vi "VIP_Phase_2.vi"() -> ()   [LabVIEW 2024]
uses:
  <vilib>/DAQmx/read.llb/DAQmx Read (Digital 1D Bool 1Chan 1Samp).vi
  <vilib>/Utility/file.llb/Write To Spreadsheet File (DBL).vi
  <vilib>/DAQmx/create/channels.llb/DAQmx Create Channel (DI-Digital Input).vi
  <vilib>/DAQmx/miscellaneous.llb/DAQmx Fill In Error Info.vi
  <vilib>/ptbypt/NI_PtbyPt.lvlib
panel:
  out "4.2":bool
  out "mouse 4.2":cluster{"Y":dbl[], "Y":dbl[]}[](graph)
  out "mouse 4.1":cluster{"Y":dbl[], "Y":dbl[]}[](graph)
  in  "fake 4.2":bool
  in  "fake 4.1":bool
  out "ratio 4.2R":cluster{"Y":dbl[], "Y":dbl[]}[](graph)=[{"Y"=[2.5380001068115234, 12.063000202178955, 24.592000007629395, 36.145999908447266, 48.69600009918213, 58.23899984359741, 67.79099988937378, 81.40899991989136, 91.96199989318848, 99.9980001449585], "Y"=[0.0, 0.0, 0.0, 0.0, 0.0, 0.0, 0.0, 0.0, 0.0, 0.0]}]
  out "ratio 4.1L":cluster{"Y":dbl[], "Y":dbl[]}[](graph)=[{"Y"=[2.5380001068115234, 12.063000202178955, 24.592000007629395, 36.145999908447266, 48.69600009918213, 58.23899984359741, 67.79099988937378, 81.40899991989136, 91.96199989318848, 99.9980001449585], "Y"=[0.0, 0.0, 0.0, 0.0, 0.0, 0.0, 0.0, 0.0, 0.0, 0.0]}]
  out "ratio 4.2R":dbl
  out "ratio 4.1L":dbl
  in  "water dur (ms) 4.2":dbl=11.5
  in  "water port 4.2":tag="Dev1/port2/line0"
  out "Mouse path 4":path=path "C:/Users/Administrator/Documents/LabVIEW Data/a-lick-20140707-145848"
  out "Mouse file 4":string="a-lick-20140707-145848"
  in  "Mouse ID 4":string
  in  "water dur (ms) 4.1":dbl=9.0
  in  "water port 4.1":tag="Dev1/port1/line7"
  in  "free water 4.2":bool
  in  "free water 4.1":bool
  out "4.1":bool
  out "state 4.2":enum16{"waiting", "sound", "ITI"}(ring)=enum."ITI"
  out "state 4.1":enum16{"waiting", "sound", "ITI"}(ring)=enum."ITI"
  out "water # 4.1L":dbl
  out "water # 4.2R":dbl
  out "lick # 4.2R":dbl
  out "lick # 4.1L":dbl
  out "last water 4.2R":dbl
  out "last water 4.1L":dbl
  out "mistake # 4.2R":dbl
  out "mistake # 4.1L":dbl
  out "ratio 3.2R":cluster{"Y":dbl[], "Y":dbl[]}[](graph)=[{"Y"=[2.5380001068115234, 12.063000202178955, 24.592000007629395, 36.145999908447266, 48.69600009918213, 58.23899984359741, 67.79099988937378, 81.40899991989136, 91.96199989318848, 99.9980001449585], "Y"=[0.0, 0.0, 0.0, 0.0, 0.0, 0.0, 0.0, 0.0, 0.0, 0.0]}]
  out "ratio 3.1L":cluster{"Y":dbl[], "Y":dbl[]}[](graph)=[{"Y"=[2.5380001068115234, 12.063000202178955, 24.592000007629395, 36.145999908447266, 48.69600009918213, 58.23899984359741, 67.79099988937378, 81.40899991989136, 91.96199989318848, 99.9980001449585], "Y"=[0.0, 0.0, 0.0, 0.0, 0.0, 0.0, 0.0, 0.0, 0.0, 0.0]}]
  in  "free water 3.2":bool
  in  "free water 3.1":bool
  in  "water dur (ms) 3. 2":dbl=26.0
  in  "water dur (ms) 3.1":dbl=26.0
  out "mouse 3.2":cluster{"Y":dbl[], "Y":dbl[]}[](graph)
  out "mouse 3.1":cluster{"Y":dbl[], "Y":dbl[]}[](graph)
  in  "fake 3.2":bool
  in  "fake 3.1":bool
  out "last water 3.2R":dbl
  out "last water 3.1L":dbl
  out "mistake # 3.2R":dbl
  out "mistake # 3.1L":dbl
  out "water # 3.2R":dbl
  out "water # 3.1L":dbl
  out "lick # 3.2R":dbl
  out "lick # 3.1L":dbl
  out "ratio 3.2R":dbl
  out "ratio 3.1L":dbl
  in  "water port 3.2":tag="Dev1/port1/line6"
  out "3.2":bool
  out "state 3.2":enum16{"waiting", "sound", "ITI"}(ring)=enum."ITI"
  out "state 3.1":enum16{"waiting", "sound", "ITI"}(ring)=enum."ITI"
  out "3.1":bool
  out "Mouse path 3":path=path "C:/Users/Administrator/Documents/LabVIEW Data/a-lick-20140707-145848"
  out "Mouse file 3":string="a-lick-20140707-145848"
  in  "water port 3.1":tag="Dev1/port1/line5"
  in  "Mouse ID 3":string="test_3"
  out "ratio 2.2R":cluster{"Y":dbl[], "Y":dbl[]}[](graph)=[{"Y"=[2.5380001068115234, 12.063000202178955, 24.592000007629395, 36.145999908447266, 48.69600009918213, 58.23899984359741, 67.79099988937378, 81.40899991989136, 91.96199989318848, 99.9980001449585], "Y"=[0.0, 0.0, 0.0, 0.0, 0.0, 0.0, 0.0, 0.0, 0.0, 0.0]}]
  out "ratio 2.1L":cluster{"Y":dbl[], "Y":dbl[]}[](graph)=[{"Y"=[2.5380001068115234, 12.063000202178955, 24.592000007629395, 36.145999908447266, 48.69600009918213, 58.23899984359741, 67.79099988937378, 81.40899991989136, 91.96199989318848, 99.9980001449585], "Y"=[0.0, 0.0, 0.0, 0.0, 0.0, 0.0, 0.0, 0.0, 0.0, 0.0]}]
  out "ratio 1.2R":cluster{"Y":dbl[], "Y":dbl[]}[](graph)=[{"Y"=[2.5380001068115234, 12.063000202178955, 24.592000007629395, 36.145999908447266, 48.69600009918213, 58.23899984359741, 67.79099988937378, 81.40899991989136, 91.96199989318848, 99.9980001449585], "Y"=[0.0, 0.0, 0.0, 0.0, 0.0, 0.0, 0.0, 0.0, 0.0, 0.0]}]
  out "mouse 2.2":cluster{"Y":dbl[], "Y":dbl[]}[](graph)
  out "mouse 2.1":cluster{"Y":dbl[], "Y":dbl[]}[](graph)
  in  "free water 2.2":bool
  in  "free water 2.1":bool
  out "last water 2.2R":dbl
  out "last water 2.1L":dbl
  out "mistake # 2.2R":dbl
  out "mistake # 2.1L":dbl
  out "water # 2.2R":dbl
  out "water # 2.1L":dbl
  out "lick  #  2.2R":dbl
  out "lick  #  2.1L":dbl
  out "2.1":bool
  out "ratio 2.2R":dbl
  out "ratio 2.1L":dbl
  out "2.2":bool
  in  "fake 2.2":bool
  in  "fake 2.1":bool
  out "Mouse path 2":path=path "C:/Users/Administrator/Documents/LabVIEW Data/a-lick-20140707-145848"
  out "Mouse file 2":string="a-lick-20140707-145848"
  in  "Mouse ID 2":string="test_2"
  in  "water dur (ms) 2.2":dbl=26.5
  in  "water dur (ms) 2.1":dbl=35.5
  in  "water port 2.2":tag="Dev1/port1/line4"
  in  "water port 2.1":tag="Dev1/port1/line3"
  out "state 2.2":enum16{"waiting", "sound", "ITI"}(ring)=enum."ITI"
  out "state 2.1":enum16{"waiting", "sound", "ITI"}(ring)=enum."ITI"
  in  "sound port 2":tag="Dev1/ao1"
  out "time (s)":dbl=103.38100004196167
  out "mistake # 1.2R":dbl
  out "mistake # 1.1L":dbl
  in  "water dur (ms) 1.1":dbl=33.0
  in  "water port 1.1":tag="Dev1/port1/line1"
  in  "water dur (ms) 1.2":dbl=25.0
  in  "water port 1.2":tag="Dev1/port1/line2"
  out "1.1":bool
  out "1.2":bool
  out "state 1.2":enum16{"waiting", "sound", "ITI"}(ring)=enum."ITI"
  out "lick # 1.2R":dbl
  out "water # 1.2R":dbl
  in  "fake 1.2":bool
  in  "free water 1.2":bool
  out "mouse 1.2":cluster{"Y":dbl[], "Y":dbl[]}[](graph)
  out "ratio 1.2R":dbl
  out "last water 1.2R":dbl
  out "ratio 1.1L":dbl
  out "ratio 1.1L":cluster{"Y":dbl[], "Y":dbl[]}[](graph)=[{"Y"=[2.5380001068115234, 12.063000202178955, 24.592000007629395, 36.145999908447266, 48.69600009918213, 58.23899984359741, 67.79099988937378, 81.40899991989136, 91.96199989318848, 99.9980001449585], "Y"=[0.0, 0.0, 0.0, 0.0, 0.0, 0.0, 0.0, 0.0, 0.0, 0.0]}]
  in  "free water 1.1":bool
  out "Right Speaker":dbl=5.0
  out "Left Speaker":dbl=5.0
  in  "sound file 2":path=path "C:/Users/cvm-gritton-lab/Documents/Lab View Programs/Lab View Programs/LabVIEW VIs/Tones/New_Phase_2_Sounds/200k_target2.wav"
  in  "ITI max (ms)":dbl=7000.0
  in  "ITI min (ms)":dbl=5000.0
  in  "reaction dur (ms)":dbl=1750.0
  in  "sound dur (ms)":dbl=3000.0
  in  "sound file 1":path=path "C:/Users/cvm-gritton-lab/Documents/Lab View Programs/Lab View Programs/LabVIEW VIs/Tones/New_Phase_2_Sounds/200k_target1.wav"
  in  "sound port 1":tag="Dev1/ao0"
  out "trial state":T1(ring)=enum."ITI"
  out "trial #":dbl=10.0
  out "current sound":dbl=1.0
  out "next sound":dbl[](array[numeric])
  out "Mouse path 1":path=path "C:/Users/Administrator/Documents/LabVIEW Data/a-lick-20140707-145848"
  in  "fake 1.1":bool
  out "mouse 1.1":cluster{"Y":dbl[], "Y":dbl[]}[](graph)
  out "ITI (s)":dbl=6.5
  out "last water 1.1L":dbl
  out "state 1.1":enum16{"waiting", "sound", "ITI"}(ring)=enum."ITI"
  out "water # 1.1L":dbl
  out "lick # 1.1L":dbl
  out "Mouse file 1":string="a-lick-20140707-145848"
  out "data folder":path=path "C:/LabVIEW VIs/LabVIEW data"
  in  "Mouse ID 1":string
  in  "lick port":tag="Dev1/port0/line0:7"
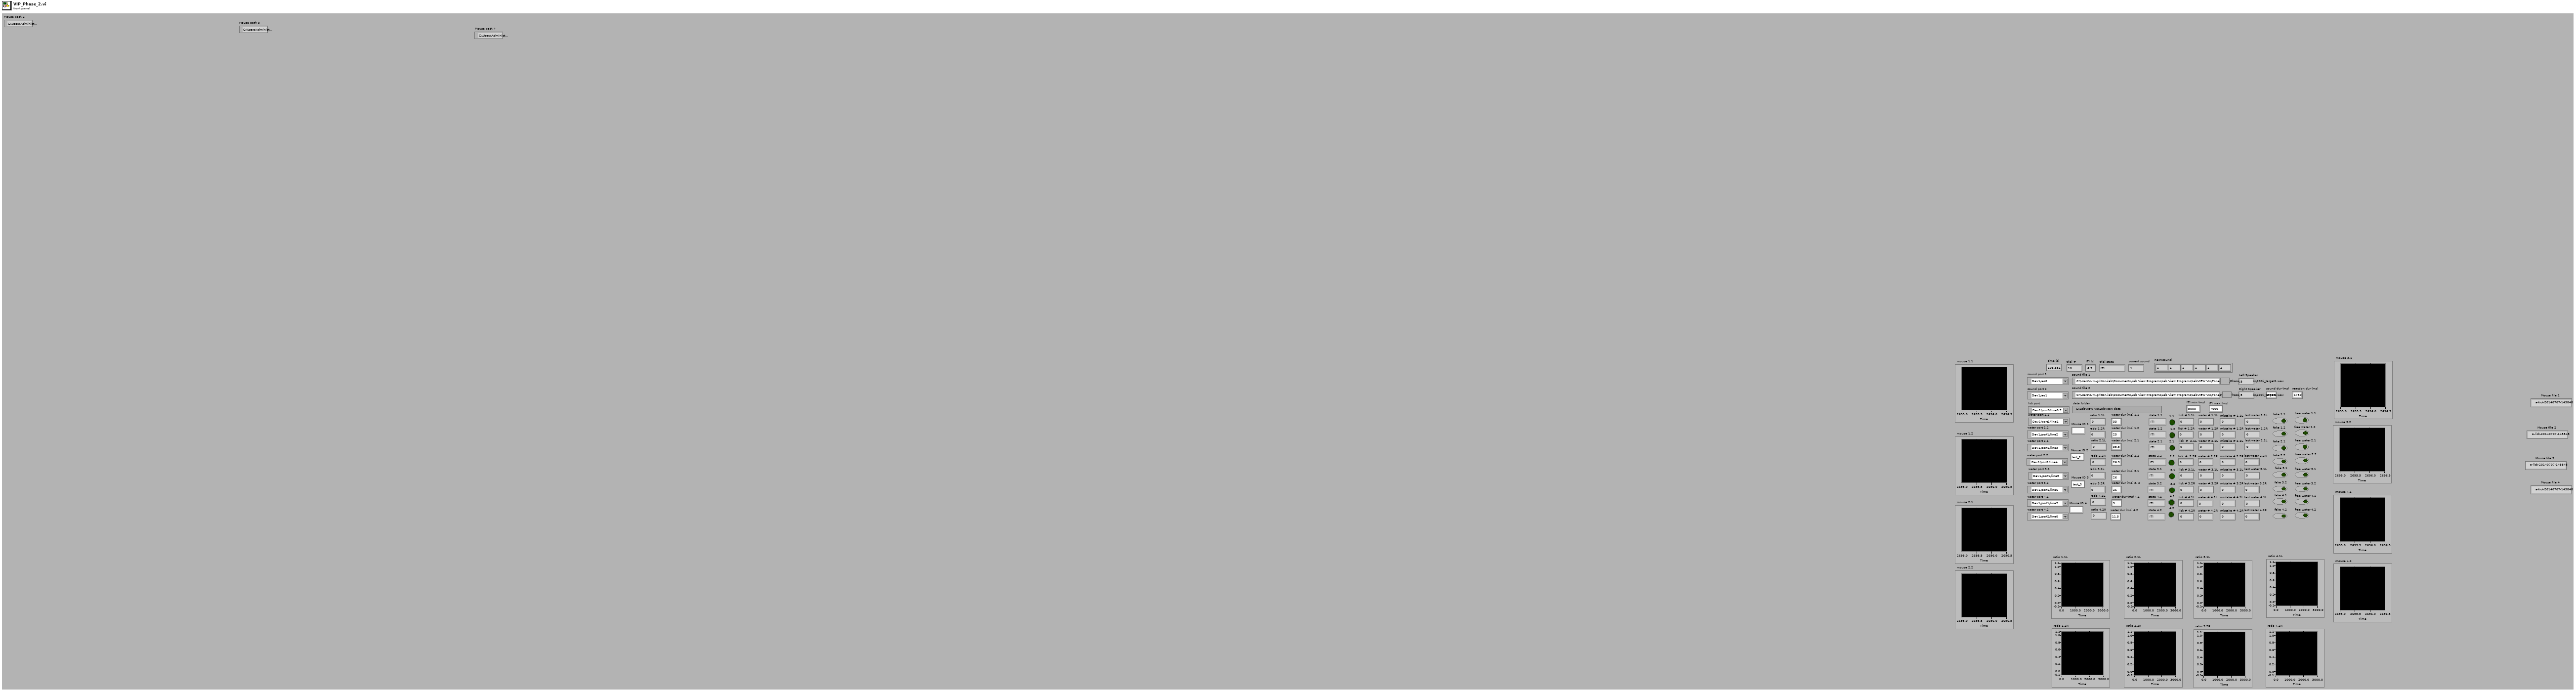
[diagram p1: front panel]
types:
  T1 = enum16{"prepare", "sound", "reaction window", "ITI", "free water", "graph", "data collection"}
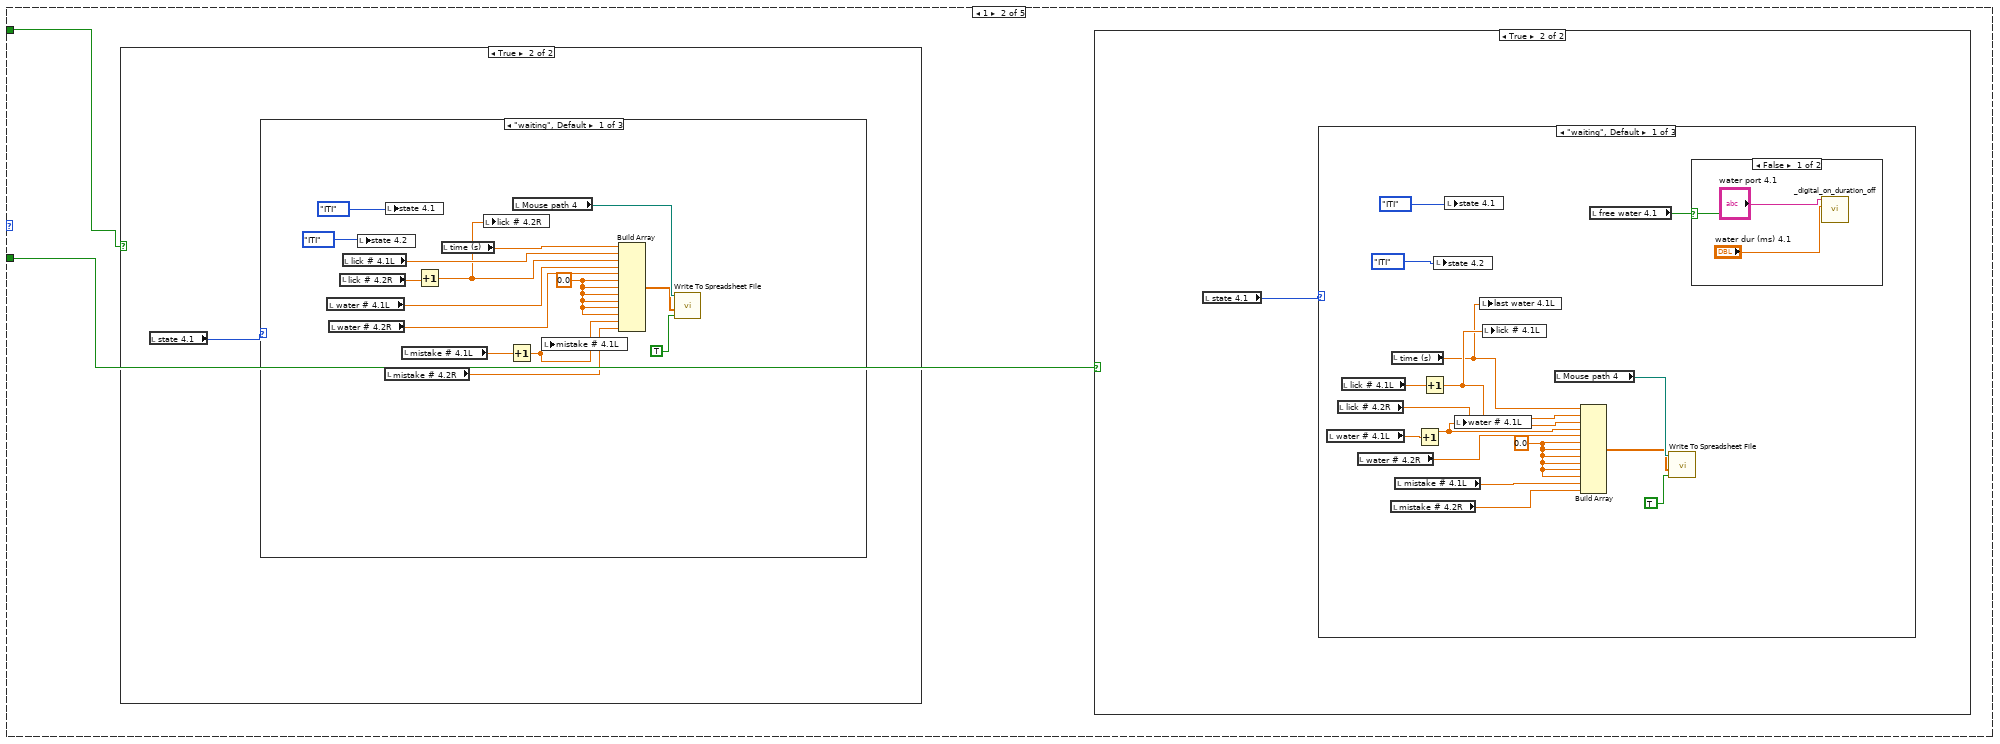
[diagram p3: hidden frame]
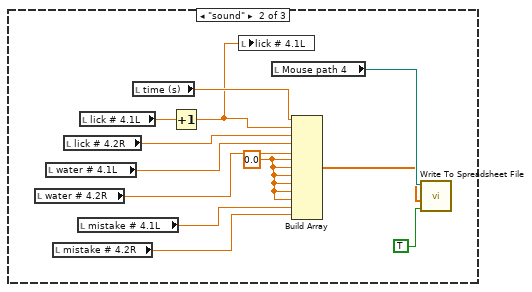
[diagram p6: hidden frame]
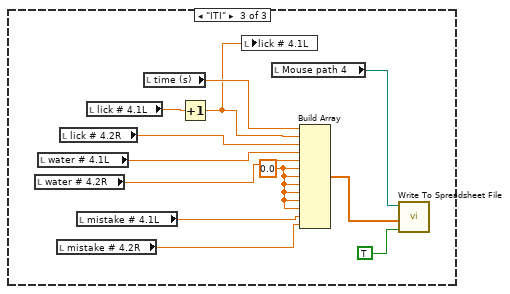
[diagram p7: hidden frame]
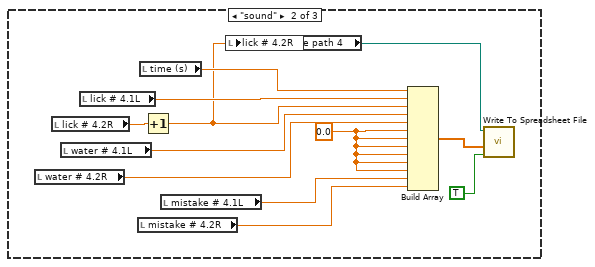
[diagram p9: hidden frame]
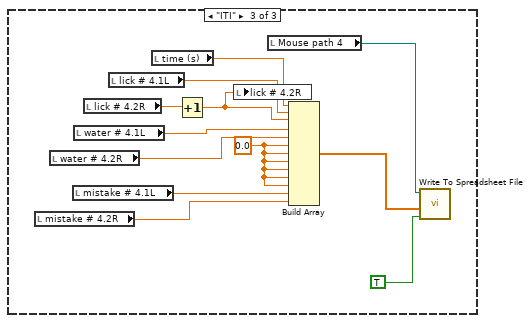
[diagram p10: hidden frame]
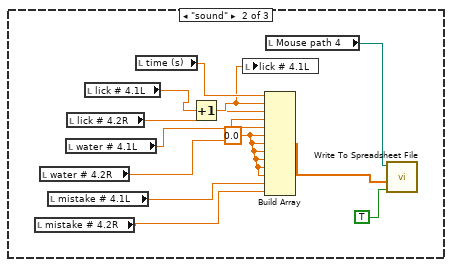
[diagram p12: hidden frame]
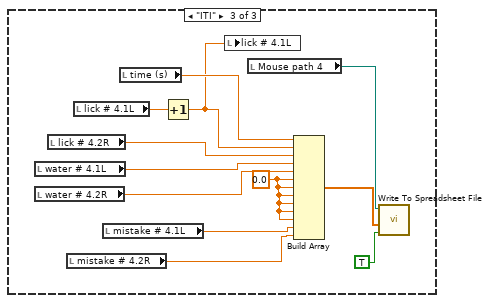
[diagram p13: hidden frame]
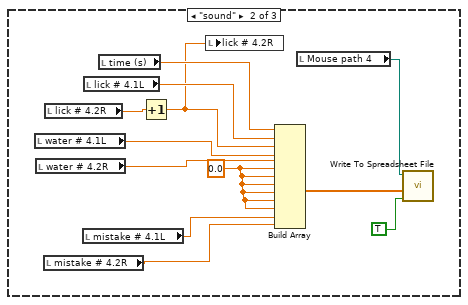
[diagram p16: hidden frame]
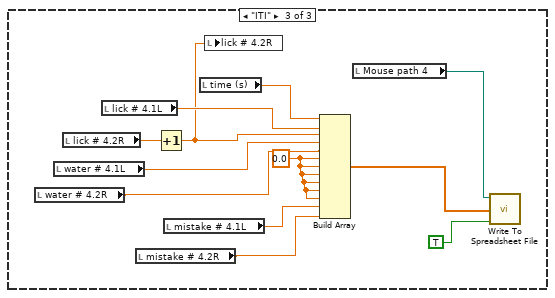
[diagram p17: hidden frame]
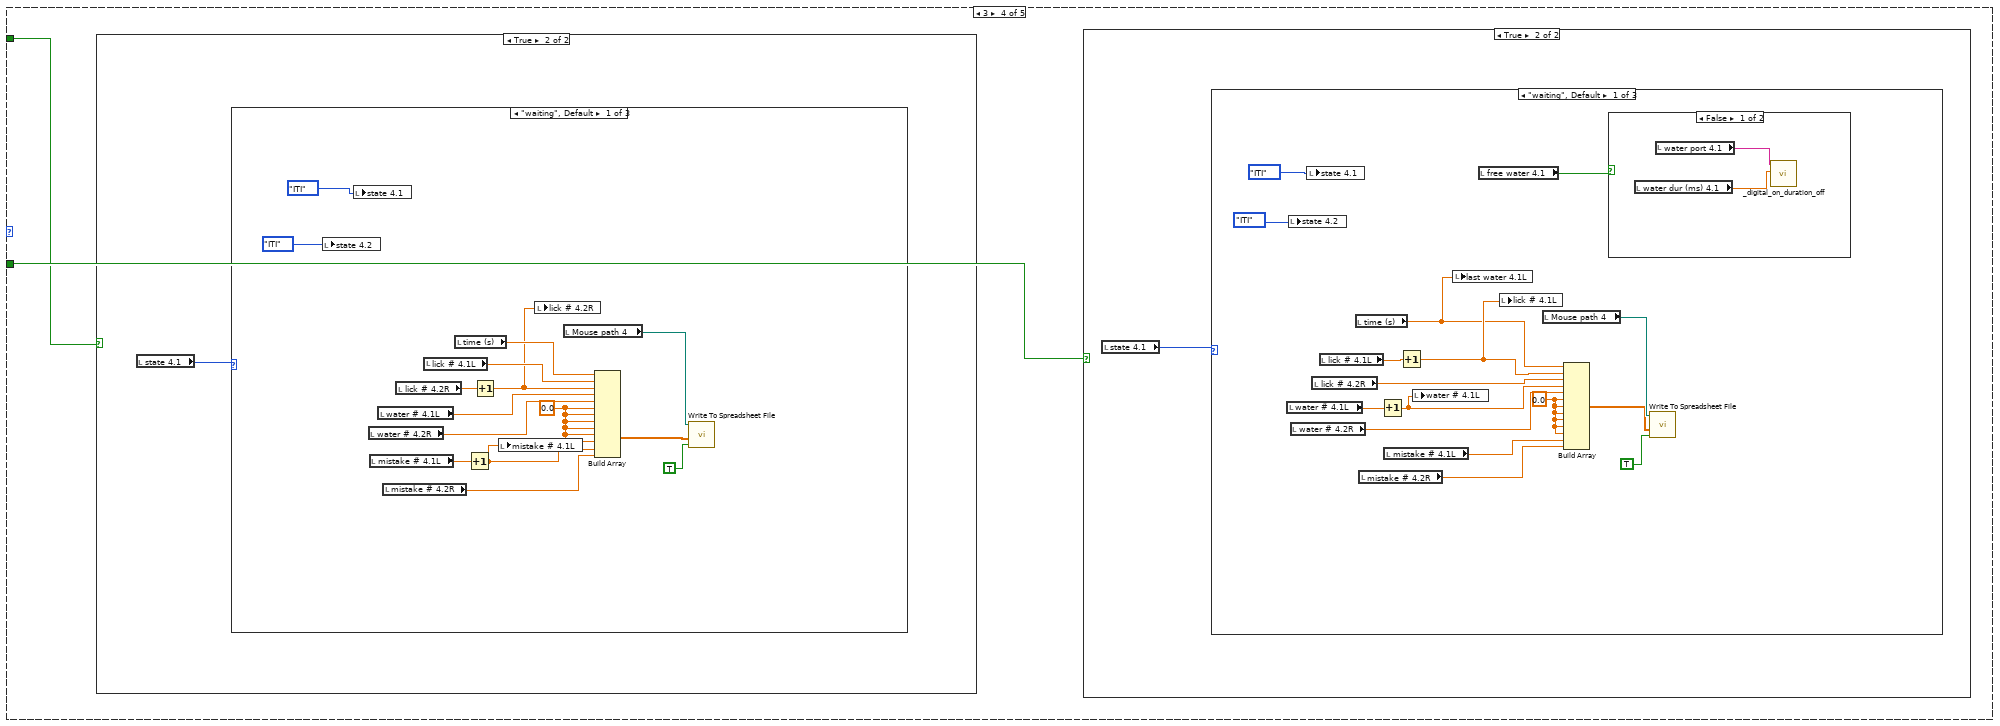
[diagram p18: hidden frame]
diagram:
  n1 = flat-sequence {
    frame #0 {
      w10 = 0.0 ("mistake # 1.1L")
      w2 = 0
      w20 = 0
      w9 = 0
      w1 = 0
      w8 = enum16{"waiting", "sound", "ITI"}."sound"
      n2 = Get Date/Time In Seconds() -> (seconds since 1Jan1904=w22:timestamp)
      n3 = call <vilib>:"Dflt Data Dir.vi"() -> ("App:Default Data Directory"=w4:path)
      "data folder" <- w4
      n4 = Format Date/Time String(time format string (%c)="%m%d%Y-%H%M%S-", seconds (now)=w22) -> (date/time string=w7:string)  [unwired: 1 in]
      n5 = Concatenate Strings(w7, "Mouse ID 1") -> (w25:string)
      "Mouse file 1" <- w25
      n6 = Concatenate Strings(w7, "Mouse ID 4") -> (w5:string)
      "Mouse file 4" <- w5
      n7 = Concatenate Strings(w7, "Mouse ID 2") -> (w15:string)
      "Mouse file 2" <- w15
      n8 = Concatenate Strings(w7, "Mouse ID 3") -> (w12:string)
      "Mouse file 3" <- w12
      n9 = Build Path(base path=w4, name or relative path=w25) -> (appended path=→"Mouse path 1":path)
      n10 = Build Path(base path=w4, name or relative path=w15) -> (appended path=→"Mouse path 2":path)
      n11 = Build Path(base path=w4, name or relative path=w12) -> (appended path=→"Mouse path 3":path)
      n12 = Build Path(base path=w4, name or relative path=w5) -> (appended path=→"Mouse path 4":path)
      n13 = call "_array_shuffle.vi"("total number"=40, "input array"=i32[] [1, 2, 3, 4, 1, 2, 3, 4]) -> ("output array"=→"next sound":dbl[])  [unwired: 9 in]
      n14 = local write "time (s)"(w20) -> ()
      "water # 1.1L" <- w1
      "lick # 1.1L" <- w1
      "state 1.1" <- w8
      "last water 1.1L" <- w9
      "current sound" <- w20
      "trial #" <- w20
      "ITI (s)" <- w20
      "Left Speaker" <- w20
      "Right Speaker" <- w20
      "ratio 1.1L" <- w2
      "last water 1.2R" <- w9
      "ratio 1.2R" <- w2
      "water # 1.2R" <- w1
      "lick # 1.2R" <- w1
      "state 1.2" <- w8
      "mistake # 1.1L" <- w10
      "mistake # 1.2R" <- w10
      "state 2.1" <- w8
      "state 2.2" <- w8
      "ratio 2.1L" <- w2
      "ratio 2.2R" <- w2
      "lick  #  2.1L" <- w1
      "lick  #  2.2R" <- w1
      "water # 2.1L" <- w1
      "water # 2.2R" <- w1
      "mistake # 2.1L" <- w10
      "mistake # 2.2R" <- w10
      "last water 2.1L" <- w9
      "last water 2.2R" <- w9
      "state 3.1" <- w8
      "state 3.2" <- w8
      "ratio 3.1L" <- w2
      "ratio 3.2R" <- w2
      "lick # 3.1L" <- w1
      "lick # 3.2R" <- w1
      "water # 3.1L" <- w1
      "water # 3.2R" <- w1
      "mistake # 3.1L" <- w10
      "mistake # 3.2R" <- w10
      "last water 3.1L" <- w9
      "last water 3.2R" <- w9
      "mistake # 4.1L" <- w10
      "mistake # 4.2R" <- w10
      "last water 4.1L" <- w9
      "last water 4.2R" <- w9
      "lick # 4.1L" <- w1
      "lick # 4.2R" <- w1
      "water # 4.2R" <- w1
      "water # 4.1L" <- w1
      "state 4.1" <- w8
      "state 4.2" <- w8
      "ratio 4.1L" <- w2
      "ratio 4.2R" <- w2
    }
    frame #1 {
      # "file format:\n1. time stamp\n2. lick #\n3. water #\n4. water triggered by lick?\n5. trial start?\n6. trial #\n7. trial sound\n8. trial ITI\n9. free water?"
      n15 = call-poly <vilib>:"DAQmx Create Virtual Channel.vi"("lines"="lick port") -> ("task out"=w27:refnum<k21>)  [unwired: 13 in, 1 out]
      n16 = call <vilib>:"DAQmx Start Task.vi"("task/channels in"=w27) -> ("task out"=w28:refnum<k21>)  [unwired: 13 in, 1 out]
      n17 = while {
        tunnel: w28 -> [w87]
        tunnel: [w86] -> w29
        shift-right: [w77] -> _
        shift-left: _ -> [w85]
        shift-right: [w82] -> _
        shift-left: _ -> [w83]
        stop <- FALSE stop-if-true
        n18 = call-poly <vilib>:"DAQmx Read.vi"("task/channels in"=w87) -> ("task out"=w86:refnum<k21>, "data"=w78:bool[])  [unwired: 12 in, 1 out]
        n19 = Build Array("fake 1.1", "fake 1.2", "fake 2.1", "fake 2.2", "fake 3.1", "fake 3.2", "fake 4.1", "fake 4.2") -> (w74:bool[])
        n20 = Or(x=w78, y=w74) -> (x .or. y?=w77:bool[])
        n21 = Index Array(array=w77) -> (element #1=w80:bool, element #2=w66:bool, element #3=w57:bool, element #4=w54:bool, element #5=w46:bool, element #6=w43:bool, element #7=w38:bool, element #8=w34:bool)  [unwired: 8 in]
        n22 = call "Collector1."("Signals"=w57) -> ("Collected Signals"=w58:dynamicdata)  [unwired: 9 in, 1 out]
        n23 = call "Collector1.2"("Signals"=w66) -> ("Collected Signals"=w65:dynamicdata)  [unwired: 9 in, 1 out]
        n24 = call "Collector1.7"("Signals"=w34) -> ("Collected Signals"=w36:dynamicdata)  [unwired: 9 in, 1 out]
        n25 = call "Collector1.3"("Signals"=w54) -> ("Collected Signals"=w55:dynamicdata)  [unwired: 9 in, 1 out]
        n26 = call "Collector1.6"("Signals"=w38) -> ("Collected Signals"=w39:dynamicdata)  [unwired: 9 in, 1 out]
        n27 = call "Collector1.1"("Signals"=w80) -> ("Collected Signals"=w67:dynamicdata)  [unwired: 9 in, 1 out]
        n28 = call "Collector1.5"("Signals"=w43) -> ("Collected Signals"=w44:dynamicdata)  [unwired: 9 in, 1 out]
        n29 = call "Collector1.4"("Signals"=w46) -> ("Collected Signals"=w47:dynamicdata)  [unwired: 9 in, 1 out]
        n30 = local read "time (s)"() -> (w81:dbl)
        n31 = call "Collector"("Signals"=w81) -> ("Collected Signals"=w33:dynamicdata)  [unwired: 9 in, 1 out]
        n32 = call "Build XY Graph1.1"("Y Input"=w67, "X Input"=w33) -> ("XY Graph"=→"mouse 1.1":cluster{"Y":dbl[], "Y":dbl[]}[])  [unwired: 3 in, 6 out]
        n33 = call "Build XY Graph1."("Y Input"=w58, "X Input"=w33) -> ("XY Graph"=→"mouse 2.1":cluster{"Y":dbl[], "Y":dbl[]}[])  [unwired: 3 in, 6 out]
        n34 = call "Build XY Graph1.2"("Y Input"=w65, "X Input"=w33) -> ("XY Graph"=→"mouse 1.2":cluster{"Y":dbl[], "Y":dbl[]}[])  [unwired: 3 in, 6 out]
        n35 = call "Build XY Graph1.7"("Y Input"=w36, "X Input"=w33) -> ("XY Graph"=→"mouse 4.2":cluster{"Y":dbl[], "Y":dbl[]}[])  [unwired: 3 in, 6 out]
        n36 = call "Build XY Graph1.3"("Y Input"=w55, "X Input"=w33) -> ("XY Graph"=→"mouse 2.2":cluster{"Y":dbl[], "Y":dbl[]}[])  [unwired: 3 in, 6 out]
        n37 = call "Build XY Graph1.6"("Y Input"=w39, "X Input"=w33) -> ("XY Graph"=→"mouse 4.1":cluster{"Y":dbl[], "Y":dbl[]}[])  [unwired: 3 in, 6 out]
        n38 = call "Build XY Graph1.5"("Y Input"=w44, "X Input"=w33) -> ("XY Graph"=→"mouse 3.2":cluster{"Y":dbl[], "Y":dbl[]}[])  [unwired: 3 in, 6 out]
        n39 = call "Build XY Graph1.4"("Y Input"=w47, "X Input"=w33) -> ("XY Graph"=→"mouse 3.1":cluster{"Y":dbl[], "Y":dbl[]}[])  [unwired: 3 in, 6 out]
        n40 = Greater?(x=w77, y=w85) -> (0:w84:bool[])
        n41 = Index Array(array=w84) -> (element #1=w72:bool, element #2=w71:bool, element #3=w60:bool, element #4=w61:bool, element #5=w52:bool, element #6=w51:bool, element #7=w31:bool, element #8=w32:bool)  [unwired: 8 in]
        "1.2" <- w71
        "1.1" <- w72
        "2.2" <- w61
        "2.1" <- w60
        "3.1" <- w52
        "3.2" <- w51
        "4.1" <- w31
        "4.2" <- w32
        n42 = local read "current sound"() -> (w70:dbl)
        n43 = local read "current sound"() -> (w64:dbl)
        n44 = local read "current sound"() -> (w42:dbl)
        n45 = local read "current sound"() -> (w53:dbl)
        n46 = case shown="1" w53 {
          tunnel: w52 -> [_ w429 w514 w599 w684]
          tunnel: w51 -> [_ w428 w513 w598 w683]
          frame 0, Default {
          }
          frame 1 {
            n47 = case shown="True" w429 {
              frame False {
              }
              frame True {
                n48 = local read "state 3.1"() -> (w470:enum16{"waiting", "sound", "ITI"})
                n49 = case shown="\"waiting\", Default" w470 {
                  frame "waiting", Default {
                    w475 = 0.0 ("element")
                    n50 = local write "state 3.2"(enum16{"waiting", "sound", "ITI"}."ITI") -> ()
                    n51 = local read "free water 3.1"() -> (w486:bool)
                    n52 = local write "state 3.1"(enum16{"waiting", "sound", "ITI"}."ITI") -> ()
                    n53 = local read "water # 3.1L"() -> (w478:dbl)
                    n54 = local read "lick # 3.2R"() -> (w479:dbl)
                    n55 = local read "lick # 3.1L"() -> (w481:dbl)
                    n56 = local read "water # 3.2R"() -> (w476:dbl)
                    n57 = case shown="False" w486 {
                      frame False {
                        n58 = call "_digital_on_duration_off.vi"("duration (ms)"="water dur (ms) 3.1", "digital port"="water port 3.1") -> ()  [unwired: 10 in]
                      }
                      frame True {
                      }
                    }
                    n59 = local read "mistake # 3.2R"() -> (w473:dbl)
                    n60 = local read "mistake # 3.1L"() -> (w474:dbl)
                    n61 = Increment(x=w478) -> (x+1=w477:dbl)
                    n62 = Increment(x=w481) -> (x+1=w480:dbl)
                    n63 = local read "time (s)"() -> (w482:dbl)
                    n64 = local write "water # 3.1L"(w477) -> ()
                    n65 = local write "lick # 3.1L"(w480) -> ()
                    n66 = local write "last water 3.1L"(w482) -> ()
                    n67 = local read "Mouse path 3"() -> (w485:path)
                    n68 = Build Array(w482, w480, w479, w477, w476, w475, w475, w475, w475, w475, w475, w474, w473) -> (w483:dbl[])
                    n69 = call-poly <vilib>:"Write To Spreadsheet File.vi"("append to file? (new file:F)"=TRUE, "1D data"=w483, "file path (dialog if empty)"=w485) -> ()  [unwired: 5 in, 1 out]
                  }
                  frame "sound" {
                    w491 = 0.0 ("element")
                    n70 = local read "water # 3.2R"() -> (w492:dbl)
                    n71 = local read "water # 3.1L"() -> (w493:dbl)
                    n72 = local read "lick # 3.2R"() -> (w494:dbl)
                    n73 = local read "mistake # 3.2R"() -> (w489:dbl)
                    n74 = local read "lick # 3.1L"() -> (w496:dbl)
                    n75 = local read "mistake # 3.1L"() -> (w490:dbl)
                    n76 = local read "time (s)"() -> (w497:dbl)
                    n77 = Increment(x=w496) -> (x+1=w495:dbl)
                    n78 = local write "lick # 3.1L"(w495) -> ()
                    n79 = local read "Mouse path 3"() -> (w500:path)
                    n80 = Build Array(w497, w495, w494, w493, w492, w491, w491, w491, w491, w491, w491, w490, w489) -> (w498:dbl[])
                    n81 = call-poly <vilib>:"Write To Spreadsheet File.vi"("append to file? (new file:F)"=TRUE, "1D data"=w498, "file path (dialog if empty)"=w500) -> ()  [unwired: 5 in, 1 out]
                  }
                  frame "ITI" {
                    w503 = 0.0 ("element")
                    n82 = local read "water # 3.2R"() -> (w504:dbl)
                    n83 = local read "lick # 3.2R"() -> (w506:dbl)
                    n84 = local read "lick # 3.1L"() -> (w508:dbl)
                    n85 = local read "water # 3.1L"() -> (w505:dbl)
                    n86 = local read "time (s)"() -> (w509:dbl)
                    n87 = Increment(x=w508) -> (x+1=w507:dbl)
                    n88 = local read "mistake # 3.1L"() -> (w502:dbl)
                    n89 = local read "mistake # 3.2R"() -> (w501:dbl)
                    n90 = local write "lick # 3.1L"(w507) -> ()
                    n91 = local read "Mouse path 3"() -> (w512:path)
                    n92 = Build Array(w509, w507, w506, w505, w504, w503, w503, w503, w503, w503, w503, w502, w501) -> (w510:dbl[])
                    n93 = call-poly <vilib>:"Write To Spreadsheet File.vi"("append to file? (new file:F)"=TRUE, "1D data"=w510, "file path (dialog if empty)"=w512) -> ()  [unwired: 5 in, 1 out]
                  }
                }
              }
            }
            n94 = case shown="True" w428 {
              frame False {
              }
              frame True {
                n95 = local read "state 3.1"() -> (w430:enum16{"waiting", "sound", "ITI"})
                n96 = case shown="\"waiting\", Default" w430 {
                  frame "waiting", Default {
                    w434 = 0.0 ("element")
                    n97 = local write "state 3.2"(enum16{"waiting", "sound", "ITI"}."ITI") -> ()
                    n98 = local write "state 3.1"(enum16{"waiting", "sound", "ITI"}."ITI") -> ()
                    n99 = local read "water # 3.2R"() -> (w435:dbl)
                    n100 = local read "water # 3.1L"() -> (w436:dbl)
                    n101 = local read "lick # 3.2R"() -> (w438:dbl)
                    n102 = local read "mistake # 3.1L"() -> (w433:dbl)
                    n103 = local read "lick # 3.1L"() -> (w439:dbl)
                    n104 = local read "mistake # 3.2R"() -> (w431:dbl)
                    n105 = local read "time (s)"() -> (w440:dbl)
                    n106 = Increment(x=w438) -> (x+1=w437:dbl)
                    n107 = local write "lick # 3.2R"(w437) -> ()
                    n108 = Increment(x=w433) -> (x+1=w432:dbl)
                    n109 = local write "mistake # 3.1L"(w432) -> ()
                    n110 = Build Array(w440, w439, w437, w436, w435, w434, w434, w434, w434, w434, w434, w432, w431) -> (w441:dbl[])
                    n111 = local read "Mouse path 3"() -> (w443:path)
                    n112 = call-poly <vilib>:"Write To Spreadsheet File.vi"("append to file? (new file:F)"=TRUE, "1D data"=w441, "file path (dialog if empty)"=w443) -> ()  [unwired: 5 in, 1 out]
                  }
                  frame "sound" {
                    w448 = 0.0 ("element")
                    n113 = local read "water # 3.1L"() -> (w450:dbl)
                    n114 = local read "lick # 3.2R"() -> (w452:dbl)
                    n115 = local read "water # 3.2R"() -> (w449:dbl)
                    n116 = local read "lick # 3.1L"() -> (w453:dbl)
                    n117 = local read "time (s)"() -> (w454:dbl)
                    n118 = Increment(x=w452) -> (x+1=w451:dbl)
                    n119 = local read "mistake # 3.2R"() -> (w446:dbl)
                    n120 = local read "mistake # 3.1L"() -> (w447:dbl)
                    n121 = local write "lick # 3.2R"(w451) -> ()
                    n122 = local read "Mouse path 3"() -> (w456:path)
                    n123 = Build Array(w454, w453, w451, w450, w449, w448, w448, w448, w448, w448, w448, w447, w446) -> (w455:dbl[])
                    n124 = call-poly <vilib>:"Write To Spreadsheet File.vi"("append to file? (new file:F)"=TRUE, "1D data"=w455, "file path (dialog if empty)"=w456) -> ()  [unwired: 5 in, 1 out]
                  }
                  frame "ITI" {
                    w460 = 0.0 ("element")
                    n125 = local read "water # 3.2R"() -> (w461:dbl)
                    n126 = local read "water # 3.1L"() -> (w462:dbl)
                    n127 = local read "lick # 3.2R"() -> (w464:dbl)
                    n128 = local read "lick # 3.1L"() -> (w465:dbl)
                    n129 = Increment(x=w464) -> (x+1=w463:dbl)
                    n130 = local read "time (s)"() -> (w466:dbl)
                    n131 = local read "mistake # 3.2R"() -> (w458:dbl)
                    n132 = local read "mistake # 3.1L"() -> (w459:dbl)
                    n133 = local write "lick # 3.2R"(w463) -> ()
                    n134 = local read "Mouse path 3"() -> (w468:path)
                    n135 = Build Array(w466, w465, w463, w462, w461, w460, w460, w460, w460, w460, w460, w459, w458) -> (w467:dbl[])
                    n136 = call-poly <vilib>:"Write To Spreadsheet File.vi"("append to file? (new file:F)"=TRUE, "1D data"=w467, "file path (dialog if empty)"=w468) -> ()  [unwired: 5 in, 1 out]
                  }
                }
              }
            }
          }
          frame 2 {
            n137 = case shown="True" w514 {
              frame False {
              }
              frame True {
                n138 = local read "state 3.2"() -> (w558:enum16{"waiting", "sound", "ITI"})
                n139 = case shown="\"waiting\", Default" w558 {
                  frame "waiting", Default {
                    w562 = 0.0 ("element")
                    n140 = local read "water # 3.2R"() -> (w563:dbl)
                    n141 = local read "water # 3.1L"() -> (w564:dbl)
                    n142 = local read "lick # 3.2R"() -> (w565:dbl)
                    n143 = local read "lick # 3.1L"() -> (w567:dbl)
                    n144 = local write "state 3.2"(enum16{"waiting", "sound", "ITI"}."ITI") -> ()
                    n145 = local read "time (s)"() -> (w568:dbl)
                    n146 = local write "state 3.1"(enum16{"waiting", "sound", "ITI"}."ITI") -> ()
                    n147 = local read "mistake # 3.1L"() -> (w561:dbl)
                    n148 = local read "mistake # 3.2R"() -> (w560:dbl)
                    n149 = Increment(x=w567) -> (x+1=w566:dbl)
                    n150 = local write "lick # 3.1L"(w566) -> ()
                    n151 = local read "Mouse path 3"() -> (w570:path)
                    n152 = Increment(x=w560) -> (x+1=w559:dbl)
                    n153 = local write "mistake # 3.2R"(w559) -> ()
                    n154 = Build Array(w568, w566, w565, w564, w563, w562, w562, w562, w562, w562, w562, w561, w559) -> (w569:dbl[])
                    n155 = call-poly <vilib>:"Write To Spreadsheet File.vi"("append to file? (new file:F)"=TRUE, "1D data"=w569, "file path (dialog if empty)"=w570) -> ()  [unwired: 5 in, 1 out]
                  }
                  frame "sound" {
                    w576 = 0.0 ("element")
                    n156 = local read "water # 3.2R"() -> (w577:dbl)
                    n157 = local read "water # 3.1L"() -> (w578:dbl)
                    n158 = local read "lick # 3.2R"() -> (w579:dbl)
                    n159 = local read "lick # 3.1L"() -> (w581:dbl)
                    n160 = local read "mistake # 3.2R"() -> (w574:dbl)
                    n161 = local read "mistake # 3.1L"() -> (w575:dbl)
                    n162 = local read "time (s)"() -> (w582:dbl)
                    n163 = Increment(x=w581) -> (x+1=w580:dbl)
                    n164 = local write "lick # 3.1L"(w580) -> ()
                    n165 = local read "Mouse path 3"() -> (w584:path)
                    n166 = Build Array(w582, w580, w579, w578, w577, w576, w576, w576, w576, w576, w576, w575, w574) -> (w583:dbl[])
                    n167 = call-poly <vilib>:"Write To Spreadsheet File.vi"("append to file? (new file:F)"=TRUE, "1D data"=w583, "file path (dialog if empty)"=w584) -> ()  [unwired: 5 in, 1 out]
                  }
                  frame "ITI" {
                    w588 = 0.0 ("element")
                    n168 = local read "mistake # 3.2R"() -> (w586:dbl)
                    n169 = local read "mistake # 3.1L"() -> (w587:dbl)
                    n170 = local read "water # 3.2R"() -> (w589:dbl)
                    n171 = local read "water # 3.1L"() -> (w590:dbl)
                    n172 = local read "lick # 3.2R"() -> (w591:dbl)
                    n173 = local read "lick # 3.1L"() -> (w593:dbl)
                    n174 = local read "time (s)"() -> (w594:dbl)
                    n175 = Increment(x=w593) -> (x+1=w592:dbl)
                    n176 = local write "lick # 3.1L"(w592) -> ()
                    n177 = local read "Mouse path 3"() -> (w596:path)
                    n178 = Build Array(w594, w592, w591, w590, w589, w588, w588, w588, w588, w588, w588, w587, w586) -> (w595:dbl[])
                    n179 = call-poly <vilib>:"Write To Spreadsheet File.vi"("append to file? (new file:F)"=TRUE, "1D data"=w595, "file path (dialog if empty)"=w596) -> ()  [unwired: 5 in, 1 out]
                  }
                }
              }
            }
            n180 = case shown="True" w513 {
              frame False {
              }
              frame True {
                n181 = local read "state 3.2"() -> (w515:enum16{"waiting", "sound", "ITI"})
                n182 = case shown="\"waiting\", Default" w515 {
                  frame "waiting", Default {
                    w519 = 0.0 ("element")
                    n183 = local read "water # 3.2R"() -> (w521:dbl)
                    n184 = local read "mistake # 3.2R"() -> (w517:dbl)
                    n185 = local read "lick # 3.2R"() -> (w524:dbl)
                    n186 = local read "water # 3.1L"() -> (w522:dbl)
                    n187 = local read "mistake # 3.1L"() -> (w518:dbl)
                    n188 = local write "state 3.1"(enum16{"waiting", "sound", "ITI"}."ITI") -> ()
                    n189 = local write "state 3.2"(enum16{"waiting", "sound", "ITI"}."ITI") -> ()
                    n190 = local read "lick # 3.1L"() -> (w525:dbl)
                    n191 = local read "time (s)"() -> (w516:dbl)
                    n192 = Increment(x=w521) -> (x+1=w520:dbl)
                    n193 = Increment(x=w524) -> (x+1=w523:dbl)
                    n194 = local read "free water 3.2"() -> (w531:bool)
                    n195 = local write "water # 3.2R"(w520) -> ()
                    n196 = local write "last water 3.2R"(w516) -> ()
                    n197 = local write "lick # 3.2R"(w523) -> ()
                    n198 = local read "Mouse path 3"() -> (w527:path)
                    n199 = Build Array(w516, w525, w523, w522, w520, w519, w519, w519, w519, w519, w519, w518, w517) -> (w526:dbl[])
                    n200 = case shown="False" w531 {
                      frame False {
                        n201 = call "_digital_on_duration_off.vi"("duration (ms)"="water dur (ms) 3. 2", "digital port"="water port 3.2") -> ()  [unwired: 10 in]
                      }
                      frame True {
                      }
                    }
                    n202 = call-poly <vilib>:"Write To Spreadsheet File.vi"("append to file? (new file:F)"=TRUE, "1D data"=w526, "file path (dialog if empty)"=w527) -> ()  [unwired: 5 in, 1 out]
                  }
                  frame "sound" {
                    w536 = 0.0 ("element")
                    n203 = local read "lick # 3.2R"() -> (w540:dbl)
                    n204 = local read "water # 3.1L"() -> (w538:dbl)
                    n205 = local read "water # 3.2R"() -> (w537:dbl)
                    n206 = local read "lick # 3.1L"() -> (w541:dbl)
                    n207 = local read "mistake # 3.2R"() -> (w534:dbl)
                    n208 = local read "mistake # 3.1L"() -> (w535:dbl)
                    n209 = Increment(x=w540) -> (x+1=w539:dbl)
                    n210 = local read "time (s)"() -> (w542:dbl)
                    n211 = local write "lick # 3.2R"(w539) -> ()
                    n212 = local read "Mouse path 3"() -> (w545:path)
                    n213 = Build Array(w542, w541, w539, w538, w537, w536, w536, w536, w536, w536, w536, w535, w534) -> (w543:dbl[])
                    n214 = call-poly <vilib>:"Write To Spreadsheet File.vi"("append to file? (new file:F)"=TRUE, "1D data"=w543, "file path (dialog if empty)"=w545) -> ()  [unwired: 5 in, 1 out]
                  }
                  frame "ITI" {
                    w548 = 0.0 ("element")
                    n215 = local read "water # 3.2R"() -> (w549:dbl)
                    n216 = local read "lick # 3.2R"() -> (w552:dbl)
                    n217 = local read "water # 3.1L"() -> (w550:dbl)
                    n218 = local read "lick # 3.1L"() -> (w553:dbl)
                    n219 = local read "mistake # 3.2R"() -> (w546:dbl)
                    n220 = local read "mistake # 3.1L"() -> (w547:dbl)
                    n221 = local read "time (s)"() -> (w554:dbl)
                    n222 = Increment(x=w552) -> (x+1=w551:dbl)
                    n223 = local write "lick # 3.2R"(w551) -> ()
                    n224 = local read "Mouse path 3"() -> (w556:path)
                    n225 = Build Array(w554, w553, w551, w550, w549, w548, w548, w548, w548, w548, w548, w547, w546) -> (w555:dbl[])
                    n226 = call-poly <vilib>:"Write To Spreadsheet File.vi"("append to file? (new file:F)"=TRUE, "1D data"=w555, "file path (dialog if empty)"=w556) -> ()  [unwired: 5 in, 1 out]
                  }
                }
              }
            }
          }
          frame 3 {
            n227 = case shown="True" w599 {
              frame False {
              }
              frame True {
                n228 = local read "state 3.1"() -> (w640:enum16{"waiting", "sound", "ITI"})
                n229 = case shown="\"waiting\", Default" w640 {
                  frame "waiting", Default {
                    w643 = 0.0 ("element")
                    n230 = local read "water # 3.2R"() -> (w645:dbl)
                    n231 = local read "water # 3.1L"() -> (w647:dbl)
                    n232 = local read "lick # 3.1L"() -> (w650:dbl)
                    n233 = local write "state 3.2"(enum16{"waiting", "sound", "ITI"}."ITI") -> ()
                    n234 = local read "lick # 3.2R"() -> (w648:dbl)
                    n235 = local write "state 3.1"(enum16{"waiting", "sound", "ITI"}."ITI") -> ()
                    n236 = local read "time (s)"() -> (w644:dbl)
                    n237 = Increment(x=w650) -> (x+1=w649:dbl)
                    n238 = Increment(x=w647) -> (x+1=w646:dbl)
                    n239 = local read "mistake # 3.2R"() -> (w641:dbl)
                    n240 = local read "mistake # 3.1L"() -> (w642:dbl)
                    n241 = local read "free water 3.1"() -> (w654:bool)
                    n242 = local write "water # 3.1L"(w646) -> ()
                    n243 = local write "lick # 3.1L"(w649) -> ()
                    n244 = local write "last water 3.1L"(w644) -> ()
                    n245 = local read "Mouse path 3"() -> (w653:path)
                    n246 = case shown="False" w654 {
                      frame False {
                        n247 = local read "water dur (ms) 3.1"() -> (w657:dbl)
                        n248 = local read "water port 3.1"() -> (w658:tag)
                        n249 = call "_digital_on_duration_off.vi"("duration (ms)"=w657, "digital port"=w658) -> ()  [unwired: 10 in]
                      }
                      frame True {
                      }
                    }
                    n250 = Build Array(w644, w649, w648, w646, w645, w643, w643, w643, w643, w643, w643, w642, w641) -> (w651:dbl[])
                    n251 = call-poly <vilib>:"Write To Spreadsheet File.vi"("append to file? (new file:F)"=TRUE, "1D data"=w651, "file path (dialog if empty)"=w653) -> ()  [unwired: 5 in, 1 out]
                  }
                  frame "sound" {
                    w661 = 0.0 ("element")
                    n252 = local read "lick # 3.2R"() -> (w664:dbl)
                    n253 = local read "water # 3.2R"() -> (w662:dbl)
                    n254 = local read "water # 3.1L"() -> (w663:dbl)
                    n255 = local read "lick # 3.1L"() -> (w666:dbl)
                    n256 = local read "mistake # 3.2R"() -> (w659:dbl)
                    n257 = local read "mistake # 3.1L"() -> (w660:dbl)
                    n258 = Increment(x=w666) -> (x+1=w665:dbl)
                    n259 = local read "time (s)"() -> (w667:dbl)
                    n260 = local write "lick # 3.1L"(w665) -> ()
                    n261 = local read "Mouse path 3"() -> (w669:path)
                    n262 = Build Array(w667, w665, w664, w663, w662, w661, w661, w661, w661, w661, w661, w660, w659) -> (w668:dbl[])
                    n263 = call-poly <vilib>:"Write To Spreadsheet File.vi"("append to file? (new file:F)"=TRUE, "1D data"=w668, "file path (dialog if empty)"=w669) -> ()  [unwired: 5 in, 1 out]
                  }
                  frame "ITI" {
                    w673 = 0.0 ("element")
                    n264 = local read "water # 3.2R"() -> (w674:dbl)
                    n265 = local read "water # 3.1L"() -> (w675:dbl)
                    n266 = local read "lick # 3.2R"() -> (w676:dbl)
                    n267 = local read "lick # 3.1L"() -> (w678:dbl)
                    n268 = local read "mistake # 3.2R"() -> (w671:dbl)
                    n269 = local read "mistake # 3.1L"() -> (w672:dbl)
                    n270 = local read "time (s)"() -> (w679:dbl)
                    n271 = Increment(x=w678) -> (x+1=w677:dbl)
                    n272 = local write "lick # 3.1L"(w677) -> ()
                    n273 = local read "Mouse path 3"() -> (w681:path)
                    n274 = Build Array(w679, w677, w676, w675, w674, w673, w673, w673, w673, w673, w673, w672, w671) -> (w680:dbl[])
                    n275 = call-poly <vilib>:"Write To Spreadsheet File.vi"("append to file? (new file:F)"=TRUE, "1D data"=w680, "file path (dialog if empty)"=w681) -> ()  [unwired: 5 in, 1 out]
                  }
                }
              }
            }
            n276 = case shown="True" w598 {
              frame False {
              }
              frame True {
                n277 = local read "state 3.1"() -> (w600:enum16{"waiting", "sound", "ITI"})
                n278 = case shown="\"ITI\"" w600 {
                  frame "waiting", Default {
                    w604 = 0.0 ("element")
                    n279 = local write "state 3.2"(enum16{"waiting", "sound", "ITI"}."ITI") -> ()
                    n280 = local write "state 3.1"(enum16{"waiting", "sound", "ITI"}."ITI") -> ()
                    n281 = local read "lick # 3.2R"() -> (w608:dbl)
                    n282 = local read "water # 3.2R"() -> (w605:dbl)
                    n283 = local read "water # 3.1L"() -> (w606:dbl)
                    n284 = local read "lick # 3.1L"() -> (w609:dbl)
                    n285 = local read "mistake # 3.1L"() -> (w603:dbl)
                    n286 = local read "mistake # 3.2R"() -> (w601:dbl)
                    n287 = local read "time (s)"() -> (w610:dbl)
                    n288 = Increment(x=w608) -> (x+1=w607:dbl)
                    n289 = local write "lick # 3.2R"(w607) -> ()
                    n290 = Increment(x=w603) -> (x+1=w602:dbl)
                    n291 = local write "mistake # 3.1L"(w602) -> ()
                    n292 = local read "Mouse path 3"() -> (w611:path)
                    n293 = Build Array(w610, w609, w607, w606, w605, w604, w604, w604, w604, w604, w604, w602, w601) -> (w612:dbl[])
                    n294 = call-poly <vilib>:"Write To Spreadsheet File.vi"("append to file? (new file:F)"=TRUE, "1D data"=w612, "file path (dialog if empty)"=w611) -> ()  [unwired: 5 in, 1 out]
                  }
                  frame "sound" {
                    w618 = 0.0 ("element")
                    n295 = local read "water # 3.2R"() -> (w619:dbl)
                    n296 = local read "water # 3.1L"() -> (w620:dbl)
                    n297 = local read "mistake # 3.2R"() -> (w616:dbl)
                    n298 = local read "lick # 3.2R"() -> (w622:dbl)
                    n299 = local read "mistake # 3.1L"() -> (w617:dbl)
                    n300 = local read "lick # 3.1L"() -> (w623:dbl)
                    n301 = local read "time (s)"() -> (w624:dbl)
                    n302 = Increment(x=w622) -> (x+1=w621:dbl)
                    n303 = local read "Mouse path 3"() -> (w626:path)
                    n304 = local write "lick # 3.2R"(w621) -> ()
                    n305 = Build Array(w624, w623, w621, w620, w619, w618, w618, w618, w618, w618, w618, w617, w616) -> (w625:dbl[])
                    n306 = call-poly <vilib>:"Write To Spreadsheet File.vi"("append to file? (new file:F)"=TRUE, "1D data"=w625, "file path (dialog if empty)"=w626) -> ()  [unwired: 5 in, 1 out]
                  }
                  frame "ITI" {
                    w630 = 0.0 ("element")
                    n307 = local read "lick # 3.2R"() -> (w634:dbl)
                    n308 = local read "water # 3.2R"() -> (w631:dbl)
                    n309 = local read "water # 3.1L"() -> (w632:dbl)
                    n310 = local read "lick # 3.1L"() -> (w635:dbl)
                    n311 = local read "mistake # 3.1L"() -> (w629:dbl)
                    n312 = local read "mistake # 3.2R"() -> (w628:dbl)
                    n313 = Increment(x=w634) -> (x+1=w633:dbl)
                    n314 = local read "time (s)"() -> (w636:dbl)
                    n315 = local write "lick # 3.2R"(w633) -> ()
                    n316 = local read "Mouse path 3"() -> (w638:path)
                    n317 = Build Array(w636, w635, w633, w632, w631, w630, w630, w630, w630, w630, w630, w629, w628) -> (w637:dbl[])
                    n318 = call-poly <vilib>:"Write To Spreadsheet File.vi"("append to file? (new file:F)"=TRUE, "1D data"=w637, "file path (dialog if empty)"=w638) -> ()  [unwired: 5 in, 1 out]
                  }
                }
              }
            }
          }
          frame 4 {
            n319 = case shown="True" w684 {
              frame False {
              }
              frame True {
                n320 = local read "state 3.2"() -> (w728:enum16{"waiting", "sound", "ITI"})
                n321 = case shown="\"waiting\", Default" w728 {
                  frame "waiting", Default {
                    w732 = 0.0 ("element")
                    n322 = local read "mistake # 3.2R"() -> (w730:dbl)
                    n323 = local read "mistake # 3.1L"() -> (w731:dbl)
                    n324 = local read "water # 3.2R"() -> (w733:dbl)
                    n325 = local read "water # 3.1L"() -> (w734:dbl)
                    n326 = local read "lick # 3.2R"() -> (w735:dbl)
                    n327 = local read "lick # 3.1L"() -> (w737:dbl)
                    n328 = local write "state 3.2"(enum16{"waiting", "sound", "ITI"}."ITI") -> ()
                    n329 = local write "state 3.1"(enum16{"waiting", "sound", "ITI"}."ITI") -> ()
                    n330 = local read "time (s)"() -> (w738:dbl)
                    n331 = Increment(x=w730) -> (x+1=w729:dbl)
                    n332 = Increment(x=w737) -> (x+1=w736:dbl)
                    n333 = local write "mistake # 3.2R"(w729) -> ()
                    n334 = local write "lick # 3.1L"(w736) -> ()
                    n335 = local read "Mouse path 3"() -> (w740:path)
                    n336 = Build Array(w738, w736, w735, w734, w733, w732, w732, w732, w732, w732, w732, w731, w729) -> (w739:dbl[])
                    n337 = call-poly <vilib>:"Write To Spreadsheet File.vi"("append to file? (new file:F)"=TRUE, "1D data"=w739, "file path (dialog if empty)"=w740) -> ()  [unwired: 5 in, 1 out]
                  }
                  frame "sound" {
                    w746 = 0.0 ("element")
                    n338 = local read "mistake # 3.2R"() -> (w744:dbl)
                    n339 = local read "water # 3.2R"() -> (w747:dbl)
                    n340 = local read "mistake # 3.1L"() -> (w745:dbl)
                    n341 = local read "water # 3.1L"() -> (w748:dbl)
                    n342 = local read "lick # 3.2R"() -> (w749:dbl)
                    n343 = local read "lick # 3.1L"() -> (w751:dbl)
                    n344 = local read "time (s)"() -> (w752:dbl)
                    n345 = Increment(x=w751) -> (x+1=w750:dbl)
                    n346 = local read "Mouse path 3"() -> (w754:path)
                    n347 = local write "lick # 3.1L"(w750) -> ()
                    n348 = Build Array(w752, w750, w749, w748, w747, w746, w746, w746, w746, w746, w746, w745, w744) -> (w753:dbl[])
                    n349 = call-poly <vilib>:"Write To Spreadsheet File.vi"("append to file? (new file:F)"=TRUE, "1D data"=w753, "file path (dialog if empty)"=w754) -> ()  [unwired: 5 in, 1 out]
                  }
                  frame "ITI" {
                    w758 = 0.0 ("element")
                    n350 = local read "water # 3.1L"() -> (w760:dbl)
                    n351 = local read "water # 3.2R"() -> (w759:dbl)
                    n352 = local read "lick # 3.2R"() -> (w761:dbl)
                    n353 = local read "lick # 3.1L"() -> (w763:dbl)
                    n354 = local read "mistake # 3.1L"() -> (w757:dbl)
                    n355 = local read "mistake # 3.2R"() -> (w756:dbl)
                    n356 = local read "time (s)"() -> (w764:dbl)
                    n357 = Increment(x=w763) -> (x+1=w762:dbl)
                    n358 = local write "lick # 3.1L"(w762) -> ()
                    n359 = Build Array(w764, w762, w761, w760, w759, w758, w758, w758, w758, w758, w758, w757, w756) -> (w765:dbl[])
                    n360 = local read "Mouse path 3"() -> (w766:path)
                    n361 = call-poly <vilib>:"Write To Spreadsheet File.vi"("append to file? (new file:F)"=TRUE, "1D data"=w765, "file path (dialog if empty)"=w766) -> ()  [unwired: 5 in, 1 out]
                  }
                }
              }
            }
            n362 = case shown="True" w683 {
              frame False {
              }
              frame True {
                n363 = local read "state 3.2"() -> (w685:enum16{"waiting", "sound", "ITI"})
                n364 = case shown="\"waiting\", Default" w685 {
                  frame "waiting", Default {
                    w690 = 0.0 ("element")
                    n365 = local read "lick # 3.2R"() -> (w695:dbl)
                    n366 = local read "water # 3.2R"() -> (w692:dbl)
                    n367 = local read "water # 3.1L"() -> (w693:dbl)
                    n368 = local read "lick # 3.1L"() -> (w696:dbl)
                    n369 = local read "mistake # 3.1L"() -> (w689:dbl)
                    n370 = local read "mistake # 3.2R"() -> (w688:dbl)
                    n371 = local read "time (s)"() -> (w686:dbl)
                    n372 = Increment(x=w695) -> (x+1=w694:dbl)
                    n373 = Increment(x=w692) -> (x+1=w691:dbl)
                    n374 = local write "water # 3.2R"(w691) -> ()
                    n375 = local write "state 3.2"(enum16{"waiting", "sound", "ITI"}."ITI") -> ()
                    n376 = local write "state 3.1"(enum16{"waiting", "sound", "ITI"}."ITI") -> ()
                    n377 = local write "last water 3.2R"(w686) -> ()
                    n378 = local write "lick # 3.2R"(w694) -> ()
                    n379 = local read "Mouse path 3"() -> (w698:path)
                    n380 = local read "free water 3.2"() -> (w687:bool)
                    n381 = Build Array(w686, w696, w694, w693, w691, w690, w690, w690, w690, w690, w690, w689, w688) -> (w697:dbl[])
                    n382 = call-poly <vilib>:"Write To Spreadsheet File.vi"("append to file? (new file:F)"=TRUE, "1D data"=w697, "file path (dialog if empty)"=w698) -> ()  [unwired: 5 in, 1 out]
                    n383 = case shown="False" w687 {
                      frame False {
                        n384 = local read "water dur (ms) 3. 2"() -> (w703:dbl)
                        n385 = local read "water port 3.2"() -> (w702:tag)
                        n386 = call "_digital_on_duration_off.vi"("duration (ms)"=w703, "digital port"=w702) -> ()  [unwired: 10 in]
                      }
                      frame True {
                      }
                    }
                  }
                  frame "sound" {
                    w706 = 0.0 ("element")
                    n387 = local read "water # 3.2R"() -> (w707:dbl)
                    n388 = local read "water # 3.1L"() -> (w708:dbl)
                    n389 = local read "lick # 3.2R"() -> (w710:dbl)
                    n390 = local read "mistake # 3.2R"() -> (w704:dbl)
                    n391 = local read "lick # 3.1L"() -> (w711:dbl)
                    n392 = local read "mistake # 3.1L"() -> (w705:dbl)
                    n393 = local read "time (s)"() -> (w712:dbl)
                    n394 = Increment(x=w710) -> (x+1=w709:dbl)
                    n395 = local write "lick # 3.2R"(w709) -> ()
                    n396 = local read "Mouse path 3"() -> (w714:path)
                    n397 = Build Array(w712, w711, w709, w708, w707, w706, w706, w706, w706, w706, w706, w705, w704) -> (w713:dbl[])
                    n398 = call-poly <vilib>:"Write To Spreadsheet File.vi"("append to file? (new file:F)"=TRUE, "1D data"=w713, "file path (dialog if empty)"=w714) -> ()  [unwired: 5 in, 1 out]
                  }
                  frame "ITI" {
                    w718 = 0.0 ("element")
                    n399 = local read "water # 3.2R"() -> (w719:dbl)
                    n400 = local read "lick # 3.2R"() -> (w722:dbl)
                    n401 = local read "water # 3.1L"() -> (w720:dbl)
                    n402 = local read "mistake # 3.2R"() -> (w716:dbl)
                    n403 = local read "lick # 3.1L"() -> (w723:dbl)
                    n404 = local read "mistake # 3.1L"() -> (w717:dbl)
                    n405 = local read "time (s)"() -> (w724:dbl)
                    n406 = Increment(x=w722) -> (x+1=w721:dbl)
                    n407 = local write "lick # 3.2R"(w721) -> ()
                    n408 = local read "Mouse path 3"() -> (w726:path)
                    n409 = Build Array(w724, w723, w721, w720, w719, w718, w718, w718, w718, w718, w718, w717, w716) -> (w725:dbl[])
                    n410 = call-poly <vilib>:"Write To Spreadsheet File.vi"("append to file? (new file:F)"=TRUE, "1D data"=w725, "file path (dialog if empty)"=w726) -> ()  [unwired: 5 in, 1 out]
                  }
                }
              }
            }
          }
        }
        n411 = case shown="2" w64 {
          tunnel: w60 -> [_ w769 w854 w939 w1024]
          tunnel: w61 -> [_ w768 w853 w938 w1023]
          frame 0, Default {
          }
          frame 1 {
            n412 = case shown="True" w769 {
              frame False {
              }
              frame True {
                n413 = local read "state 2.1"() -> (w810:enum16{"waiting", "sound", "ITI"})
                n414 = case shown="\"waiting\", Default" w810 {
                  frame "waiting", Default {
                    w815 = 0.0 ("element")
                    n415 = local read "free water 2.1"() -> (w811:bool)
                    n416 = case shown="False" w811 {
                      frame False {
                        n417 = call "_digital_on_duration_off.vi"("duration (ms)"="water dur (ms) 2.1", "digital port"="water port 2.1") -> ()  [unwired: 10 in]
                      }
                      frame True {
                      }
                    }
                    n418 = local write "state 2.2"(enum16{"waiting", "sound", "ITI"}."ITI") -> ()
                    n419 = local write "state 2.1"(enum16{"waiting", "sound", "ITI"}."ITI") -> ()
                    n420 = local read "lick  #  2.1L"() -> (w821:dbl)
                    n421 = local read "water # 2.2R"() -> (w816:dbl)
                    n422 = local read "water # 2.1L"() -> (w818:dbl)
                    n423 = local read "lick  #  2.2R"() -> (w819:dbl)
                    n424 = Increment(x=w821) -> (x+1=w820:dbl)
                    n425 = local read "mistake # 2.2R"() -> (w813:dbl)
                    n426 = local read "mistake # 2.1L"() -> (w814:dbl)
                    n427 = Increment(x=w818) -> (x+1=w817:dbl)
                    n428 = local read "time (s)"() -> (w812:dbl)
                    n429 = local write "lick  #  2.1L"(w820) -> ()
                    n430 = local write "water # 2.1L"(w817) -> ()
                    n431 = local write "last water 2.1L"(w812) -> ()
                    n432 = local read "Mouse path 2"() -> (w824:path)
                    n433 = Build Array(w812, w820, w819, w817, w816, w815, w815, w815, w815, w815, w815, w814, w813) -> (w822:dbl[])
                    n434 = call-poly <vilib>:"Write To Spreadsheet File.vi"("append to file? (new file:F)"=TRUE, "1D data"=w822, "file path (dialog if empty)"=w824) -> ()  [unwired: 5 in, 1 out]
                  }
                  frame "sound" {
                    w831 = 0.0 ("element")
                    n435 = local read "water # 2.2R"() -> (w832:dbl)
                    n436 = local read "water # 2.1L"() -> (w833:dbl)
                    n437 = local read "lick  #  2.2R"() -> (w834:dbl)
                    n438 = local read "lick  #  2.1L"() -> (w836:dbl)
                    n439 = local read "mistake # 2.2R"() -> (w829:dbl)
                    n440 = local read "mistake # 2.1L"() -> (w830:dbl)
                    n441 = local read "time (s)"() -> (w837:dbl)
                    n442 = Increment(x=w836) -> (x+1=w835:dbl)
                    n443 = local write "lick  #  2.1L"(w835) -> ()
                    n444 = local read "Mouse path 2"() -> (w840:path)
                    n445 = Build Array(w837, w835, w834, w833, w832, w831, w831, w831, w831, w831, w831, w830, w829) -> (w838:dbl[])
                    n446 = call-poly <vilib>:"Write To Spreadsheet File.vi"("append to file? (new file:F)"=TRUE, "1D data"=w838, "file path (dialog if empty)"=w840) -> ()  [unwired: 5 in, 1 out]
                  }
                  frame "ITI" {
                    w843 = 0.0 ("element")
                    n447 = local read "water # 2.2R"() -> (w844:dbl)
                    n448 = local read "water # 2.1L"() -> (w845:dbl)
                    n449 = local read "lick  #  2.2R"() -> (w846:dbl)
                    n450 = local read "lick  #  2.1L"() -> (w848:dbl)
                    n451 = local read "time (s)"() -> (w849:dbl)
                    n452 = local read "mistake # 2.2R"() -> (w841:dbl)
                    n453 = local read "mistake # 2.1L"() -> (w842:dbl)
                    n454 = Increment(x=w848) -> (x+1=w847:dbl)
                    n455 = local write "lick  #  2.1L"(w847) -> ()
                    n456 = local read "Mouse path 2"() -> (w851:path)
                    n457 = Build Array(w849, w847, w846, w845, w844, w843, w843, w843, w843, w843, w843, w842, w841) -> (w850:dbl[])
                    n458 = call-poly <vilib>:"Write To Spreadsheet File.vi"("append to file? (new file:F)"=TRUE, "1D data"=w850, "file path (dialog if empty)"=w851) -> ()  [unwired: 5 in, 1 out]
                  }
                }
              }
            }
            n459 = case shown="True" w768 {
              frame False {
              }
              frame True {
                n460 = local read "state 2.1"() -> (w770:enum16{"waiting", "sound", "ITI"})
                n461 = case shown="\"waiting\", Default" w770 {
                  frame "waiting", Default {
                    w774 = 0.0 ("element")
                    n462 = local read "mistake # 2.1L"() -> (w773:dbl)
                    n463 = local read "mistake # 2.2R"() -> (w771:dbl)
                    n464 = local read "water # 2.2R"() -> (w775:dbl)
                    n465 = local read "lick  #  2.2R"() -> (w779:dbl)
                    n466 = local read "water # 2.1L"() -> (w776:dbl)
                    n467 = local read "lick  #  2.1L"() -> (w778:dbl)
                    n468 = local write "state 2.2"(enum16{"waiting", "sound", "ITI"}."ITI") -> ()
                    n469 = local read "time (s)"() -> (w780:dbl)
                    n470 = Increment(x=w779) -> (x+1=w777:dbl)
                    n471 = Increment(x=w773) -> (x+1=w772:dbl)
                    n472 = local write "state 2.1"(enum16{"waiting", "sound", "ITI"}."ITI") -> ()
                    n473 = local write "mistake # 2.1L"(w772) -> ()
                    n474 = local write "lick  #  2.2R"(w777) -> ()
                    n475 = local read "Mouse path 2"() -> (w783:path)
                    n476 = Build Array(w780, w778, w777, w776, w775, w774, w774, w774, w774, w774, w774, w772, w771) -> (w782:dbl[])
                    n477 = call-poly <vilib>:"Write To Spreadsheet File.vi"("append to file? (new file:F)"=TRUE, "1D data"=w782, "file path (dialog if empty)"=w783) -> ()  [unwired: 5 in, 1 out]
                  }
                  frame "ITI" {
                    w788 = 0.0 ("element")
                    n478 = local read "water # 2.2R"() -> (w789:dbl)
                    n479 = local read "lick  #  2.2R"() -> (w792:dbl)
                    n480 = local read "water # 2.1L"() -> (w790:dbl)
                    n481 = local read "lick  #  2.1L"() -> (w793:dbl)
                    n482 = local read "mistake # 2.2R"() -> (w786:dbl)
                    n483 = Increment(x=w792) -> (x+1=w791:dbl)
                    n484 = local read "time (s)"() -> (w794:dbl)
                    n485 = local read "mistake # 2.1L"() -> (w787:dbl)
                    n486 = local write "lick  #  2.2R"(w791) -> ()
                    n487 = local read "Mouse path 2"() -> (w796:path)
                    n488 = Build Array(w794, w793, w791, w790, w789, w788, w788, w788, w788, w788, w788, w787, w786) -> (w795:dbl[])
                    n489 = call-poly <vilib>:"Write To Spreadsheet File.vi"("append to file? (new file:F)"=TRUE, "1D data"=w795, "file path (dialog if empty)"=w796) -> ()  [unwired: 5 in, 1 out]
                  }
                  frame "sound" {
                    w800 = 0.0 ("element")
                    n490 = local read "water # 2.2R"() -> (w801:dbl)
                    n491 = local read "water # 2.1L"() -> (w802:dbl)
                    n492 = local read "lick  #  2.2R"() -> (w804:dbl)
                    n493 = local read "lick  #  2.1L"() -> (w805:dbl)
                    n494 = local read "mistake # 2.2R"() -> (w798:dbl)
                    n495 = local read "mistake # 2.1L"() -> (w799:dbl)
                    n496 = Increment(x=w804) -> (x+1=w803:dbl)
                    n497 = local read "time (s)"() -> (w806:dbl)
                    n498 = local write "lick  #  2.2R"(w803) -> ()
                    n499 = local read "Mouse path 2"() -> (w808:path)
                    n500 = Build Array(w806, w805, w803, w802, w801, w800, w800, w800, w800, w800, w800, w799, w798) -> (w807:dbl[])
                    n501 = call-poly <vilib>:"Write To Spreadsheet File.vi"("append to file? (new file:F)"=TRUE, "1D data"=w807, "file path (dialog if empty)"=w808) -> ()  [unwired: 5 in, 1 out]
                  }
                }
              }
            }
          }
          frame 2 {
            n502 = case shown="True" w854 {
              frame False {
              }
              frame True {
                n503 = local read "state 2.2"() -> (w898:enum16{"waiting", "sound", "ITI"})
                n504 = case shown="\"waiting\", Default" w898 {
                  frame "waiting", Default {
                    w902 = 0.0 ("element")
                    n505 = local write "state 2.2"(enum16{"waiting", "sound", "ITI"}."ITI") -> ()
                    n506 = local write "state 2.1"(enum16{"waiting", "sound", "ITI"}."ITI") -> ()
                    n507 = local read "mistake # 2.2R"() -> (w900:dbl)
                    n508 = local read "water # 2.2R"() -> (w903:dbl)
                    n509 = local read "water # 2.1L"() -> (w904:dbl)
                    n510 = local read "lick  #  2.2R"() -> (w905:dbl)
                    n511 = local read "mistake # 2.1L"() -> (w901:dbl)
                    n512 = local read "lick  #  2.1L"() -> (w907:dbl)
                    n513 = Increment(x=w900) -> (x+1=w899:dbl)
                    n514 = local read "time (s)"() -> (w908:dbl)
                    n515 = Increment(x=w907) -> (x+1=w906:dbl)
                    n516 = local write "mistake # 2.2R"(w899) -> ()
                    n517 = local write "lick  #  2.1L"(w906) -> ()
                    n518 = local read "Mouse path 2"() -> (w910:path)
                    n519 = Build Array(w908, w906, w905, w904, w903, w902, w902, w902, w902, w902, w902, w901, w899) -> (w909:dbl[])
                    n520 = call-poly <vilib>:"Write To Spreadsheet File.vi"("append to file? (new file:F)"=TRUE, "1D data"=w909, "file path (dialog if empty)"=w910) -> ()  [unwired: 5 in, 1 out]
                  }
                  frame "sound" {
                    w916 = 0.0 ("element")
                    n521 = local read "water # 2.2R"() -> (w917:dbl)
                    n522 = local read "water # 2.1L"() -> (w918:dbl)
                    n523 = local read "lick  #  2.2R"() -> (w919:dbl)
                    n524 = local read "mistake # 2.2R"() -> (w914:dbl)
                    n525 = local read "mistake # 2.1L"() -> (w915:dbl)
                    n526 = local read "lick  #  2.1L"() -> (w921:dbl)
                    n527 = Increment(x=w921) -> (x+1=w920:dbl)
                    n528 = local read "time (s)"() -> (w922:dbl)
                    n529 = local write "lick  #  2.1L"(w920) -> ()
                    n530 = local read "Mouse path 2"() -> (w924:path)
                    n531 = Build Array(w922, w920, w919, w918, w917, w916, w916, w916, w916, w916, w916, w915, w914) -> (w923:dbl[])
                    n532 = call-poly <vilib>:"Write To Spreadsheet File.vi"("append to file? (new file:F)"=TRUE, "1D data"=w923, "file path (dialog if empty)"=w924) -> ()  [unwired: 5 in, 1 out]
                  }
                  frame "ITI" {
                    w928 = 0.0 ("element")
                    n533 = local read "water # 2.2R"() -> (w929:dbl)
                    n534 = local read "water # 2.1L"() -> (w930:dbl)
                    n535 = local read "lick  #  2.1L"() -> (w933:dbl)
                    n536 = local read "lick  #  2.2R"() -> (w931:dbl)
                    n537 = local read "time (s)"() -> (w934:dbl)
                    n538 = Increment(x=w933) -> (x+1=w932:dbl)
                    n539 = local write "lick  #  2.1L"(w932) -> ()
                    n540 = local read "Mouse path 2"() -> (w936:path)
                    n541 = local read "mistake # 2.2R"() -> (w926:dbl)
                    n542 = local read "mistake # 2.1L"() -> (w927:dbl)
                    n543 = Build Array(w934, w932, w931, w930, w929, w928, w928, w928, w928, w928, w928, w927, w926) -> (w935:dbl[])
                    n544 = call-poly <vilib>:"Write To Spreadsheet File.vi"("append to file? (new file:F)"=TRUE, "1D data"=w935, "file path (dialog if empty)"=w936) -> ()  [unwired: 5 in, 1 out]
                  }
                }
              }
            }
            n545 = case shown="True" w853 {
              frame False {
              }
              frame True {
                n546 = local read "state 2.2"() -> (w855:enum16{"waiting", "sound", "ITI"})
                n547 = case shown="\"waiting\", Default" w855 {
                  frame "waiting", Default {
                    w862 = 0.0 ("element")
                    n548 = local read "water # 2.2R"() -> (w857:dbl)
                    n549 = local read "water # 2.1L"() -> (w863:dbl)
                    n550 = local read "lick  #  2.2R"() -> (w865:dbl)
                    n551 = local read "mistake # 2.2R"() -> (w860:dbl)
                    n552 = local read "mistake # 2.1L"() -> (w861:dbl)
                    n553 = local read "lick  #  2.1L"() -> (w866:dbl)
                    n554 = local read "time (s)"() -> (w859:dbl)
                    n555 = Increment(x=w857) -> (x+1=w856:dbl)
                    n556 = Increment(x=w865) -> (x+1=w864:dbl)
                    n557 = local write "water # 2.2R"(w856) -> ()
                    n558 = local read "free water 2.2"() -> (w858:bool)
                    n559 = local write "lick  #  2.2R"(w864) -> ()
                    n560 = local write "last water 2.2R"(w859) -> ()
                    n561 = local read "Mouse path 2"() -> (w868:path)
                    n562 = Build Array(w859, w866, w864, w863, w856, w862, w862, w862, w862, w862, w862, w861, w860) -> (w867:dbl[])
                    n563 = case shown="False" w858 {
                      frame False {
                        n564 = call "_digital_on_duration_off.vi"("duration (ms)"="water dur (ms) 2.2", "digital port"="water port 2.2") -> ()  [unwired: 10 in]
                      }
                      frame True {
                      }
                    }
                    n565 = local write "state 2.2"(enum16{"waiting", "sound", "ITI"}."ITI") -> ()
                    n566 = call-poly <vilib>:"Write To Spreadsheet File.vi"("append to file? (new file:F)"=TRUE, "1D data"=w867, "file path (dialog if empty)"=w868) -> ()  [unwired: 5 in, 1 out]
                    n567 = local write "state 2.1"(enum16{"waiting", "sound", "ITI"}."ITI") -> ()
                  }
                  frame "ITI" {
                    w876 = 0.0 ("element")
                    n568 = local read "water # 2.2R"() -> (w877:dbl)
                    n569 = local read "water # 2.1L"() -> (w878:dbl)
                    n570 = local read "lick  #  2.2R"() -> (w880:dbl)
                    n571 = local read "mistake # 2.2R"() -> (w874:dbl)
                    n572 = local read "mistake # 2.1L"() -> (w875:dbl)
                    n573 = local read "lick  #  2.1L"() -> (w881:dbl)
                    n574 = local read "time (s)"() -> (w882:dbl)
                    n575 = Increment(x=w880) -> (x+1=w879:dbl)
                    n576 = local write "lick  #  2.2R"(w879) -> ()
                    n577 = local read "Mouse path 2"() -> (w885:path)
                    n578 = Build Array(w882, w881, w879, w878, w877, w876, w876, w876, w876, w876, w876, w875, w874) -> (w883:dbl[])
                    n579 = call-poly <vilib>:"Write To Spreadsheet File.vi"("append to file? (new file:F)"=TRUE, "1D data"=w883, "file path (dialog if empty)"=w885) -> ()  [unwired: 5 in, 1 out]
                  }
                  frame "sound" {
                    w888 = 0.0 ("element")
                    n580 = local read "lick  #  2.2R"() -> (w892:dbl)
                    n581 = local read "water # 2.2R"() -> (w889:dbl)
                    n582 = local read "water # 2.1L"() -> (w890:dbl)
                    n583 = local read "lick  #  2.1L"() -> (w893:dbl)
                    n584 = local read "mistake # 2.2R"() -> (w886:dbl)
                    n585 = local read "time (s)"() -> (w894:dbl)
                    n586 = Increment(x=w892) -> (x+1=w891:dbl)
                    n587 = local read "mistake # 2.1L"() -> (w887:dbl)
                    n588 = local write "lick  #  2.2R"(w891) -> ()
                    n589 = local read "Mouse path 2"() -> (w897:path)
                    n590 = Build Array(w894, w893, w891, w890, w889, w888, w888, w888, w888, w888, w888, w887, w886) -> (w895:dbl[])
                    n591 = call-poly <vilib>:"Write To Spreadsheet File.vi"("append to file? (new file:F)"=TRUE, "1D data"=w895, "file path (dialog if empty)"=w897) -> ()  [unwired: 5 in, 1 out]
                  }
                }
              }
            }
          }
          frame 3 {
            n592 = case shown="True" w939 {
              frame False {
              }
              frame True {
                n593 = local read "state 2.1"() -> (w980:enum16{"waiting", "sound", "ITI"})
                n594 = case shown="\"waiting\", Default" w980 {
                  frame "waiting", Default {
                    w985 = 0.0 ("element")
                    n595 = local read "water # 2.1L"() -> (w988:dbl)
                    n596 = local read "lick  #  2.2R"() -> (w989:dbl)
                    n597 = local read "lick  #  2.1L"() -> (w991:dbl)
                    n598 = local read "water # 2.2R"() -> (w986:dbl)
                    n599 = local write "state 2.2"(enum16{"waiting", "sound", "ITI"}."ITI") -> ()
                    n600 = local write "state 2.1"(enum16{"waiting", "sound", "ITI"}."ITI") -> ()
                    n601 = local read "mistake # 2.2R"() -> (w983:dbl)
                    n602 = Increment(x=w988) -> (x+1=w987:dbl)
                    n603 = local read "mistake # 2.1L"() -> (w984:dbl)
                    n604 = Increment(x=w991) -> (x+1=w990:dbl)
                    n605 = local read "time (s)"() -> (w982:dbl)
                    n606 = local read "free water 2.1"() -> (w981:bool)
                    n607 = local write "water # 2.1L"(w987) -> ()
                    n608 = local write "lick  #  2.1L"(w990) -> ()
                    n609 = local write "last water 2.1L"(w982) -> ()
                    n610 = case shown="False" w981 {
                      frame False {
                        n611 = local read "water dur (ms) 2.1"() -> (w998:dbl)
                        n612 = local read "water port 2.1"() -> (w997:tag)
                        n613 = call "_digital_on_duration_off.vi"("duration (ms)"=w998, "digital port"=w997) -> ()  [unwired: 10 in]
                      }
                      frame True {
                      }
                    }
                    n614 = Build Array(w982, w990, w989, w987, w986, w985, w985, w985, w985, w985, w985, w984, w983) -> (w992:dbl[])
                    n615 = local read "Mouse path 2"() -> (w993:path)
                    n616 = call-poly <vilib>:"Write To Spreadsheet File.vi"("append to file? (new file:F)"=TRUE, "1D data"=w992, "file path (dialog if empty)"=w993) -> ()  [unwired: 5 in, 1 out]
                  }
                  frame "ITI" {
                    w1001 = 0.0 ("element")
                    n617 = local read "lick  #  2.2R"() -> (w1004:dbl)
                    n618 = local read "water # 2.2R"() -> (w1002:dbl)
                    n619 = local read "water # 2.1L"() -> (w1003:dbl)
                    n620 = local read "lick  #  2.1L"() -> (w1006:dbl)
                    n621 = local read "mistake # 2.2R"() -> (w999:dbl)
                    n622 = local read "mistake # 2.1L"() -> (w1000:dbl)
                    n623 = local read "time (s)"() -> (w1007:dbl)
                    n624 = Increment(x=w1006) -> (x+1=w1005:dbl)
                    n625 = local write "lick  #  2.1L"(w1005) -> ()
                    n626 = local read "Mouse path 2"() -> (w1009:path)
                    n627 = Build Array(w1007, w1005, w1004, w1003, w1002, w1001, w1001, w1001, w1001, w1001, w1001, w1000, w999) -> (w1008:dbl[])
                    n628 = call-poly <vilib>:"Write To Spreadsheet File.vi"("append to file? (new file:F)"=TRUE, "1D data"=w1008, "file path (dialog if empty)"=w1009) -> ()  [unwired: 5 in, 1 out]
                  }
                  frame "sound" {
                    w1013 = 0.0 ("element")
                    n629 = local read "water # 2.2R"() -> (w1014:dbl)
                    n630 = local read "water # 2.1L"() -> (w1015:dbl)
                    n631 = local read "mistake # 2.2R"() -> (w1011:dbl)
                    n632 = local read "lick  #  2.1L"() -> (w1018:dbl)
                    n633 = local read "mistake # 2.1L"() -> (w1012:dbl)
                    n634 = local read "lick  #  2.2R"() -> (w1016:dbl)
                    n635 = local read "time (s)"() -> (w1019:dbl)
                    n636 = Increment(x=w1018) -> (x+1=w1017:dbl)
                    n637 = local read "Mouse path 2"() -> (w1021:path)
                    n638 = local write "lick  #  2.1L"(w1017) -> ()
                    n639 = Build Array(w1019, w1017, w1016, w1015, w1014, w1013, w1013, w1013, w1013, w1013, w1013, w1012, w1011) -> (w1020:dbl[])
                    n640 = call-poly <vilib>:"Write To Spreadsheet File.vi"("append to file? (new file:F)"=TRUE, "1D data"=w1020, "file path (dialog if empty)"=w1021) -> ()  [unwired: 5 in, 1 out]
                  }
                }
              }
            }
            n641 = case shown="True" w938 {
              frame False {
              }
              frame True {
                n642 = local read "state 2.1"() -> (w940:enum16{"waiting", "sound", "ITI"})
                n643 = case shown="\"waiting\", Default" w940 {
                  frame "waiting", Default {
                    w944 = 0.0 ("element")
                    n644 = local write "state 2.2"(enum16{"waiting", "sound", "ITI"}."ITI") -> ()
                    n645 = local write "state 2.1"(enum16{"waiting", "sound", "ITI"}."ITI") -> ()
                    n646 = local read "water # 2.2R"() -> (w945:dbl)
                    n647 = local read "mistake # 2.2R"() -> (w941:dbl)
                    n648 = local read "water # 2.1L"() -> (w946:dbl)
                    n649 = local read "lick  #  2.2R"() -> (w948:dbl)
                    n650 = local read "mistake # 2.1L"() -> (w943:dbl)
                    n651 = local read "lick  #  2.1L"() -> (w949:dbl)
                    n652 = local read "time (s)"() -> (w950:dbl)
                    n653 = Increment(x=w948) -> (x+1=w947:dbl)
                    n654 = Increment(x=w943) -> (x+1=w942:dbl)
                    n655 = local write "mistake # 2.1L"(w942) -> ()
                    n656 = local write "lick  #  2.2R"(w947) -> ()
                    n657 = local read "Mouse path 2"() -> (w953:path)
                    n658 = Build Array(w950, w949, w947, w946, w945, w944, w944, w944, w944, w944, w944, w942, w941) -> (w951:dbl[])
                    n659 = call-poly <vilib>:"Write To Spreadsheet File.vi"("append to file? (new file:F)"=TRUE, "1D data"=w951, "file path (dialog if empty)"=w953) -> ()  [unwired: 5 in, 1 out]
                  }
                  frame "ITI" {
                    w958 = 0.0 ("element")
                    n660 = local read "water # 2.2R"() -> (w959:dbl)
                    n661 = local read "water # 2.1L"() -> (w960:dbl)
                    n662 = local read "lick  #  2.2R"() -> (w962:dbl)
                    n663 = local read "lick  #  2.1L"() -> (w963:dbl)
                    n664 = local read "mistake # 2.2R"() -> (w956:dbl)
                    n665 = local read "mistake # 2.1L"() -> (w957:dbl)
                    n666 = local read "time (s)"() -> (w964:dbl)
                    n667 = Increment(x=w962) -> (x+1=w961:dbl)
                    n668 = local write "lick  #  2.2R"(w961) -> ()
                    n669 = local read "Mouse path 2"() -> (w966:path)
                    n670 = Build Array(w964, w963, w961, w960, w959, w958, w958, w958, w958, w958, w958, w957, w956) -> (w965:dbl[])
                    n671 = call-poly <vilib>:"Write To Spreadsheet File.vi"("append to file? (new file:F)"=TRUE, "1D data"=w965, "file path (dialog if empty)"=w966) -> ()  [unwired: 5 in, 1 out]
                  }
                  frame "sound" {
                    w970 = 0.0 ("element")
                    n672 = local read "water # 2.2R"() -> (w971:dbl)
                    n673 = local read "water # 2.1L"() -> (w972:dbl)
                    n674 = local read "lick  #  2.2R"() -> (w974:dbl)
                    n675 = local read "mistake # 2.2R"() -> (w968:dbl)
                    n676 = local read "mistake # 2.1L"() -> (w969:dbl)
                    n677 = local read "lick  #  2.1L"() -> (w975:dbl)
                    n678 = Increment(x=w974) -> (x+1=w973:dbl)
                    n679 = local read "time (s)"() -> (w976:dbl)
                    n680 = local write "lick  #  2.2R"(w973) -> ()
                    n681 = local read "Mouse path 2"() -> (w978:path)
                    n682 = Build Array(w976, w975, w973, w972, w971, w970, w970, w970, w970, w970, w970, w969, w968) -> (w977:dbl[])
                    n683 = call-poly <vilib>:"Write To Spreadsheet File.vi"("append to file? (new file:F)"=TRUE, "1D data"=w977, "file path (dialog if empty)"=w978) -> ()  [unwired: 5 in, 1 out]
                  }
                }
              }
            }
          }
          frame 4 {
            n684 = case shown="True" w1024 {
              frame False {
              }
              frame True {
                n685 = local read "state 2.2"() -> (w1068:enum16{"waiting", "sound", "ITI"})
                n686 = case shown="\"waiting\", Default" w1068 {
                  frame "waiting", Default {
                    w1072 = 0.0 ("element")
                    n687 = local read "lick  #  2.2R"() -> (w1075:dbl)
                    n688 = local read "lick  #  2.1L"() -> (w1077:dbl)
                    n689 = local read "water # 2.2R"() -> (w1073:dbl)
                    n690 = local read "water # 2.1L"() -> (w1074:dbl)
                    n691 = local read "mistake # 2.2R"() -> (w1070:dbl)
                    n692 = local read "mistake # 2.1L"() -> (w1071:dbl)
                    n693 = local read "time (s)"() -> (w1078:dbl)
                    n694 = Increment(x=w1077) -> (x+1=w1076:dbl)
                    n695 = local write "lick  #  2.1L"(w1076) -> ()
                    n696 = local read "Mouse path 2"() -> (w1080:path)
                    n697 = Increment(x=w1070) -> (x+1=w1069:dbl)
                    n698 = local write "mistake # 2.2R"(w1069) -> ()
                    n699 = Build Array(w1078, w1076, w1075, w1074, w1073, w1072, w1072, w1072, w1072, w1072, w1072, w1071, w1069) -> (w1079:dbl[])
                    n700 = call-poly <vilib>:"Write To Spreadsheet File.vi"("append to file? (new file:F)"=TRUE, "1D data"=w1079, "file path (dialog if empty)"=w1080) -> ()  [unwired: 5 in, 1 out]
                    n701 = local write "state 2.2"(enum16{"waiting", "sound", "ITI"}."ITI") -> ()
                    n702 = local write "state 2.1"(enum16{"waiting", "sound", "ITI"}."ITI") -> ()
                  }
                  frame "sound" {
                    w1086 = 0.0 ("element")
                    n703 = local read "lick  #  2.2R"() -> (w1089:dbl)
                    n704 = local read "lick  #  2.1L"() -> (w1091:dbl)
                    n705 = local read "water # 2.2R"() -> (w1087:dbl)
                    n706 = local read "water # 2.1L"() -> (w1088:dbl)
                    n707 = local read "mistake # 2.2R"() -> (w1084:dbl)
                    n708 = local read "mistake # 2.1L"() -> (w1085:dbl)
                    n709 = local read "time (s)"() -> (w1092:dbl)
                    n710 = Increment(x=w1091) -> (x+1=w1090:dbl)
                    n711 = local write "lick  #  2.1L"(w1090) -> ()
                    n712 = local read "Mouse path 2"() -> (w1094:path)
                    n713 = Build Array(w1092, w1090, w1089, w1088, w1087, w1086, w1086, w1086, w1086, w1086, w1086, w1085, w1084) -> (w1093:dbl[])
                    n714 = call-poly <vilib>:"Write To Spreadsheet File.vi"("append to file? (new file:F)"=TRUE, "1D data"=w1093, "file path (dialog if empty)"=w1094) -> ()  [unwired: 5 in, 1 out]
                  }
                  frame "ITI" {
                    w1098 = 0.0 ("element")
                    n715 = local read "water # 2.1L"() -> (w1100:dbl)
                    n716 = local read "water # 2.2R"() -> (w1099:dbl)
                    n717 = local read "lick  #  2.2R"() -> (w1101:dbl)
                    n718 = local read "lick  #  2.1L"() -> (w1103:dbl)
                    n719 = local read "mistake # 2.2R"() -> (w1096:dbl)
                    n720 = local read "mistake # 2.1L"() -> (w1097:dbl)
                    n721 = local read "time (s)"() -> (w1104:dbl)
                    n722 = Increment(x=w1103) -> (x+1=w1102:dbl)
                    n723 = local write "lick  #  2.1L"(w1102) -> ()
                    n724 = local read "Mouse path 2"() -> (w1106:path)
                    n725 = Build Array(w1104, w1102, w1101, w1100, w1099, w1098, w1098, w1098, w1098, w1098, w1098, w1097, w1096) -> (w1105:dbl[])
                    n726 = call-poly <vilib>:"Write To Spreadsheet File.vi"("append to file? (new file:F)"=TRUE, "1D data"=w1105, "file path (dialog if empty)"=w1106) -> ()  [unwired: 5 in, 1 out]
                  }
                }
              }
            }
            n727 = case shown="True" w1023 {
              frame False {
              }
              frame True {
                n728 = local read "state 2.2"() -> (w1025:enum16{"waiting", "sound", "ITI"})
                n729 = case shown="\"waiting\", Default" w1025 {
                  frame "waiting", Default {
                    w1029 = 0.0 ("element")
                    n730 = local read "water # 2.2R"() -> (w1031:dbl)
                    n731 = local read "lick  #  2.2R"() -> (w1034:dbl)
                    n732 = local read "water # 2.1L"() -> (w1032:dbl)
                    n733 = local read "lick  #  2.1L"() -> (w1035:dbl)
                    n734 = local read "mistake # 2.2R"() -> (w1027:dbl)
                    n735 = local read "time (s)"() -> (w1036:dbl)
                    n736 = local read "mistake # 2.1L"() -> (w1028:dbl)
                    n737 = Increment(x=w1034) -> (x+1=w1033:dbl)
                    n738 = Increment(x=w1031) -> (x+1=w1030:dbl)
                    n739 = local write "state 2.1"(enum16{"waiting", "sound", "ITI"}."ITI") -> ()
                    n740 = local write "state 2.2"(enum16{"waiting", "sound", "ITI"}."ITI") -> ()
                    n741 = local write "water # 2.2R"(w1030) -> ()
                    n742 = local write "lick  #  2.2R"(w1033) -> ()
                    n743 = local read "Mouse path 2"() -> (w1038:path)
                    n744 = Build Array(w1036, w1035, w1033, w1032, w1030, w1029, w1029, w1029, w1029, w1029, w1029, w1028, w1027) -> (w1037:dbl[])
                    n745 = call-poly <vilib>:"Write To Spreadsheet File.vi"("append to file? (new file:F)"=TRUE, "1D data"=w1037, "file path (dialog if empty)"=w1038) -> ()  [unwired: 5 in, 1 out]
                    n746 = local read "free water 2.2"() -> (w1026:bool)
                    n747 = case shown="False" w1026 {
                      frame False {
                        n748 = local read "water dur (ms) 2.2"() -> (w1043:dbl)
                        n749 = local read "water port 2.2"() -> (w1042:tag)
                        n750 = call "_digital_on_duration_off.vi"("duration (ms)"=w1043, "digital port"=w1042) -> ()  [unwired: 10 in]
                      }
                      frame True {
                      }
                    }
                  }
                  frame "sound" {
                    w1046 = 0.0 ("element")
                    n751 = local read "water # 2.1L"() -> (w1048:dbl)
                    n752 = local read "water # 2.2R"() -> (w1047:dbl)
                    n753 = local read "lick  #  2.2R"() -> (w1050:dbl)
                    n754 = local read "lick  #  2.1L"() -> (w1051:dbl)
                    n755 = local read "mistake # 2.2R"() -> (w1044:dbl)
                    n756 = local read "mistake # 2.1L"() -> (w1045:dbl)
                    n757 = local read "time (s)"() -> (w1052:dbl)
                    n758 = Increment(x=w1050) -> (x+1=w1049:dbl)
                    n759 = local write "lick  #  2.2R"(w1049) -> ()
                    n760 = local read "Mouse path 2"() -> (w1055:path)
                    n761 = Build Array(w1052, w1051, w1049, w1048, w1047, w1046, w1046, w1046, w1046, w1046, w1046, w1045, w1044) -> (w1053:dbl[])
                    n762 = call-poly <vilib>:"Write To Spreadsheet File.vi"("append to file? (new file:F)"=TRUE, "1D data"=w1053, "file path (dialog if empty)"=w1055) -> ()  [unwired: 5 in, 1 out]
                  }
                  frame "ITI" {
                    w1058 = 0.0 ("element")
                    n763 = local read "water # 2.2R"() -> (w1059:dbl)
                    n764 = local read "water # 2.1L"() -> (w1060:dbl)
                    n765 = local read "lick  #  2.2R"() -> (w1062:dbl)
                    n766 = local read "lick  #  2.1L"() -> (w1063:dbl)
                    n767 = local read "time (s)"() -> (w1064:dbl)
                    n768 = Increment(x=w1062) -> (x+1=w1061:dbl)
                    n769 = local read "mistake # 2.2R"() -> (w1056:dbl)
                    n770 = local read "mistake # 2.1L"() -> (w1057:dbl)
                    n771 = local write "lick  #  2.2R"(w1061) -> ()
                    n772 = local read "Mouse path 2"() -> (w1065:path)
                    n773 = Build Array(w1064, w1063, w1061, w1060, w1059, w1058, w1058, w1058, w1058, w1058, w1058, w1057, w1056) -> (w1066:dbl[])
                    n774 = call-poly <vilib>:"Write To Spreadsheet File.vi"("append to file? (new file:F)"=TRUE, "1D data"=w1066, "file path (dialog if empty)"=w1065) -> ()  [unwired: 5 in, 1 out]
                  }
                }
              }
            }
          }
        }
        n775 = case shown="2" w42 {
          tunnel: w31 -> [_ w88 w174 w259 w344]
          tunnel: w32 -> [_ w89 w173 w258 w343]
          frame 0, Default {
          }
          frame 1 {
            n776 = case shown="True" w89 {
              frame False {
              }
              frame True {
                n777 = local read "state 4.1"() -> (w133:enum16{"waiting", "sound", "ITI"})
                n778 = case shown="\"waiting\", Default" w133 {
                  frame "waiting", Default {
                    w137 = 0.0 ("element")
                    n779 = local read "water # 4.1L"() -> (w139:dbl)
                    n780 = local read "water # 4.2R"() -> (w138:dbl)
                    n781 = local read "lick # 4.2R"() -> (w141:dbl)
                    n782 = local read "lick # 4.1L"() -> (w142:dbl)
                    n783 = local write "state 4.2"(enum16{"waiting", "sound", "ITI"}."ITI") -> ()
                    n784 = local read "mistake # 4.2R"() -> (w134:dbl)
                    n785 = local write "state 4.1"(enum16{"waiting", "sound", "ITI"}."ITI") -> ()
                    n786 = local read "mistake # 4.1L"() -> (w136:dbl)
                    n787 = Increment(x=w141) -> (x+1=w140:dbl)
                    n788 = local read "time (s)"() -> (w143:dbl)
                    n789 = local write "lick # 4.2R"(w140) -> ()
                    n790 = Increment(x=w136) -> (x+1=w135:dbl)
                    n791 = local read "Mouse path 4"() -> (w145:path)
                    n792 = local write "mistake # 4.1L"(w135) -> ()
                    n793 = Build Array(w143, w142, w140, w139, w138, w137, w137, w137, w137, w137, w137, w135, w134) -> (w144:dbl[])
                    n794 = call-poly <vilib>:"Write To Spreadsheet File.vi"("append to file? (new file:F)"=TRUE, "1D data"=w144, "file path (dialog if empty)"=w145) -> ()  [unwired: 5 in, 1 out]
                  }
                  frame "sound" {
                    w151 = 0.0 ("element")
                    n795 = local read "water # 4.2R"() -> (w152:dbl)
                    n796 = local read "lick # 4.2R"() -> (w155:dbl)
                    n797 = local read "water # 4.1L"() -> (w153:dbl)
                    n798 = local read "lick # 4.1L"() -> (w156:dbl)
                    n799 = local read "mistake # 4.2R"() -> (w149:dbl)
                    n800 = local read "time (s)"() -> (w157:dbl)
                    n801 = Increment(x=w155) -> (x+1=w154:dbl)
                    n802 = local read "mistake # 4.1L"() -> (w150:dbl)
                    n803 = local write "lick # 4.2R"(w154) -> ()
                    n804 = local read "Mouse path 4"() -> (w159:path)
                    n805 = Build Array(w157, w156, w154, w153, w152, w151, w151, w151, w151, w151, w151, w150, w149) -> (w158:dbl[])
                    n806 = call-poly <vilib>:"Write To Spreadsheet File.vi"("append to file? (new file:F)"=TRUE, "1D data"=w158, "file path (dialog if empty)"=w159) -> ()  [unwired: 5 in, 1 out]
                  }
                  frame "ITI" {
                    w163 = 0.0 ("element")
                    n807 = local read "mistake # 4.2R"() -> (w161:dbl)
                    n808 = local read "water # 4.2R"() -> (w164:dbl)
                    n809 = local read "mistake # 4.1L"() -> (w162:dbl)
                    n810 = local read "water # 4.1L"() -> (w165:dbl)
                    n811 = local read "lick # 4.2R"() -> (w167:dbl)
                    n812 = local read "lick # 4.1L"() -> (w168:dbl)
                    n813 = local read "time (s)"() -> (w169:dbl)
                    n814 = Increment(x=w167) -> (x+1=w166:dbl)
                    n815 = local write "lick # 4.2R"(w166) -> ()
                    n816 = local read "Mouse path 4"() -> (w171:path)
                    n817 = Build Array(w169, w168, w166, w165, w164, w163, w163, w163, w163, w163, w163, w162, w161) -> (w170:dbl[])
                    n818 = call-poly <vilib>:"Write To Spreadsheet File.vi"("append to file? (new file:F)"=TRUE, "1D data"=w170, "file path (dialog if empty)"=w171) -> ()  [unwired: 5 in, 1 out]
                  }
                }
              }
            }
            n819 = case shown="True" w88 {
              frame False {
              }
              frame True {
                n820 = local read "state 4.1"() -> (w90:enum16{"waiting", "sound", "ITI"})
                n821 = case shown="\"waiting\", Default" w90 {
                  frame "waiting", Default {
                    w94 = 0.0 ("element")
                    n822 = local read "water # 4.1L"() -> (w97:dbl)
                    n823 = local read "lick # 4.2R"() -> (w98:dbl)
                    n824 = local read "lick # 4.1L"() -> (w100:dbl)
                    n825 = local read "water # 4.2R"() -> (w95:dbl)
                    n826 = local read "mistake # 4.2R"() -> (w92:dbl)
                    n827 = local read "time (s)"() -> (w91:dbl)
                    n828 = local read "mistake # 4.1L"() -> (w93:dbl)
                    n829 = Increment(x=w97) -> (x+1=w96:dbl)
                    n830 = Increment(x=w100) -> (x+1=w99:dbl)
                    n831 = local write "state 4.2"(enum16{"waiting", "sound", "ITI"}."ITI") -> ()
                    n832 = local write "state 4.1"(enum16{"waiting", "sound", "ITI"}."ITI") -> ()
                    n833 = local write "water # 4.1L"(w96) -> ()
                    n834 = local write "last water 4.1L"(w91) -> ()
                    n835 = local write "lick # 4.1L"(w99) -> ()
                    n836 = local read "Mouse path 4"() -> (w102:path)
                    n837 = Build Array(w91, w99, w98, w96, w95, w94, w94, w94, w94, w94, w94, w93, w92) -> (w101:dbl[])
                    n838 = local read "free water 4.1"() -> (w104:bool)
                    n839 = call-poly <vilib>:"Write To Spreadsheet File.vi"("append to file? (new file:F)"=TRUE, "1D data"=w101, "file path (dialog if empty)"=w102) -> ()  [unwired: 5 in, 1 out]
                    n840 = case shown="False" w104 {
                      frame False {
                        n841 = call "_digital_on_duration_off.vi"("duration (ms)"="water dur (ms) 4.1", "digital port"="water port 4.1") -> ()  [unwired: 10 in]
                      }
                      frame True {
                      }
                    }
                  }
                  frame "sound" {
                    w111 = 0.0 ("element")
                    n842 = local read "water # 4.2R"() -> (w112:dbl)
                    n843 = local read "water # 4.1L"() -> (w113:dbl)
                    n844 = local read "mistake # 4.2R"() -> (w109:dbl)
                    n845 = local read "lick # 4.2R"() -> (w114:dbl)
                    n846 = local read "mistake # 4.1L"() -> (w110:dbl)
                    n847 = local read "lick # 4.1L"() -> (w116:dbl)
                    n848 = local read "time (s)"() -> (w117:dbl)
                    n849 = Increment(x=w116) -> (x+1=w115:dbl)
                    n850 = local write "lick # 4.1L"(w115) -> ()
                    n851 = local read "Mouse path 4"() -> (w119:path)
                    n852 = Build Array(w117, w115, w114, w113, w112, w111, w111, w111, w111, w111, w111, w110, w109) -> (w118:dbl[])
                    n853 = call-poly <vilib>:"Write To Spreadsheet File.vi"("append to file? (new file:F)"=TRUE, "1D data"=w118, "file path (dialog if empty)"=w119) -> ()  [unwired: 5 in, 1 out]
                  }
                  frame "ITI" {
                    w123 = 0.0 ("element")
                    n854 = local read "water # 4.2R"() -> (w124:dbl)
                    n855 = local read "water # 4.1L"() -> (w125:dbl)
                    n856 = local read "mistake # 4.2R"() -> (w121:dbl)
                    n857 = local read "lick # 4.2R"() -> (w126:dbl)
                    n858 = local read "mistake # 4.1L"() -> (w122:dbl)
                    n859 = local read "lick # 4.1L"() -> (w128:dbl)
                    n860 = local read "time (s)"() -> (w129:dbl)
                    n861 = Increment(x=w128) -> (x+1=w127:dbl)
                    n862 = local write "lick # 4.1L"(w127) -> ()
                    n863 = local read "Mouse path 4"() -> (w131:path)
                    n864 = Build Array(w129, w127, w126, w125, w124, w123, w123, w123, w123, w123, w123, w122, w121) -> (w130:dbl[])
                    n865 = call-poly <vilib>:"Write To Spreadsheet File.vi"("append to file? (new file:F)"=TRUE, "1D data"=w130, "file path (dialog if empty)"=w131) -> ()  [unwired: 5 in, 1 out]
                  }
                }
              }
            }
          }
          frame 2 {
            n866 = case shown="True" w173 {
              frame False {
              }
              frame True {
                n867 = local read "state 4.2"() -> (w215:enum16{"waiting", "sound", "ITI"})
                n868 = case shown="\"waiting\", Default" w215 {
                  frame "waiting", Default {
                    w219 = 0.0 ("element")
                    n869 = local read "water # 4.2R"() -> (w221:dbl)
                    n870 = local read "mistake # 4.2R"() -> (w217:dbl)
                    n871 = local read "mistake # 4.1L"() -> (w218:dbl)
                    n872 = local read "water # 4.1L"() -> (w222:dbl)
                    n873 = local read "lick # 4.2R"() -> (w224:dbl)
                    n874 = local write "state 4.2"(enum16{"waiting", "sound", "ITI"}."ITI") -> ()
                    n875 = local write "state 4.1"(enum16{"waiting", "sound", "ITI"}."ITI") -> ()
                    n876 = local read "lick # 4.1L"() -> (w225:dbl)
                    n877 = Increment(x=w221) -> (x+1=w220:dbl)
                    n878 = local read "time (s)"() -> (w216:dbl)
                    n879 = local write "water # 4.2R"(w220) -> ()
                    n880 = Increment(x=w224) -> (x+1=w223:dbl)
                    n881 = local write "last water 4.2R"(w216) -> ()
                    n882 = local read "free water 4.2"() -> (w229:bool)
                    n883 = local write "lick # 4.2R"(w223) -> ()
                    n884 = Build Array(w216, w225, w223, w222, w220, w219, w219, w219, w219, w219, w219, w218, w217) -> (w226:dbl[])
                    n885 = local read "Mouse path 4"() -> (w227:path)
                    n886 = case shown="False" w229 {
                      frame False {
                        n887 = call "_digital_on_duration_off.vi"("duration (ms)"="water dur (ms) 4.2", "digital port"="water port 4.2") -> ()  [unwired: 10 in]
                      }
                      frame True {
                      }
                    }
                    n888 = call-poly <vilib>:"Write To Spreadsheet File.vi"("append to file? (new file:F)"=TRUE, "1D data"=w226, "file path (dialog if empty)"=w227) -> ()  [unwired: 5 in, 1 out]
                  }
                  frame "sound" {
                    w236 = 0.0 ("element")
                    n889 = local read "water # 4.1L"() -> (w238:dbl)
                    n890 = local read "water # 4.2R"() -> (w237:dbl)
                    n891 = local read "mistake # 4.2R"() -> (w234:dbl)
                    n892 = local read "lick # 4.2R"() -> (w240:dbl)
                    n893 = local read "mistake # 4.1L"() -> (w235:dbl)
                    n894 = local read "lick # 4.1L"() -> (w241:dbl)
                    n895 = local read "time (s)"() -> (w242:dbl)
                    n896 = Increment(x=w240) -> (x+1=w239:dbl)
                    n897 = local write "lick # 4.2R"(w239) -> ()
                    n898 = Build Array(w242, w241, w239, w238, w237, w236, w236, w236, w236, w236, w236, w235, w234) -> (w243:dbl[])
                    n899 = local read "Mouse path 4"() -> (w244:path)
                    n900 = call-poly <vilib>:"Write To Spreadsheet File.vi"("append to file? (new file:F)"=TRUE, "1D data"=w243, "file path (dialog if empty)"=w244) -> ()  [unwired: 5 in, 1 out]
                  }
                  frame "ITI" {
                    w248 = 0.0 ("element")
                    n901 = local read "water # 4.2R"() -> (w249:dbl)
                    n902 = local read "water # 4.1L"() -> (w250:dbl)
                    n903 = local read "lick # 4.2R"() -> (w252:dbl)
                    n904 = local read "lick # 4.1L"() -> (w253:dbl)
                    n905 = local read "mistake # 4.2R"() -> (w246:dbl)
                    n906 = Increment(x=w252) -> (x+1=w251:dbl)
                    n907 = local read "mistake # 4.1L"() -> (w247:dbl)
                    n908 = local read "time (s)"() -> (w254:dbl)
                    n909 = local write "lick # 4.2R"(w251) -> ()
                    n910 = Build Array(w254, w253, w251, w250, w249, w248, w248, w248, w248, w248, w248, w247, w246) -> (w255:dbl[])
                    n911 = local read "Mouse path 4"() -> (w256:path)
                    n912 = call-poly <vilib>:"Write To Spreadsheet File.vi"("append to file? (new file:F)"=TRUE, "1D data"=w255, "file path (dialog if empty)"=w256) -> ()  [unwired: 5 in, 1 out]
                  }
                }
              }
            }
            n913 = case shown="True" w174 {
              frame False {
              }
              frame True {
                n914 = local read "state 4.2"() -> (w175:enum16{"waiting", "sound", "ITI"})
                n915 = case shown="\"waiting\", Default" w175 {
                  frame "waiting", Default {
                    w179 = 0.0 ("element")
                    n916 = local read "lick # 4.2R"() -> (w182:dbl)
                    n917 = local read "lick # 4.1L"() -> (w184:dbl)
                    n918 = local read "mistake # 4.2R"() -> (w177:dbl)
                    n919 = local read "water # 4.1L"() -> (w181:dbl)
                    n920 = local read "water # 4.2R"() -> (w180:dbl)
                    n921 = local read "time (s)"() -> (w185:dbl)
                    n922 = local read "mistake # 4.1L"() -> (w178:dbl)
                    n923 = local write "state 4.2"(enum16{"waiting", "sound", "ITI"}."ITI") -> ()
                    n924 = local write "state 4.1"(enum16{"waiting", "sound", "ITI"}."ITI") -> ()
                    n925 = Increment(x=w184) -> (x+1=w183:dbl)
                    n926 = Increment(x=w177) -> (x+1=w176:dbl)
                    n927 = local write "mistake # 4.2R"(w176) -> ()
                    n928 = local write "lick # 4.1L"(w183) -> ()
                    n929 = Build Array(w185, w183, w182, w181, w180, w179, w179, w179, w179, w179, w179, w178, w176) -> (w186:dbl[])
                    n930 = local read "Mouse path 4"() -> (w187:path)
                    n931 = call-poly <vilib>:"Write To Spreadsheet File.vi"("append to file? (new file:F)"=TRUE, "1D data"=w186, "file path (dialog if empty)"=w187) -> ()  [unwired: 5 in, 1 out]
                  }
                  frame "sound" {
                    w193 = 0.0 ("element")
                    n932 = local read "mistake # 4.2R"() -> (w191:dbl)
                    n933 = local read "water # 4.2R"() -> (w194:dbl)
                    n934 = local read "mistake # 4.1L"() -> (w192:dbl)
                    n935 = local read "water # 4.1L"() -> (w195:dbl)
                    n936 = local read "lick # 4.2R"() -> (w196:dbl)
                    n937 = local read "lick # 4.1L"() -> (w198:dbl)
                    n938 = local read "time (s)"() -> (w199:dbl)
                    n939 = Increment(x=w198) -> (x+1=w197:dbl)
                    n940 = local write "lick # 4.1L"(w197) -> ()
                    n941 = Build Array(w199, w197, w196, w195, w194, w193, w193, w193, w193, w193, w193, w192, w191) -> (w200:dbl[])
                    n942 = local read "Mouse path 4"() -> (w201:path)
                    n943 = call-poly <vilib>:"Write To Spreadsheet File.vi"("append to file? (new file:F)"=TRUE, "1D data"=w200, "file path (dialog if empty)"=w201) -> ()  [unwired: 5 in, 1 out]
                  }
                  frame "ITI" {
                    w205 = 0.0 ("element")
                    n944 = local read "water # 4.1L"() -> (w207:dbl)
                    n945 = local read "water # 4.2R"() -> (w206:dbl)
                    n946 = local read "lick # 4.2R"() -> (w208:dbl)
                    n947 = local read "mistake # 4.2R"() -> (w203:dbl)
                    n948 = local read "lick # 4.1L"() -> (w210:dbl)
                    n949 = local read "mistake # 4.1L"() -> (w204:dbl)
                    n950 = local read "time (s)"() -> (w211:dbl)
                    n951 = Increment(x=w210) -> (x+1=w209:dbl)
                    n952 = local write "lick # 4.1L"(w209) -> ()
                    n953 = local read "Mouse path 4"() -> (w213:path)
                    n954 = Build Array(w211, w209, w208, w207, w206, w205, w205, w205, w205, w205, w205, w204, w203) -> (w212:dbl[])
                    n955 = call-poly <vilib>:"Write To Spreadsheet File.vi"("append to file? (new file:F)"=TRUE, "1D data"=w212, "file path (dialog if empty)"=w213) -> ()  [unwired: 5 in, 1 out]
                  }
                }
              }
            }
          }
          frame 3 {
            n956 = case shown="True" w258 {
              frame False {
              }
              frame True {
                n957 = local read "state 4.1"() -> (w303:enum16{"waiting", "sound", "ITI"})
                n958 = case shown="\"waiting\", Default" w303 {
                  frame "waiting", Default {
                    w307 = 0.0 ("element")
                    n959 = local write "state 4.2"(enum16{"waiting", "sound", "ITI"}."ITI") -> ()
                    n960 = local write "state 4.1"(enum16{"waiting", "sound", "ITI"}."ITI") -> ()
                    n961 = local read "water # 4.2R"() -> (w308:dbl)
                    n962 = local read "mistake # 4.1L"() -> (w306:dbl)
                    n963 = local read "water # 4.1L"() -> (w309:dbl)
                    n964 = local read "mistake # 4.2R"() -> (w304:dbl)
                    n965 = local read "lick # 4.2R"() -> (w311:dbl)
                    n966 = local read "lick # 4.1L"() -> (w312:dbl)
                    n967 = local read "time (s)"() -> (w313:dbl)
                    n968 = Increment(x=w306) -> (x+1=w305:dbl)
                    n969 = Increment(x=w311) -> (x+1=w310:dbl)
                    n970 = local write "mistake # 4.1L"(w305) -> ()
                    n971 = local write "lick # 4.2R"(w310) -> ()
                    n972 = local read "Mouse path 4"() -> (w315:path)
                    n973 = Build Array(w313, w312, w310, w309, w308, w307, w307, w307, w307, w307, w307, w305, w304) -> (w314:dbl[])
                    n974 = call-poly <vilib>:"Write To Spreadsheet File.vi"("append to file? (new file:F)"=TRUE, "1D data"=w314, "file path (dialog if empty)"=w315) -> ()  [unwired: 5 in, 1 out]
                  }
                  frame "sound" {
                    w321 = 0.0 ("element")
                    n975 = local read "lick # 4.2R"() -> (w325:dbl)
                    n976 = local read "water # 4.1L"() -> (w323:dbl)
                    n977 = local read "water # 4.2R"() -> (w322:dbl)
                    n978 = local read "mistake # 4.2R"() -> (w319:dbl)
                    n979 = local read "lick # 4.1L"() -> (w326:dbl)
                    n980 = local read "time (s)"() -> (w327:dbl)
                    n981 = local read "mistake # 4.1L"() -> (w320:dbl)
                    n982 = Increment(x=w325) -> (x+1=w324:dbl)
                    n983 = local write "lick # 4.2R"(w324) -> ()
                    n984 = Build Array(w327, w326, w324, w323, w322, w321, w321, w321, w321, w321, w321, w320, w319) -> (w328:dbl[])
                    n985 = local read "Mouse path 4"() -> (w329:path)
                    n986 = call-poly <vilib>:"Write To Spreadsheet File.vi"("append to file? (new file:F)"=TRUE, "1D data"=w328, "file path (dialog if empty)"=w329) -> ()  [unwired: 5 in, 1 out]
                  }
                  frame "ITI" {
                    w333 = 0.0 ("element")
                    n987 = local read "water # 4.2R"() -> (w334:dbl)
                    n988 = local read "water # 4.1L"() -> (w335:dbl)
                    n989 = local read "mistake # 4.1L"() -> (w332:dbl)
                    n990 = local read "mistake # 4.2R"() -> (w331:dbl)
                    n991 = local read "lick # 4.2R"() -> (w337:dbl)
                    n992 = local read "lick # 4.1L"() -> (w338:dbl)
                    n993 = local read "time (s)"() -> (w339:dbl)
                    n994 = Increment(x=w337) -> (x+1=w336:dbl)
                    n995 = local write "lick # 4.2R"(w336) -> ()
                    n996 = local read "Mouse path 4"() -> (w341:path)
                    n997 = Build Array(w339, w338, w336, w335, w334, w333, w333, w333, w333, w333, w333, w332, w331) -> (w340:dbl[])
                    n998 = call-poly <vilib>:"Write To Spreadsheet File.vi"("append to file? (new file:F)"=TRUE, "1D data"=w340, "file path (dialog if empty)"=w341) -> ()  [unwired: 5 in, 1 out]
                  }
                }
              }
            }
            n999 = case shown="True" w259 {
              frame False {
              }
              frame True {
                n1000 = local read "state 4.1"() -> (w260:enum16{"waiting", "sound", "ITI"})
                n1001 = case shown="\"waiting\", Default" w260 {
                  frame "waiting", Default {
                    w264 = 0.0 ("element")
                    n1002 = local read "water # 4.1L"() -> (w267:dbl)
                    n1003 = local write "state 4.2"(enum16{"waiting", "sound", "ITI"}."ITI") -> ()
                    n1004 = local read "water # 4.2R"() -> (w265:dbl)
                    n1005 = local write "state 4.1"(enum16{"waiting", "sound", "ITI"}."ITI") -> ()
                    n1006 = local read "lick # 4.2R"() -> (w268:dbl)
                    n1007 = local read "lick # 4.1L"() -> (w270:dbl)
                    n1008 = local read "time (s)"() -> (w261:dbl)
                    n1009 = local read "mistake # 4.2R"() -> (w262:dbl)
                    n1010 = Increment(x=w267) -> (x+1=w266:dbl)
                    n1011 = local read "mistake # 4.1L"() -> (w263:dbl)
                    n1012 = Increment(x=w270) -> (x+1=w269:dbl)
                    n1013 = local write "water # 4.1L"(w266) -> ()
                    n1014 = local write "last water 4.1L"(w261) -> ()
                    n1015 = local read "free water 4.1"() -> (w276:bool)
                    n1016 = local write "lick # 4.1L"(w269) -> ()
                    n1017 = local read "Mouse path 4"() -> (w272:path)
                    n1018 = Build Array(w261, w269, w268, w266, w265, w264, w264, w264, w264, w264, w264, w263, w262) -> (w271:dbl[])
                    n1019 = case shown="False" w276 {
                      frame False {
                        n1020 = local read "water dur (ms) 4.1"() -> (w277:dbl)
                        n1021 = local read "water port 4.1"() -> (w278:tag)
                        n1022 = call "_digital_on_duration_off.vi"("duration (ms)"=w277, "digital port"=w278) -> ()  [unwired: 10 in]
                      }
                      frame True {
                      }
                    }
                    n1023 = call-poly <vilib>:"Write To Spreadsheet File.vi"("append to file? (new file:F)"=TRUE, "1D data"=w271, "file path (dialog if empty)"=w272) -> ()  [unwired: 5 in, 1 out]
                  }
                  frame "sound" {
                    w281 = 0.0 ("element")
                    n1024 = local read "water # 4.1L"() -> (w283:dbl)
                    n1025 = local read "water # 4.2R"() -> (w282:dbl)
                    n1026 = local read "lick # 4.2R"() -> (w284:dbl)
                    n1027 = local read "lick # 4.1L"() -> (w286:dbl)
                    n1028 = local read "mistake # 4.2R"() -> (w279:dbl)
                    n1029 = local read "mistake # 4.1L"() -> (w280:dbl)
                    n1030 = Increment(x=w286) -> (x+1=w285:dbl)
                    n1031 = local read "time (s)"() -> (w287:dbl)
                    n1032 = local write "lick # 4.1L"(w285) -> ()
                    n1033 = Build Array(w287, w285, w284, w283, w282, w281, w281, w281, w281, w281, w281, w280, w279) -> (w288:dbl[])
                    n1034 = local read "Mouse path 4"() -> (w289:path)
                    n1035 = call-poly <vilib>:"Write To Spreadsheet File.vi"("append to file? (new file:F)"=TRUE, "1D data"=w288, "file path (dialog if empty)"=w289) -> ()  [unwired: 5 in, 1 out]
                  }
                  frame "ITI" {
                    w293 = 0.0 ("element")
                    n1036 = local read "water # 4.2R"() -> (w294:dbl)
                    n1037 = local read "lick # 4.2R"() -> (w296:dbl)
                    n1038 = local read "water # 4.1L"() -> (w295:dbl)
                    n1039 = local read "lick # 4.1L"() -> (w298:dbl)
                    n1040 = local read "mistake # 4.1L"() -> (w292:dbl)
                    n1041 = local read "mistake # 4.2R"() -> (w291:dbl)
                    n1042 = Increment(x=w298) -> (x+1=w297:dbl)
                    n1043 = local read "time (s)"() -> (w299:dbl)
                    n1044 = local write "lick # 4.1L"(w297) -> ()
                    n1045 = local read "Mouse path 4"() -> (w301:path)
                    n1046 = Build Array(w299, w297, w296, w295, w294, w293, w293, w293, w293, w293, w293, w292, w291) -> (w300:dbl[])
                    n1047 = call-poly <vilib>:"Write To Spreadsheet File.vi"("append to file? (new file:F)"=TRUE, "1D data"=w300, "file path (dialog if empty)"=w301) -> ()  [unwired: 5 in, 1 out]
                  }
                }
              }
            }
          }
          frame 4 {
            n1048 = case shown="True" w343 {
              frame False {
              }
              frame True {
                n1049 = local read "state 4.2"() -> (w385:enum16{"waiting", "sound", "ITI"})
                n1050 = case shown="\"waiting\", Default" w385 {
                  frame "waiting", Default {
                    w389 = 0.0 ("element")
                    n1051 = local read "water # 4.2R"() -> (w391:dbl)
                    n1052 = local read "lick # 4.2R"() -> (w394:dbl)
                    n1053 = local read "water # 4.1L"() -> (w392:dbl)
                    n1054 = local read "lick # 4.1L"() -> (w395:dbl)
                    n1055 = local read "mistake # 4.2R"() -> (w387:dbl)
                    n1056 = local read "time (s)"() -> (w386:dbl)
                    n1057 = local read "mistake # 4.1L"() -> (w388:dbl)
                    n1058 = Increment(x=w394) -> (x+1=w393:dbl)
                    n1059 = Increment(x=w391) -> (x+1=w390:dbl)
                    n1060 = local write "state 4.2"(enum16{"waiting", "sound", "ITI"}."ITI") -> ()
                    n1061 = local write "water # 4.2R"(w390) -> ()
                    n1062 = local write "lick # 4.2R"(w393) -> ()
                    n1063 = local write "last water 4.2R"(w386) -> ()
                    n1064 = local read "Mouse path 4"() -> (w397:path)
                    n1065 = local write "state 4.1"(enum16{"waiting", "sound", "ITI"}."ITI") -> ()
                    n1066 = local read "free water 4.2"() -> (w399:bool)
                    n1067 = Build Array(w386, w395, w393, w392, w390, w389, w389, w389, w389, w389, w389, w388, w387) -> (w396:dbl[])
                    n1068 = call-poly <vilib>:"Write To Spreadsheet File.vi"("append to file? (new file:F)"=TRUE, "1D data"=w396, "file path (dialog if empty)"=w397) -> ()  [unwired: 5 in, 1 out]
                    n1069 = case shown="False" w399 {
                      frame False {
                        n1070 = local read "water dur (ms) 4.2"() -> (w402:dbl)
                        n1071 = local read "water port 4.2"() -> (w403:tag)
                        n1072 = call "_digital_on_duration_off.vi"("duration (ms)"=w402, "digital port"=w403) -> ()  [unwired: 10 in]
                      }
                      frame True {
                      }
                    }
                  }
                  frame "sound" {
                    w406 = 0.0 ("element")
                    n1073 = local read "water # 4.2R"() -> (w407:dbl)
                    n1074 = local read "water # 4.1L"() -> (w408:dbl)
                    n1075 = local read "lick # 4.2R"() -> (w410:dbl)
                    n1076 = local read "lick # 4.1L"() -> (w411:dbl)
                    n1077 = local read "mistake # 4.2R"() -> (w404:dbl)
                    n1078 = local read "mistake # 4.1L"() -> (w405:dbl)
                    n1079 = Increment(x=w410) -> (x+1=w409:dbl)
                    n1080 = local write "lick # 4.2R"(w409) -> ()
                    n1081 = local read "time (s)"() -> (w412:dbl)
                    n1082 = Build Array(w412, w411, w409, w408, w407, w406, w406, w406, w406, w406, w406, w405, w404) -> (w413:dbl[])
                    n1083 = local read "Mouse path 4"() -> (w414:path)
                    n1084 = call-poly <vilib>:"Write To Spreadsheet File.vi"("append to file? (new file:F)"=TRUE, "1D data"=w413, "file path (dialog if empty)"=w414) -> ()  [unwired: 5 in, 1 out]
                  }
                  frame "ITI" {
                    w418 = 0.0 ("element")
                    n1085 = local read "water # 4.2R"() -> (w419:dbl)
                    n1086 = local read "lick # 4.2R"() -> (w422:dbl)
                    n1087 = local read "water # 4.1L"() -> (w420:dbl)
                    n1088 = local read "lick # 4.1L"() -> (w423:dbl)
                    n1089 = local read "mistake # 4.2R"() -> (w416:dbl)
                    n1090 = local read "mistake # 4.1L"() -> (w417:dbl)
                    n1091 = Increment(x=w422) -> (x+1=w421:dbl)
                    n1092 = local read "time (s)"() -> (w424:dbl)
                    n1093 = local write "lick # 4.2R"(w421) -> ()
                    n1094 = Build Array(w424, w423, w421, w420, w419, w418, w418, w418, w418, w418, w418, w417, w416) -> (w425:dbl[])
                    n1095 = local read "Mouse path 4"() -> (w426:path)
                    n1096 = call-poly <vilib>:"Write To Spreadsheet File.vi"("append to file? (new file:F)"=TRUE, "1D data"=w425, "file path (dialog if empty)"=w426) -> ()  [unwired: 5 in, 1 out]
                  }
                }
              }
            }
            n1097 = case shown="True" w344 {
              frame False {
              }
              frame True {
                n1098 = local read "state 4.2"() -> (w345:enum16{"waiting", "sound", "ITI"})
                n1099 = case shown="\"ITI\"" w345 {
                  frame "waiting", Default {
                    w349 = 0.0 ("element")
                    n1100 = local read "water # 4.2R"() -> (w350:dbl)
                    n1101 = local read "water # 4.1L"() -> (w351:dbl)
                    n1102 = local read "lick # 4.2R"() -> (w352:dbl)
                    n1103 = local read "lick # 4.1L"() -> (w354:dbl)
                    n1104 = local read "mistake # 4.2R"() -> (w347:dbl)
                    n1105 = local read "mistake # 4.1L"() -> (w348:dbl)
                    n1106 = local read "time (s)"() -> (w355:dbl)
                    n1107 = Increment(x=w354) -> (x+1=w353:dbl)
                    n1108 = Increment(x=w347) -> (x+1=w346:dbl)
                    n1109 = local write "lick # 4.1L"(w353) -> ()
                    n1110 = local write "mistake # 4.2R"(w346) -> ()
                    n1111 = local read "Mouse path 4"() -> (w357:path)
                    n1112 = Build Array(w355, w353, w352, w351, w350, w349, w349, w349, w349, w349, w348, w346) -> (w356:dbl[])
                    n1113 = local write "state 4.1"(enum16{"waiting", "sound", "ITI"}."ITI") -> ()
                    n1114 = local write "state 4.2"(enum16{"waiting", "sound", "ITI"}."ITI") -> ()
                    n1115 = call-poly <vilib>:"Write To Spreadsheet File.vi"("append to file? (new file:F)"=TRUE, "1D data"=w356, "file path (dialog if empty)"=w357) -> ()  [unwired: 5 in, 1 out]
                  }
                  frame "sound" {
                    w363 = 0.0 ("element")
                    n1116 = local read "lick # 4.2R"() -> (w366:dbl)
                    n1117 = local read "water # 4.2R"() -> (w364:dbl)
                    n1118 = local read "water # 4.1L"() -> (w365:dbl)
                    n1119 = local read "lick # 4.1L"() -> (w368:dbl)
                    n1120 = local read "mistake # 4.2R"() -> (w361:dbl)
                    n1121 = local read "mistake # 4.1L"() -> (w362:dbl)
                    n1122 = local read "time (s)"() -> (w369:dbl)
                    n1123 = Increment(x=w368) -> (x+1=w367:dbl)
                    n1124 = local write "lick # 4.1L"(w367) -> ()
                    n1125 = local read "Mouse path 4"() -> (w371:path)
                    n1126 = Build Array(w369, w367, w366, w365, w364, w363, w363, w363, w363, w363, w363, w362, w361) -> (w370:dbl[])
                    n1127 = call-poly <vilib>:"Write To Spreadsheet File.vi"("append to file? (new file:F)"=TRUE, "1D data"=w370, "file path (dialog if empty)"=w371) -> ()  [unwired: 5 in, 1 out]
                  }
                  frame "ITI" {
                    w375 = 0.0 ("element")
                    n1128 = local read "water # 4.2R"() -> (w376:dbl)
                    n1129 = local read "water # 4.1L"() -> (w377:dbl)
                    n1130 = local read "lick # 4.2R"() -> (w378:dbl)
                    n1131 = local read "lick # 4.1L"() -> (w380:dbl)
                    n1132 = local read "mistake # 4.1L"() -> (w374:dbl)
                    n1133 = local read "mistake # 4.2R"() -> (w373:dbl)
                    n1134 = local read "time (s)"() -> (w381:dbl)
                    n1135 = Increment(x=w380) -> (x+1=w379:dbl)
                    n1136 = local write "lick # 4.1L"(w379) -> ()
                    n1137 = local read "Mouse path 4"() -> (w383:path)
                    n1138 = Build Array(w381, w379, w378, w377, w376, w375, w375, w375, w375, w375, w375, w374, w373) -> (w382:dbl[])
                    n1139 = call-poly <vilib>:"Write To Spreadsheet File.vi"("append to file? (new file:F)"=TRUE, "1D data"=w382, "file path (dialog if empty)"=w383) -> ()  [unwired: 5 in, 1 out]
                  }
                }
              }
            }
          }
        }
        n1140 = case shown="1" w70 {
          tunnel: w72 -> [_ w1109 w1214 w1321 w1425]
          tunnel: w71 -> [_ w1108 w1215 w1320 w1424]
          frame 0, Default {
          }
          frame 1 {
            n1141 = case shown="True" w1108 {
              frame False {
              }
              frame True {
                n1142 = local read "state 1.1"() -> (w1110:enum16{"waiting", "sound", "ITI"})
                n1143 = case shown="\"waiting\", Default" w1110 {
                  frame "waiting", Default {
                    w1119 = 0
                    n1144 = local read "water # 1.2R"() -> (w1113:dbl)
                    n1145 = local read "lick # 1.2R"() -> (w1123:dbl)
                    n1146 = local read "lick # 1.1L"() -> (w1122:dbl)
                    n1147 = local read "water # 1.1L"() -> (w1125:dbl)
                    n1148 = local read "current sound"() -> (w1127:dbl)
                    n1149 = local read "time (s)"() -> (w1121:dbl)
                    n1150 = local read "trial #"() -> (w1126:dbl)
                    n1151 = local read "mistake # 1.1L"() -> (w1115:dbl)
                    n1152 = Increment(x=w1123) -> (x+1=w1124:dbl)
                    n1153 = local read "mistake # 1.2R"() -> (w1117:dbl)
                    n1154 = local write "lick # 1.2R"(w1124) -> ()
                    n1155 = local write "state 1.2"(enum16{"waiting", "sound", "ITI"}."ITI") -> ()
                    n1156 = local write "state 1.1"(enum16{"waiting", "sound", "ITI"}."ITI") -> ()
                    n1157 = local read "ITI (s)"() -> (w1128:dbl)
                    n1158 = Increment(x=w1115) -> (x+1=w1114:dbl)
                    n1159 = local read "Mouse path 1"() -> (w1118:path)
                    n1160 = local write "mistake # 1.1L"(w1114) -> ()
                    n1161 = Build Array(w1121, w1122, w1124, w1125, w1113, 0.0 ("element"), w1119, w1126, w1127, w1128, w1119, w1114, w1117) -> (w1129:dbl[])
                    n1162 = call-poly <vilib>:"Write To Spreadsheet File.vi"("append to file? (new file:F)"=TRUE, "1D data"=w1129, "file path (dialog if empty)"=w1118) -> ()  [unwired: 5 in, 1 out]
                  }
                  frame "ITI" {
                    w1132 = 0 ("element")
                    n1163 = local read "lick # 1.2R"() -> (w1139:dbl)
                    n1164 = local read "water # 1.1L"() -> (w1137:dbl)
                    n1165 = local read "water # 1.2R"() -> (w1136:dbl)
                    n1166 = local read "lick # 1.1L"() -> (w1140:dbl)
                    n1167 = local read "mistake # 1.2R"() -> (w1130:dbl)
                    n1168 = local read "current sound"() -> (w1134:dbl)
                    n1169 = local read "mistake # 1.1L"() -> (w1131:dbl)
                    n1170 = local read "time (s)"() -> (w1141:dbl)
                    n1171 = local read "trial #"() -> (w1135:dbl)
                    n1172 = local read "ITI (s)"() -> (w1133:dbl)
                    n1173 = Increment(x=w1139) -> (x+1=w1138:dbl)
                    n1174 = local write "lick # 1.2R"(w1138) -> ()
                    n1175 = local read "Mouse path 1"() -> (w1144:path)
                    n1176 = Build Array(w1141, w1140, w1138, w1137, w1136, w1132, w1132, w1135, w1134, w1133, w1132, w1131, w1130) -> (w1142:dbl[])
                    n1177 = call-poly <vilib>:"Write To Spreadsheet File.vi"("append to file? (new file:F)"=TRUE, "1D data"=w1142, "file path (dialog if empty)"=w1144) -> ()  [unwired: 5 in, 1 out]
                  }
                  frame "sound" {
                    w1147 = 0 ("element")
                    n1178 = local read "water # 1.2R"() -> (w1151:dbl)
                    n1179 = local read "water # 1.1L"() -> (w1152:dbl)
                    n1180 = local read "lick # 1.2R"() -> (w1154:dbl)
                    n1181 = local read "lick # 1.1L"() -> (w1155:dbl)
                    n1182 = Increment(x=w1154) -> (x+1=w1153:dbl)
                    n1183 = local read "mistake # 1.2R"() -> (w1145:dbl)
                    n1184 = local read "mistake # 1.1L"() -> (w1146:dbl)
                    n1185 = local read "current sound"() -> (w1149:dbl)
                    n1186 = local read "time (s)"() -> (w1156:dbl)
                    n1187 = local write "lick # 1.2R"(w1153) -> ()
                    n1188 = local read "ITI (s)"() -> (w1148:dbl)
                    n1189 = local read "trial #"() -> (w1150:dbl)
                    n1190 = local read "Mouse path 1"() -> (w1159:path)
                    n1191 = Build Array(w1156, w1155, w1153, w1152, w1151, w1147, w1147, w1150, w1149, w1148, w1147, w1146, w1145) -> (w1157:dbl[])
                    n1192 = call-poly <vilib>:"Write To Spreadsheet File.vi"("append to file? (new file:F)"=TRUE, "1D data"=w1157, "file path (dialog if empty)"=w1159) -> ()  [unwired: 5 in, 1 out]
                  }
                }
              }
            }
            n1193 = case shown="True" w1109 {
              frame False {
              }
              frame True {
                n1194 = local read "Mouse path 1"() -> (w1160:path)
                n1195 = local read "state 1.1"() -> (w1161:enum16{"waiting", "sound", "ITI"})
                n1196 = case shown="\"waiting\", Default" w1161 {
                  tunnel: w1160 -> [w1168 _ w1201]
                  frame "waiting", Default {
                    w1173 = 0
                    n1197 = local read "time (s)"() -> (w1180:dbl)
                    n1198 = local read "lick # 1.1L"() -> (w1179:dbl)
                    n1199 = local read "water # 1.1L"() -> (w1178:dbl)
                    n1200 = local write "state 1.2"(enum16{"waiting", "sound", "ITI"}."ITI") -> ()
                    n1201 = local write "state 1.1"(enum16{"waiting", "sound", "ITI"}."ITI") -> ()
                    n1202 = local write "last water 1.1L"(w1180) -> ()
                    n1203 = Increment(x=w1178) -> (x+1=w1176:dbl)
                    n1204 = Increment(x=w1179) -> (x+1=w1177:dbl)
                    n1205 = local write "lick # 1.1L"(w1177) -> ()
                    n1206 = local write "water # 1.1L"(w1176) -> ()
                    n1207 = local read "lick # 1.2R"() -> (w1167:dbl)
                    n1208 = local read "free water 1.1"() -> (w1164:bool)
                    n1209 = local read "current sound"() -> (w1171:dbl)
                    n1210 = local read "trial #"() -> (w1172:dbl)
                    n1211 = local read "water # 1.2R"() -> (w1175:dbl)
                    n1212 = case shown="False" w1164 {
                      frame False {
                        n1213 = call "_digital_on_duration_off.vi"("duration (ms)"="water dur (ms) 1.1", "digital port"="water port 1.1") -> ()  [unwired: 10 in]
                      }
                      frame True {
                      }
                    }
                    n1214 = local read "ITI (s)"() -> (w1170:dbl)
                    n1215 = local read "mistake # 1.1L"() -> (w1166:dbl)
                    n1216 = local read "mistake # 1.2R"() -> (w1165:dbl)
                    n1217 = Build Array(w1180, w1177, w1167, w1176, w1175, 1, w1173, w1172, w1171, w1170, w1173, w1166, w1165) -> (w1169:dbl[])
                    n1218 = call-poly <vilib>:"Write To Spreadsheet File.vi"("append to file? (new file:F)"=TRUE, "1D data"=w1169, "file path (dialog if empty)"=w1168) -> ()  [unwired: 5 in, 1 out]
                  }
                  frame "sound" {
                    w1186 = 0 ("element")
                    n1219 = local read "mistake # 1.2R"() -> (w1184:dbl)
                    n1220 = local read "water # 1.2R"() -> (w1190:dbl)
                    n1221 = local read "water # 1.1L"() -> (w1191:dbl)
                    n1222 = local read "mistake # 1.1L"() -> (w1185:dbl)
                    n1223 = local read "current sound"() -> (w1188:dbl)
                    n1224 = local read "trial #"() -> (w1189:dbl)
                    n1225 = local read "lick # 1.2R"() -> (w1192:dbl)
                    n1226 = local read "lick # 1.1L"() -> (w1194:dbl)
                    n1227 = local read "ITI (s)"() -> (w1187:dbl)
                    n1228 = Increment(x=w1194) -> (x+1=w1193:dbl)
                    n1229 = local read "time (s)"() -> (w1195:dbl)
                    n1230 = local write "lick # 1.1L"(w1193) -> ()
                    n1231 = local read "Mouse path 1"() -> (w1197:path)
                    n1232 = Build Array(w1195, w1193, w1192, w1191, w1190, w1186, w1186, w1189, w1188, w1187, w1186, w1185, w1184) -> (w1196:dbl[])
                    n1233 = call-poly <vilib>:"Write To Spreadsheet File.vi"("append to file? (new file:F)"=TRUE, "1D data"=w1196, "file path (dialog if empty)"=w1197) -> ()  [unwired: 5 in, 1 out]
                  }
                  frame "ITI" {
                    w1207 = 0
                    n1234 = local read "time (s)"() -> (w1212:dbl)
                    n1235 = local read "lick # 1.1L"() -> (w1211:dbl)
                    n1236 = local read "lick # 1.2R"() -> (w1202:dbl)
                    n1237 = Increment(x=w1211) -> (x+1=w1210:dbl)
                    n1238 = local read "water # 1.1L"() -> (w1209:dbl)
                    n1239 = local read "water # 1.2R"() -> (w1208:dbl)
                    n1240 = local write "lick # 1.1L"(w1210) -> ()
                    n1241 = local read "current sound"() -> (w1205:dbl)
                    n1242 = local read "ITI (s)"() -> (w1204:dbl)
                    n1243 = local read "trial #"() -> (w1206:dbl)
                    n1244 = local read "mistake # 1.2R"() -> (w1199:dbl)
                    n1245 = local read "mistake # 1.1L"() -> (w1200:dbl)
                    n1246 = Build Array(w1212, w1210, w1202, w1209, w1208, w1207, w1207, w1206, w1205, w1204, w1207, w1200, w1199) -> (w1203:dbl[])
                    n1247 = call-poly <vilib>:"Write To Spreadsheet File.vi"("append to file? (new file:F)"=TRUE, "1D data"=w1203, "file path (dialog if empty)"=w1201) -> ()  [unwired: 5 in, 1 out]
                  }
                }
              }
            }
          }
          frame 2 {
            n1248 = case shown="True" w1214 {
              frame False {
              }
              frame True {
                n1249 = local read "state 1.2"() -> (w1216:enum16{"waiting", "sound", "ITI"})
                n1250 = case shown="\"waiting\", Default" w1216 {
                  frame "waiting", Default {
                    w1223 = 0
                    n1251 = local read "water # 1.1L"() -> (w1217:dbl)
                    n1252 = local read "lick # 1.2R"() -> (w1229:dbl)
                    n1253 = local read "water # 1.2R"() -> (w1230:dbl)
                    n1254 = local read "time (s)"() -> (w1226:dbl)
                    n1255 = local read "current sound"() -> (w1232:dbl)
                    n1256 = local read "lick # 1.1L"() -> (w1227:dbl)
                    n1257 = local write "state 1.2"(enum16{"waiting", "sound", "ITI"}."ITI") -> ()
                    n1258 = local write "state 1.1"(enum16{"waiting", "sound", "ITI"}."ITI") -> ()
                    n1259 = local read "mistake # 1.2R"() -> (w1220:dbl)
                    n1260 = local read "ITI (s)"() -> (w1233:dbl)
                    n1261 = Increment(x=w1227) -> (x+1=w1228:dbl)
                    n1262 = local write "lick # 1.1L"(w1228) -> ()
                    n1263 = local read "mistake # 1.1L"() -> (w1222:dbl)
                    n1264 = local read "trial #"() -> (w1231:dbl)
                    n1265 = Increment(x=w1220) -> (x+1=w1219:dbl)
                    n1266 = local read "Mouse path 1"() -> (w1235:path)
                    n1267 = local write "mistake # 1.2R"(w1219) -> ()
                    n1268 = Build Array(w1226, w1228, w1229, w1217, w1230, 0.0 ("element"), w1223, w1231, w1232, w1233, w1223, w1222, w1219) -> (w1234:dbl[])
                    n1269 = call-poly <vilib>:"Write To Spreadsheet File.vi"("append to file? (new file:F)"=TRUE, "1D data"=w1234, "file path (dialog if empty)"=w1235) -> ()  [unwired: 5 in, 1 out]
                  }
                  frame "ITI" {
                    w1238 = 0 ("element")
                    n1270 = local read "lick # 1.1L"() -> (w1246:dbl)
                    n1271 = local read "water # 1.2R"() -> (w1242:dbl)
                    n1272 = local read "water # 1.1L"() -> (w1243:dbl)
                    n1273 = local read "lick # 1.2R"() -> (w1244:dbl)
                    n1274 = local read "mistake # 1.2R"() -> (w1236:dbl)
                    n1275 = local read "current sound"() -> (w1240:dbl)
                    n1276 = local read "mistake # 1.1L"() -> (w1237:dbl)
                    n1277 = local read "trial #"() -> (w1241:dbl)
                    n1278 = Increment(x=w1246) -> (x+1=w1245:dbl)
                    n1279 = local read "time (s)"() -> (w1247:dbl)
                    n1280 = local read "ITI (s)"() -> (w1239:dbl)
                    n1281 = local write "lick # 1.1L"(w1245) -> ()
                    n1282 = Build Array(w1247, w1245, w1244, w1243, w1242, w1238, w1238, w1241, w1240, w1239, w1238, w1237, w1236) -> (w1248:dbl[])
                    n1283 = local read "Mouse path 1"() -> (w1250:path)
                    n1284 = call-poly <vilib>:"Write To Spreadsheet File.vi"("append to file? (new file:F)"=TRUE, "1D data"=w1248, "file path (dialog if empty)"=w1250) -> ()  [unwired: 5 in, 1 out]
                  }
                  frame "sound" {
                    w1253 = 0 ("element")
                    n1285 = local read "water # 1.2R"() -> (w1257:dbl)
                    n1286 = local read "water # 1.1L"() -> (w1258:dbl)
                    n1287 = local read "lick # 1.2R"() -> (w1259:dbl)
                    n1288 = local read "mistake # 1.2R"() -> (w1251:dbl)
                    n1289 = local read "mistake # 1.1L"() -> (w1252:dbl)
                    n1290 = local read "current sound"() -> (w1255:dbl)
                    n1291 = local read "lick # 1.1L"() -> (w1261:dbl)
                    n1292 = local read "trial #"() -> (w1256:dbl)
                    n1293 = local read "ITI (s)"() -> (w1254:dbl)
                    n1294 = local read "time (s)"() -> (w1262:dbl)
                    n1295 = Increment(x=w1261) -> (x+1=w1260:dbl)
                    n1296 = local write "lick # 1.1L"(w1260) -> ()
                    n1297 = local read "Mouse path 1"() -> (w1265:path)
                    n1298 = Build Array(w1262, w1260, w1259, w1258, w1257, w1253, w1253, w1256, w1255, w1254, w1253, w1252, w1251) -> (w1263:dbl[])
                    n1299 = call-poly <vilib>:"Write To Spreadsheet File.vi"("append to file? (new file:F)"=TRUE, "1D data"=w1263, "file path (dialog if empty)"=w1265) -> ()  [unwired: 5 in, 1 out]
                  }
                }
              }
            }
            n1300 = case shown="True" w1215 {
              frame False {
              }
              frame True {
                n1301 = local read "Mouse path 1"() -> (w1266:path)
                n1302 = local read "state 1.2"() -> (w1267:enum16{"waiting", "sound", "ITI"})
                n1303 = case shown="\"waiting\", Default" w1267 {
                  tunnel: w1266 -> [w1275 _ w1307]
                  frame "waiting", Default {
                    w1281 = 0
                    n1304 = local read "lick # 1.1L"() -> (w1274:dbl)
                    n1305 = local read "lick # 1.2R"() -> (w1273:dbl)
                    n1306 = local read "time (s)"() -> (w1286:dbl)
                    n1307 = local read "water # 1.2R"() -> (w1284:dbl)
                    n1308 = Increment(x=w1273) -> (x+1=w1272:dbl)
                    n1309 = local write "last water 1.2R"(w1286) -> ()
                    n1310 = local write "lick # 1.2R"(w1272) -> ()
                    n1311 = Increment(x=w1284) -> (x+1=w1283:dbl)
                    n1312 = local read "free water 1.2"() -> (w1269:bool)
                    n1313 = local write "water # 1.2R"(w1283) -> ()
                    n1314 = case shown="False" w1269 {
                      frame False {
                        n1315 = call "_digital_on_duration_off.vi"("duration (ms)"="water dur (ms) 1.2", "digital port"="water port 1.2") -> ()  [unwired: 10 in]
                      }
                      frame True {
                      }
                    }
                    n1316 = local read "water # 1.1L"() -> (w1285:dbl)
                    n1317 = local read "current sound"() -> (w1279:dbl)
                    n1318 = local read "trial #"() -> (w1280:dbl)
                    n1319 = local read "mistake # 1.2R"() -> (w1270:dbl)
                    n1320 = local read "mistake # 1.1L"() -> (w1271:dbl)
                    n1321 = local read "ITI (s)"() -> (w1278:dbl)
                    n1322 = Build Array(w1286, w1274, w1272, w1285, w1283, 1, w1281, w1280, w1279, w1278, w1281, w1271, w1270) -> (w1277:dbl[])
                    n1323 = local write "state 1.1"(enum16{"waiting", "sound", "ITI"}."ITI") -> ()
                    n1324 = local write "state 1.2"(enum16{"waiting", "sound", "ITI"}."ITI") -> ()
                    n1325 = call-poly <vilib>:"Write To Spreadsheet File.vi"("append to file? (new file:F)"=TRUE, "1D data"=w1277, "file path (dialog if empty)"=w1275) -> ()  [unwired: 5 in, 1 out]
                  }
                  frame "sound" {
                    w1292 = 0 ("element")
                    n1326 = local read "water # 1.2R"() -> (w1296:dbl)
                    n1327 = local read "water # 1.1L"() -> (w1297:dbl)
                    n1328 = local read "lick # 1.1L"() -> (w1299:dbl)
                    n1329 = local read "lick # 1.2R"() -> (w1300:dbl)
                    n1330 = local read "current sound"() -> (w1294:dbl)
                    n1331 = local read "mistake # 1.1L"() -> (w1291:dbl)
                    n1332 = local read "ITI (s)"() -> (w1293:dbl)
                    n1333 = local read "mistake # 1.2R"() -> (w1290:dbl)
                    n1334 = local read "trial #"() -> (w1295:dbl)
                    n1335 = local read "time (s)"() -> (w1301:dbl)
                    n1336 = Increment(x=w1300) -> (x+1=w1298:dbl)
                    n1337 = local write "lick # 1.2R"(w1298) -> ()
                    n1338 = local read "Mouse path 1"() -> (w1304:path)
                    n1339 = Build Array(w1301, w1299, w1298, w1297, w1296, w1292, w1292, w1295, w1294, w1293, w1292, w1291, w1290) -> (w1302:dbl[])
                    n1340 = call-poly <vilib>:"Write To Spreadsheet File.vi"("append to file? (new file:F)"=TRUE, "1D data"=w1302, "file path (dialog if empty)"=w1304) -> ()  [unwired: 5 in, 1 out]
                  }
                  frame "ITI" {
                    w1313 = 0
                    n1341 = local read "lick # 1.1L"() -> (w1308:dbl)
                    n1342 = local read "lick # 1.2R"() -> (w1317:dbl)
                    n1343 = local read "time (s)"() -> (w1318:dbl)
                    n1344 = Increment(x=w1317) -> (x+1=w1316:dbl)
                    n1345 = local write "lick # 1.2R"(w1316) -> ()
                    n1346 = local read "water # 1.1L"() -> (w1315:dbl)
                    n1347 = local read "current sound"() -> (w1311:dbl)
                    n1348 = local read "water # 1.2R"() -> (w1314:dbl)
                    n1349 = local read "trial #"() -> (w1312:dbl)
                    n1350 = local read "mistake # 1.1L"() -> (w1306:dbl)
                    n1351 = local read "mistake # 1.2R"() -> (w1305:dbl)
                    n1352 = local read "ITI (s)"() -> (w1310:dbl)
                    n1353 = Build Array(w1318, w1308, w1316, w1315, w1314, w1313, w1313, w1312, w1311, w1310, w1313, w1306, w1305) -> (w1309:dbl[])
                    n1354 = call-poly <vilib>:"Write To Spreadsheet File.vi"("append to file? (new file:F)"=TRUE, "1D data"=w1309, "file path (dialog if empty)"=w1307) -> ()  [unwired: 5 in, 1 out]
                  }
                }
              }
            }
          }
          frame 3 {
            n1355 = case shown="True" w1321 {
              frame False {
              }
              frame True {
                n1356 = local read "state 1.1"() -> (w1371:enum16{"waiting", "sound", "ITI"})
                n1357 = case shown="\"waiting\", Default" w1371 {
                  frame "waiting", Default {
                    w1376 = 0 ("element")
                    n1358 = local read "water # 1.2R"() -> (w1381:dbl)
                    n1359 = local read "water # 1.1L"() -> (w1383:dbl)
                    n1360 = local read "lick # 1.2R"() -> (w1384:dbl)
                    n1361 = local read "lick # 1.1L"() -> (w1386:dbl)
                    n1362 = local read "time (s)"() -> (w1387:dbl)
                    n1363 = Increment(x=w1383) -> (x+1=w1382:dbl)
                    n1364 = Increment(x=w1386) -> (x+1=w1385:dbl)
                    n1365 = local write "state 1.1"(enum16{"waiting", "sound", "ITI"}."ITI") -> ()
                    n1366 = local write "water # 1.1L"(w1382) -> ()
                    n1367 = local read "Mouse path 1"() -> (w1389:path)
                    n1368 = local write "lick # 1.1L"(w1385) -> ()
                    n1369 = local write "last water 1.1L"(w1387) -> ()
                    n1370 = local read "current sound"() -> (w1378:dbl)
                    n1371 = local read "mistake # 1.2R"() -> (w1374:dbl)
                    n1372 = local read "mistake # 1.1L"() -> (w1375:dbl)
                    n1373 = local read "ITI (s)"() -> (w1377:dbl)
                    n1374 = local read "trial #"() -> (w1379:dbl)
                    n1375 = local read "free water 1.1"() -> (w1372:bool)
                    n1376 = local write "state 1.2"(enum16{"waiting", "sound", "ITI"}."ITI") -> ()
                    n1377 = case shown="False" w1372 {
                      frame False {
                        n1378 = local read "water port 1.1"() -> (w1392:tag)
                        n1379 = local read "water dur (ms) 1.1"() -> (w1393:dbl)
                        n1380 = call "_digital_on_duration_off.vi"("duration (ms)"=w1393, "digital port"=w1392) -> ()  [unwired: 10 in]
                      }
                      frame True {
                      }
                    }
                    n1381 = Build Array(w1387, w1385, w1384, w1382, w1381, 1 ("element"), w1376, w1379, w1378, w1377, w1376, w1375, w1374) -> (w1388:dbl[])
                    n1382 = call-poly <vilib>:"Write To Spreadsheet File.vi"("append to file? (new file:F)"=TRUE, "1D data"=w1388, "file path (dialog if empty)"=w1389) -> ()  [unwired: 5 in, 1 out]
                  }
                  frame "ITI" {
                    w1396 = 0 ("element")
                    n1383 = local read "water # 1.2R"() -> (w1400:dbl)
                    n1384 = local read "water # 1.1L"() -> (w1401:dbl)
                    n1385 = local read "lick # 1.1L"() -> (w1404:dbl)
                    n1386 = local read "lick # 1.2R"() -> (w1402:dbl)
                    n1387 = local read "current sound"() -> (w1398:dbl)
                    n1388 = local read "trial #"() -> (w1399:dbl)
                    n1389 = local read "ITI (s)"() -> (w1397:dbl)
                    n1390 = local read "time (s)"() -> (w1405:dbl)
                    n1391 = Increment(x=w1404) -> (x+1=w1403:dbl)
                    n1392 = local read "mistake # 1.1L"() -> (w1395:dbl)
                    n1393 = local read "mistake # 1.2R"() -> (w1394:dbl)
                    n1394 = local write "lick # 1.1L"(w1403) -> ()
                    n1395 = local read "Mouse path 1"() -> (w1408:path)
                    n1396 = Build Array(w1405, w1403, w1402, w1401, w1400, w1396, w1396, w1399, w1398, w1397, w1396, w1395, w1394) -> (w1406:dbl[])
                    n1397 = call-poly <vilib>:"Write To Spreadsheet File.vi"("append to file? (new file:F)"=TRUE, "1D data"=w1406, "file path (dialog if empty)"=w1408) -> ()  [unwired: 5 in, 1 out]
                  }
                  frame "sound" {
                    w1411 = 0 ("element")
                    n1398 = local read "water # 1.2R"() -> (w1415:dbl)
                    n1399 = local read "water # 1.1L"() -> (w1416:dbl)
                    n1400 = local read "lick # 1.2R"() -> (w1417:dbl)
                    n1401 = local read "lick # 1.1L"() -> (w1419:dbl)
                    n1402 = local read "current sound"() -> (w1413:dbl)
                    n1403 = local read "mistake # 1.2R"() -> (w1409:dbl)
                    n1404 = local read "ITI (s)"() -> (w1412:dbl)
                    n1405 = local read "trial #"() -> (w1414:dbl)
                    n1406 = local read "mistake # 1.1L"() -> (w1410:dbl)
                    n1407 = local read "time (s)"() -> (w1420:dbl)
                    n1408 = Increment(x=w1419) -> (x+1=w1418:dbl)
                    n1409 = local write "lick # 1.1L"(w1418) -> ()
                    n1410 = local read "Mouse path 1"() -> (w1423:path)
                    n1411 = Build Array(w1420, w1418, w1417, w1416, w1415, w1411, w1411, w1414, w1413, w1412, w1411, w1410, w1409) -> (w1421:dbl[])
                    n1412 = call-poly <vilib>:"Write To Spreadsheet File.vi"("append to file? (new file:F)"=TRUE, "1D data"=w1421, "file path (dialog if empty)"=w1423) -> ()  [unwired: 5 in, 1 out]
                  }
                }
              }
            }
            n1413 = case shown="True" w1320 {
              frame False {
              }
              frame True {
                n1414 = local read "state 1.1"() -> (w1322:enum16{"waiting", "sound", "ITI"})
                n1415 = case shown="\"waiting\", Default" w1322 {
                  frame "waiting", Default {
                    w1327 = 0 ("element")
                    n1416 = local read "water # 1.2R"() -> (w1331:dbl)
                    n1417 = local read "water # 1.1L"() -> (w1332:dbl)
                    n1418 = local read "lick # 1.2R"() -> (w1334:dbl)
                    n1419 = local read "lick # 1.1L"() -> (w1335:dbl)
                    n1420 = local read "current sound"() -> (w1329:dbl)
                    n1421 = local read "mistake # 1.1L"() -> (w1325:dbl)
                    n1422 = Increment(x=w1334) -> (x+1=w1333:dbl)
                    n1423 = local read "time (s)"() -> (w1336:dbl)
                    n1424 = local read "mistake # 1.2R"() -> (w1326:dbl)
                    n1425 = local read "trial #"() -> (w1330:dbl)
                    n1426 = local read "ITI (s)"() -> (w1328:dbl)
                    n1427 = local write "lick # 1.2R"(w1333) -> ()
                    n1428 = local write "state 1.1"(enum16{"waiting", "sound", "ITI"}."ITI") -> ()
                    n1429 = Increment(x=w1325) -> (x+1=w1324:dbl)
                    n1430 = local read "Mouse path 1"() -> (w1339:path)
                    n1431 = local write "mistake # 1.1L"(w1324) -> ()
                    n1432 = Build Array(w1336, w1335, w1333, w1332, w1331, w1327, w1327, w1330, w1329, w1328, w1327, w1324, w1326) -> (w1338:dbl[])
                    n1433 = call-poly <vilib>:"Write To Spreadsheet File.vi"("append to file? (new file:F)"=TRUE, "1D data"=w1338, "file path (dialog if empty)"=w1339) -> ()  [unwired: 5 in, 1 out]
                    n1434 = local write "state 1.2"(enum16{"waiting", "sound", "ITI"}."ITI") -> ()
                  }
                  frame "sound" {
                    w1343 = 0 ("element")
                    n1435 = local read "water # 1.2R"() -> (w1347:dbl)
                    n1436 = local read "water # 1.1L"() -> (w1348:dbl)
                    n1437 = local read "lick # 1.2R"() -> (w1350:dbl)
                    n1438 = local read "current sound"() -> (w1345:dbl)
                    n1439 = local read "mistake # 1.2R"() -> (w1341:dbl)
                    n1440 = local read "lick # 1.1L"() -> (w1351:dbl)
                    n1441 = local read "ITI (s)"() -> (w1344:dbl)
                    n1442 = local read "mistake # 1.1L"() -> (w1342:dbl)
                    n1443 = local read "trial #"() -> (w1346:dbl)
                    n1444 = Increment(x=w1350) -> (x+1=w1349:dbl)
                    n1445 = local read "time (s)"() -> (w1352:dbl)
                    n1446 = local write "lick # 1.2R"(w1349) -> ()
                    n1447 = local read "Mouse path 1"() -> (w1354:path)
                    n1448 = Build Array(w1352, w1351, w1349, w1348, w1347, w1343, w1343, w1346, w1345, w1344, w1343, w1342, w1341) -> (w1353:dbl[])
                    n1449 = call-poly <vilib>:"Write To Spreadsheet File.vi"("append to file? (new file:F)"=TRUE, "1D data"=w1353, "file path (dialog if empty)"=w1354) -> ()  [unwired: 5 in, 1 out]
                  }
                  frame "ITI" {
                    w1358 = 0 ("element")
                    n1450 = local read "water # 1.2R"() -> (w1362:dbl)
                    n1451 = local read "water # 1.1L"() -> (w1363:dbl)
                    n1452 = local read "lick # 1.2R"() -> (w1365:dbl)
                    n1453 = local read "current sound"() -> (w1360:dbl)
                    n1454 = local read "lick # 1.1L"() -> (w1366:dbl)
                    n1455 = local read "mistake # 1.2R"() -> (w1356:dbl)
                    n1456 = local read "mistake # 1.1L"() -> (w1357:dbl)
                    n1457 = local read "trial #"() -> (w1361:dbl)
                    n1458 = local read "ITI (s)"() -> (w1359:dbl)
                    n1459 = local read "time (s)"() -> (w1367:dbl)
                    n1460 = Increment(x=w1365) -> (x+1=w1364:dbl)
                    n1461 = local write "lick # 1.2R"(w1364) -> ()
                    n1462 = local read "Mouse path 1"() -> (w1370:path)
                    n1463 = Build Array(w1367, w1366, w1364, w1363, w1362, w1358, w1358, w1361, w1360, w1359, w1358, w1357, w1356) -> (w1368:dbl[])
                    n1464 = call-poly <vilib>:"Write To Spreadsheet File.vi"("append to file? (new file:F)"=TRUE, "1D data"=w1368, "file path (dialog if empty)"=w1370) -> ()  [unwired: 5 in, 1 out]
                  }
                }
              }
            }
          }
          frame 4 {
            n1465 = case shown="True" w1425 {
              frame False {
              }
              frame True {
                n1466 = local read "state 1.2"() -> (w1479:enum16{"waiting", "sound", "ITI"})
                n1467 = case shown="\"sound\"" w1479 {
                  frame "waiting", Default {
                    w1487 = 0 ("element")
                    n1468 = local read "water # 1.1L"() -> (w1489:dbl)
                    n1469 = local read "lick # 1.2R"() -> (w1490:dbl)
                    n1470 = local read "lick # 1.1L"() -> (w1492:dbl)
                    n1471 = local read "water # 1.2R"() -> (w1488:dbl)
                    n1472 = local read "mistake # 1.2R"() -> (w1482:dbl)
                    n1473 = local read "mistake # 1.1L"() -> (w1483:dbl)
                    n1474 = local read "current sound"() -> (w1485:dbl)
                    n1475 = local read "time (s)"() -> (w1493:dbl)
                    n1476 = Increment(x=w1492) -> (x+1=w1491:dbl)
                    n1477 = local read "trial #"() -> (w1486:dbl)
                    n1478 = local read "ITI (s)"() -> (w1484:dbl)
                    n1479 = local write "state 1.2"(enum16{"waiting", "sound", "ITI"}."ITI") -> ()
                    n1480 = local write "state 1.1"(enum16{"waiting", "sound", "ITI"}."ITI") -> ()
                    n1481 = local write "lick # 1.1L"(w1491) -> ()
                    n1482 = Increment(x=w1482) -> (x+1=w1481:dbl)
                    n1483 = local write "mistake # 1.2R"(w1481) -> ()
                    n1484 = local read "Mouse path 1"() -> (w1496:path)
                    n1485 = Build Array(w1493, w1491, w1490, w1489, w1488, w1487, w1487, w1486, w1485, w1484, w1483, w1481) -> (w1494:dbl[])
                    n1486 = call-poly <vilib>:"Write To Spreadsheet File.vi"("append to file? (new file:F)"=TRUE, "1D data"=w1494, "file path (dialog if empty)"=w1496) -> ()  [unwired: 5 in, 1 out]
                  }
                  frame "sound" {
                    w1500 = 0 ("element")
                    n1487 = local read "water # 1.2R"() -> (w1504:dbl)
                    n1488 = local read "water # 1.1L"() -> (w1505:dbl)
                    n1489 = local read "lick # 1.2R"() -> (w1506:dbl)
                    n1490 = local read "mistake # 1.2R"() -> (w1498:dbl)
                    n1491 = local read "current sound"() -> (w1502:dbl)
                    n1492 = local read "lick # 1.1L"() -> (w1508:dbl)
                    n1493 = local read "mistake # 1.1L"() -> (w1499:dbl)
                    n1494 = local read "trial #"() -> (w1503:dbl)
                    n1495 = local read "ITI (s)"() -> (w1501:dbl)
                    n1496 = local read "time (s)"() -> (w1509:dbl)
                    n1497 = Increment(x=w1508) -> (x+1=w1507:dbl)
                    n1498 = local read "Mouse path 1"() -> (w1512:path)
                    n1499 = local write "lick # 1.1L"(w1507) -> ()
                    n1500 = Build Array(w1509, w1507, w1506, w1505, w1504, w1500, w1500, w1503, w1502, w1501, w1500, w1499, w1498) -> (w1510:dbl[])
                    n1501 = call-poly <vilib>:"Write To Spreadsheet File.vi"("append to file? (new file:F)"=TRUE, "1D data"=w1510, "file path (dialog if empty)"=w1512) -> ()  [unwired: 5 in, 1 out]
                  }
                  frame "ITI" {
                    w1515 = 0 ("element")
                    n1502 = local read "water # 1.2R"() -> (w1519:dbl)
                    n1503 = local read "lick # 1.1L"() -> (w1523:dbl)
                    n1504 = local read "water # 1.1L"() -> (w1520:dbl)
                    n1505 = local read "lick # 1.2R"() -> (w1521:dbl)
                    n1506 = local read "mistake # 1.2R"() -> (w1513:dbl)
                    n1507 = local read "current sound"() -> (w1517:dbl)
                    n1508 = local read "mistake # 1.1L"() -> (w1514:dbl)
                    n1509 = Increment(x=w1523) -> (x+1=w1522:dbl)
                    n1510 = local read "trial #"() -> (w1518:dbl)
                    n1511 = local read "ITI (s)"() -> (w1516:dbl)
                    n1512 = local read "time (s)"() -> (w1524:dbl)
                    n1513 = local write "lick # 1.1L"(w1522) -> ()
                    n1514 = local read "Mouse path 1"() -> (w1527:path)
                    n1515 = Build Array(w1524, w1522, w1521, w1520, w1519, w1515, w1515, w1518, w1517, w1516, w1515, w1514, w1513) -> (w1525:dbl[])
                    n1516 = call-poly <vilib>:"Write To Spreadsheet File.vi"("append to file? (new file:F)"=TRUE, "1D data"=w1525, "file path (dialog if empty)"=w1527) -> ()  [unwired: 5 in, 1 out]
                  }
                }
              }
            }
            n1517 = case shown="True" w1424 {
              frame False {
              }
              frame True {
                n1518 = local read "state 1.2"() -> (w1426:enum16{"waiting", "sound", "ITI"})
                n1519 = case shown="\"waiting\", Default" w1426 {
                  frame "waiting", Default {
                    w1431 = 0 ("element")
                    n1520 = local read "water # 1.2R"() -> (w1437:dbl)
                    n1521 = local read "lick # 1.2R"() -> (w1440:dbl)
                    n1522 = local read "free water 1.2"() -> (w1427:bool)
                    n1523 = local read "water # 1.1L"() -> (w1438:dbl)
                    n1524 = local read "lick # 1.1L"() -> (w1441:dbl)
                    n1525 = local read "time (s)"() -> (w1442:dbl)
                    n1526 = local write "state 1.2"(enum16{"waiting", "sound", "ITI"}."ITI") -> ()
                    n1527 = local write "state 1.1"(enum16{"waiting", "sound", "ITI"}."ITI") -> ()
                    n1528 = Increment(x=w1437) -> (x+1=w1436:dbl)
                    n1529 = Increment(x=w1440) -> (x+1=w1439:dbl)
                    n1530 = case shown="False" w1427 {
                      frame False {
                        n1531 = local read "water dur (ms) 1.2"() -> (w1448:dbl)
                        n1532 = local read "water port 1.2"() -> (w1447:tag)
                        n1533 = call "_digital_on_duration_off.vi"("duration (ms)"=w1448, "digital port"=w1447) -> ()  [unwired: 10 in]
                      }
                      frame True {
                      }
                    }
                    n1534 = local write "water # 1.2R"(w1436) -> ()
                    n1535 = local write "lick # 1.2R"(w1439) -> ()
                    n1536 = local write "last water 1.2R"(w1442) -> ()
                    n1537 = local read "mistake # 1.2R"() -> (w1429:dbl)
                    n1538 = local read "mistake # 1.1L"() -> (w1430:dbl)
                    n1539 = local read "current sound"() -> (w1433:dbl)
                    n1540 = local read "ITI (s)"() -> (w1432:dbl)
                    n1541 = local read "trial #"() -> (w1434:dbl)
                    n1542 = local read "Mouse path 1"() -> (w1445:path)
                    n1543 = Build Array(w1442, w1441, w1439, w1438, w1436, 1 ("element"), w1431, w1434, w1433, w1432, w1431, w1430, w1429) -> (w1443:dbl[])
                    n1544 = call-poly <vilib>:"Write To Spreadsheet File.vi"("append to file? (new file:F)"=TRUE, "1D data"=w1443, "file path (dialog if empty)"=w1445) -> ()  [unwired: 5 in, 1 out]
                  }
                  frame "sound" {
                    w1451 = 0 ("element")
                    n1545 = local read "lick # 1.2R"() -> (w1458:dbl)
                    n1546 = local read "water # 1.2R"() -> (w1455:dbl)
                    n1547 = local read "water # 1.1L"() -> (w1456:dbl)
                    n1548 = local read "lick # 1.1L"() -> (w1459:dbl)
                    n1549 = local read "mistake # 1.2R"() -> (w1449:dbl)
                    n1550 = local read "current sound"() -> (w1453:dbl)
                    n1551 = Increment(x=w1458) -> (x+1=w1457:dbl)
                    n1552 = local read "mistake # 1.1L"() -> (w1450:dbl)
                    n1553 = local read "time (s)"() -> (w1460:dbl)
                    n1554 = local read "trial #"() -> (w1454:dbl)
                    n1555 = local read "ITI (s)"() -> (w1452:dbl)
                    n1556 = local write "lick # 1.2R"(w1457) -> ()
                    n1557 = local read "Mouse path 1"() -> (w1463:path)
                    n1558 = Build Array(w1460, w1459, w1457, w1456, w1455, w1451, w1451, w1454, w1453, w1452, w1451, w1450, w1449) -> (w1461:dbl[])
                    n1559 = call-poly <vilib>:"Write To Spreadsheet File.vi"("append to file? (new file:F)"=TRUE, "1D data"=w1461, "file path (dialog if empty)"=w1463) -> ()  [unwired: 5 in, 1 out]
                  }
                  frame "ITI" {
                    w1466 = 0 ("element")
                    n1560 = local read "water # 1.2R"() -> (w1470:dbl)
                    n1561 = local read "water # 1.1L"() -> (w1471:dbl)
                    n1562 = local read "lick # 1.2R"() -> (w1473:dbl)
                    n1563 = local read "lick # 1.1L"() -> (w1474:dbl)
                    n1564 = local read "mistake # 1.2R"() -> (w1464:dbl)
                    n1565 = local read "current sound"() -> (w1468:dbl)
                    n1566 = local read "mistake # 1.1L"() -> (w1465:dbl)
                    n1567 = Increment(x=w1473) -> (x+1=w1472:dbl)
                    n1568 = local read "ITI (s)"() -> (w1467:dbl)
                    n1569 = local read "trial #"() -> (w1469:dbl)
                    n1570 = local read "time (s)"() -> (w1475:dbl)
                    n1571 = local write "lick # 1.2R"(w1472) -> ()
                    n1572 = local read "Mouse path 1"() -> (w1478:path)
                    n1573 = Build Array(w1475, w1474, w1472, w1471, w1470, w1466, w1466, w1469, w1468, w1467, w1466, w1465, w1464) -> (w1476:dbl[])
                    n1574 = call-poly <vilib>:"Write To Spreadsheet File.vi"("append to file? (new file:F)"=TRUE, "1D data"=w1476, "file path (dialog if empty)"=w1478) -> ()  [unwired: 5 in, 1 out]
                  }
                }
              }
            }
          }
        }
        n1575 = call "_loop_time.vi"("from shift register"=w83) -> ("to shift register"=w82:dbl)  [unwired: 9 in, 1 out]
        n1576 = call "Elapsed Time"() -> ("Elapsed Time (s)"=→"time (s)":dbl)  [unwired: 12 in, 7 out]
      }
      n1577 = call <vilib>:"DAQmx Clear Task.vi"("task in"=w29) -> ()  [unwired: 14 in, 1 out]
      n1578 = while {
        shift-right: [w1531] -> _
        shift-left: T1."prepare" -> [w1530]
        stop <- FALSE stop-if-true
        n1579 = local write "trial state"(w1530) -> ()
        n1580 = case shown="\"ITI\"" w1530 {
          tunnel: [w1532 w1561 w1590 w1593 w1599 T1."ITI" T1."prepare"] -> w1531
          frame "prepare", Default {
            n1581 = flat-sequence {
              tunnel: [T1."sound"] -> w1532
              frame #0 {
                w1536 = 500
                w1543 = 1000
                n1582 = Subtract(x="ITI max (ms)", y=w1536) -> (x-y=w1539:dbl)
                n1583 = Subtract(x="ITI min (ms)", y=w1536) -> (x-y=w1540:dbl)
                n1584 = local read "next sound"() -> (w1546:dbl[])
                n1585 = Divide(x=w1539, y=w1543) -> (x/y=w1534:dbl)
                n1586 = Divide(x=w1540, y=w1543) -> (x/y=w1533:dbl)
                n1587 = Delete From Array(array=w1546, index=0) -> (deleted portion=w1544:dbl, array with subset deleted=w1545:dbl[])  [unwired: 1 in]
                n1588 = local write "next sound"(w1545) -> ()
                n1589 = call "_random_integer.vi"("max"=w1534, "min"=w1533) -> ("output"=w1537:dbl)  [unwired: 9 in]
                n1590 = local write "current sound"(w1544) -> ()
                n1591 = Add(x=w1537, y=0.5) -> (x+y=w1538:dbl)
                n1592 = local write "ITI (s)"(w1538) -> ()
              }
              frame #1 {
                w1548 = 0
                n1593 = local read "current sound"() -> (w1552:dbl)
                n1594 = local read "time (s)"() -> (w1555:dbl)
                n1595 = local read "trial #"() -> (w1558:dbl)
                n1596 = local read "ITI (s)"() -> (w1551:dbl)
                n1597 = Increment(x=w1558) -> (x+1=w1553:dbl)
                n1598 = local read "Mouse path 1"() -> (w1557:path)
                n1599 = local write "trial #"(w1553) -> ()
                n1600 = Build Array(w1555, w1548, w1548, w1548, w1548, w1548, 1, w1553, w1552, w1551, 0, w1548, w1548) -> (w1549:dbl[])
                n1601 = call-poly <vilib>:"Write To Spreadsheet File.vi"("append to file? (new file:F)"=TRUE, "1D data"=w1549, "file path (dialog if empty)"=w1557) -> ()  [unwired: 5 in, 1 out]
              }
              frame #2 {
                w1559 = enum16{"waiting", "sound", "ITI"}."sound"
                n1602 = local write "state 1.2"(w1559) -> ()
                n1603 = local write "state 1.1"(w1559) -> ()
                n1604 = local write "state 3.2"(w1559) -> ()
                n1605 = local write "state 3.1"(w1559) -> ()
                n1606 = local write "state 4.2"(w1559) -> ()
                n1607 = local write "state 2.1"(w1559) -> ()
                n1608 = local write "state 2.2"(w1559) -> ()
                n1609 = local write "state 4.1"(w1559) -> ()
              }
              frame #3 {
              }
            }
          }
          frame "sound" {
            n1610 = flat-sequence {
              tunnel: [T1."free water"] -> w1561
              frame #0 {
                n1611 = local read "current sound"() -> (w1567:dbl)
                n1612 = case shown="3" w1567 {
                  tunnel: "sound dur (ms)" -> [w1572 w1577 w1582 w1586]
                  tunnel: "sound port 1" -> [w1569 _ w1579 _]
                  tunnel: "sound port 2" -> [_ w1574 _ w1587]
                  tunnel: "sound file 1" -> [w1568 _ _ w1583]
                  tunnel: "sound file 2" -> [_ w1573 w1578 _]
                  frame ..1 {
                    n1613 = local read "Left Speaker"() -> (w1571:dbl)
                    n1614 = Increment(x=w1571) -> (x+1=w1570:dbl)
                    n1615 = local write "Left Speaker"(w1570) -> ()
                    n1616 = call "_play_wave_file.vi"("sound length (ms)"=w1572, "sound file"=w1568, "sound port"=w1569) -> ()  [unwired: 9 in]
                  }
                  frame 2 {
                    n1617 = local read "Right Speaker"() -> (w1576:dbl)
                    n1618 = Increment(x=w1576) -> (x+1=w1575:dbl)
                    n1619 = call "_play_wave_file.vi"("sound length (ms)"=w1577, "sound file"=w1573, "sound port"=w1574) -> ()  [unwired: 9 in]
                    n1620 = local write "Right Speaker"(w1575) -> ()
                  }
                  frame 3 {
                    n1621 = local read "Left Speaker"() -> (w1581:dbl)
                    n1622 = call "_play_wave_file.vi"("sound length (ms)"=w1582, "sound file"=w1578, "sound port"=w1579) -> ()  [unwired: 9 in]
                    n1623 = Increment(x=w1581) -> (x+1=w1580:dbl)
                    n1624 = local write "Left Speaker"(w1580) -> ()
                  }
                  frame 4.. {
                    n1625 = local read "Right Speaker"() -> (w1585:dbl)
                    n1626 = Increment(x=w1585) -> (x+1=w1584:dbl)
                    n1627 = call "_play_wave_file.vi"("sound length (ms)"=w1586, "sound file"=w1583, "sound port"=w1587) -> ()  [unwired: 9 in]
                    n1628 = local write "Right Speaker"(w1584) -> ()
                  }
                }
              }
              frame #1 {
                w1588 = enum16{"waiting", "sound", "ITI"}."waiting"
                n1629 = local write "state 1.1"(w1588) -> ()
                n1630 = local write "state 1.2"(w1588) -> ()
                n1631 = local write "state 2.1"(w1588) -> ()
                n1632 = local write "state 2.2"(w1588) -> ()
                n1633 = local write "state 3.2"(w1588) -> ()
                n1634 = local write "state 3.1"(w1588) -> ()
                n1635 = local write "state 4.1"(w1588) -> ()
                n1636 = local write "state 4.2"(w1588) -> ()
              }
              frame #2 {
              }
            }
          }
          frame "reaction window" {
            n1637 = flat-sequence {
              tunnel: [T1."graph"] -> w1590
              frame #0 {
                n1638 = Wait (ms)(milliseconds to wait="reaction dur (ms)") -> ()  [unwired: 1 out]
              }
              frame #1 {
              }
            }
          }
          frame "ITI" {
            n1639 = flat-sequence {
              tunnel: [T1."prepare"] -> w1593
              frame #0 {
                w1594 = enum16{"waiting", "sound", "ITI"}."ITI"
                n1640 = local write "state 1.1"(w1594) -> ()
                n1641 = local write "state 1.2"(w1594) -> ()
                n1642 = local write "state 2.2"(w1594) -> ()
                n1643 = local write "state 3.1"(w1594) -> ()
                n1644 = local write "state 2.1"(w1594) -> ()
                n1645 = local write "state 3.2"(w1594) -> ()
                n1646 = local write "state 4.1"(w1594) -> ()
                n1647 = local write "state 4.2"(w1594) -> ()
              }
              frame #1 {
                n1648 = local read "ITI (s)"() -> (w1597:dbl)
                n1649 = Multiply(x=w1597, y=1000) -> (x*y=w1595:dbl)
                n1650 = Wait (ms)(milliseconds to wait=w1595) -> ()  [unwired: 1 out]
              }
              frame #2 {
              }
            }
          }
          frame "free water" {
            n1651 = flat-sequence {
              tunnel: [T1."reaction window"] -> w1599
              frame #0 {
                n1652 = local read "state 4.2"() -> (w1603:enum16{"waiting", "sound", "ITI"})
                n1653 = local read "state 4.1"() -> (w1604:enum16{"waiting", "sound", "ITI"})
                n1654 = local read "state 1.1"() -> (w1628:enum16{"waiting", "sound", "ITI"})
                n1655 = local read "state 1.2"() -> (w1627:enum16{"waiting", "sound", "ITI"})
                n1656 = local read "state 2.1"() -> (w1615:enum16{"waiting", "sound", "ITI"})
                n1657 = local read "state 2.2"() -> (w1614:enum16{"waiting", "sound", "ITI"})
                n1658 = local read "state 3.1"() -> (w1611:enum16{"waiting", "sound", "ITI"})
                n1659 = local read "state 3.2"() -> (w1610:enum16{"waiting", "sound", "ITI"})
                n1660 = Build Array(w1628, w1627, w1615, w1614, w1611, w1610, w1604, w1603) -> (w1626:enum16{"waiting", "sound", "ITI"}[])
                n1661 = local write "free water 1.1"("free water 1.1") -> ()
                n1662 = local write "free water 1.2"("free water 1.2") -> ()
                n1663 = local write "free water 2.1"("free water 2.1") -> ()
                n1664 = local write "free water 3.1"("free water 3.1") -> ()
                n1665 = local write "free water 2.2"("free water 2.2") -> ()
                n1666 = local write "free water 3.2"("free water 3.2") -> ()
                n1667 = local write "free water 4.2"("free water 4.2") -> ()
                n1668 = local write "free water 4.1"("free water 4.1") -> ()
                n1669 = Build Array("free water 1.1", "free water 1.2", "free water 2.1", "free water 2.2", "free water 3.1", "free water 3.2", "free water 4.1", "free water 4.2") -> (w1630:bool[])
                n1670 = Equal?(x=w1626, y=enum16{"waiting", "water", "ITI"}."waiting") -> (x = y?=w1631:bool[])
                n1671 = And(x=w1631, y=w1630) -> (x .and. y?=w1629:bool[])
                n1672 = Index Array(array=w1629) -> (element #1=w1624:bool, element #2=w1621:bool, element #3=w1617:bool, element #4=w1616:bool, element #5=w1608:bool, element #6=w1607:bool, element #7=w1601:bool, element #8=w1600:bool)  [unwired: 8 in]
                n1673 = local read "current sound"() -> (w1625:dbl)
                n1674 = local read "current sound"() -> (w1618:dbl)
                n1675 = local read "current sound"() -> (w1602:dbl)
                n1676 = local read "current sound"() -> (w1609:dbl)
                n1677 = case shown="1" w1625 {
                  tunnel: w1624 -> [_ w1669 _ w1693 _]
                  tunnel: w1621 -> [_ _ w1681 _ w1696]
                  frame 0, Default {
                  }
                  frame 1 {
                    n1678 = case shown="True" w1669 {
                      frame False {
                      }
                      frame True {
                        w1670 = 0
                        n1679 = local read "water port 1.1"() -> (w1672:tag)
                        n1680 = local read "water dur (ms) 1.1"() -> (w1671:dbl)
                        n1681 = local read "current sound"() -> (w1676:dbl)
                        n1682 = local read "trial #"() -> (w1677:dbl)
                        n1683 = local read "ITI (s)"() -> (w1675:dbl)
                        n1684 = local read "time (s)"() -> (w1678:dbl)
                        n1685 = call "_digital_on_duration_off.vi"("duration (ms)"=w1671, "digital port"=w1672) -> ()  [unwired: 10 in]
                        n1686 = local read "Mouse path 1"() -> (w1679:path)
                        n1687 = Build Array(w1678, w1670, w1670, w1670, w1670, w1670, w1670, w1677, w1676, w1675, 1, w1670, w1670) -> (w1673:dbl[])
                        n1688 = call-poly <vilib>:"Write To Spreadsheet File.vi"("append to file? (new file:F)"=TRUE, "1D data"=w1673, "file path (dialog if empty)"=w1679) -> ()  [unwired: 5 in, 1 out]
                      }
                    }
                  }
                  frame 2 {
                    n1689 = case shown="True" w1681 {
                      frame False {
                      }
                      frame True {
                        w1684 = 0 ("element")
                        n1690 = local read "water dur (ms) 1.2"() -> (w1682:dbl)
                        n1691 = local read "current sound"() -> (w1687:dbl)
                        n1692 = local read "water port 1.2"() -> (w1683:tag)
                        n1693 = local read "trial #"() -> (w1688:dbl)
                        n1694 = local read "ITI (s)"() -> (w1686:dbl)
                        n1695 = local read "time (s)"() -> (w1689:dbl)
                        n1696 = call "_digital_on_duration_off.vi"("duration (ms)"=w1682, "digital port"=w1683) -> ()  [unwired: 10 in]
                        n1697 = local read "Mouse path 1"() -> (w1691:path)
                        n1698 = Build Array(w1689, w1684, w1684, w1684, w1684, w1684, w1684, w1688, w1687, w1686, 1 ("element"), w1684, w1684) -> (w1690:dbl[])
                        n1699 = call-poly <vilib>:"Write To Spreadsheet File.vi"("append to file? (new file:F)"=TRUE, "1D data"=w1690, "file path (dialog if empty)"=w1691) -> ()  [unwired: 5 in, 1 out]
                      }
                    }
                  }
                  frame 3 {
                    n1700 = case shown="True" w1693 {
                      frame False {
                      }
                      frame True {
                        n1701 = local read "water dur (ms) 1.1"() -> (w1694:dbl)
                        n1702 = local read "water port 1.1"() -> (w1695:tag)
                        n1703 = call "_digital_on_duration_off.vi"("duration (ms)"=w1694, "digital port"=w1695) -> ()  [unwired: 10 in]
                      }
                    }
                  }
                  frame 4 {
                    n1704 = case shown="True" w1696 {
                      frame False {
                      }
                      frame True {
                        n1705 = local read "water dur (ms) 1.2"() -> (w1697:dbl)
                        n1706 = local read "water port 1.2"() -> (w1698:tag)
                        n1707 = call "_digital_on_duration_off.vi"("duration (ms)"=w1697, "digital port"=w1698) -> ()  [unwired: 10 in]
                      }
                    }
                  }
                }
                n1708 = case shown="1" w1609 {
                  tunnel: w1608 -> [_ w1645 _ w1651 _]
                  tunnel: w1607 -> [_ _ w1648 _ w1654]
                  frame 0, Default {
                  }
                  frame 1 {
                    n1709 = case shown="True" w1645 {
                      frame False {
                      }
                      frame True {
                        n1710 = local read "water dur (ms) 3.1"() -> (w1646:dbl)
                        n1711 = local read "water port 3.1"() -> (w1647:tag)
                        n1712 = call "_digital_on_duration_off.vi"("duration (ms)"=w1646, "digital port"=w1647) -> ()  [unwired: 10 in]
                      }
                    }
                  }
                  frame 2 {
                    n1713 = case shown="True" w1648 {
                      frame False {
                      }
                      frame True {
                        n1714 = local read "water dur (ms) 3. 2"() -> (w1649:dbl)
                        n1715 = local read "water port 3.2"() -> (w1650:tag)
                        n1716 = call "_digital_on_duration_off.vi"("duration (ms)"=w1649, "digital port"=w1650) -> ()  [unwired: 10 in]
                      }
                    }
                  }
                  frame 3 {
                    n1717 = case shown="True" w1651 {
                      frame False {
                      }
                      frame True {
                        n1718 = local read "water dur (ms) 3.1"() -> (w1652:dbl)
                        n1719 = local read "water port 3.1"() -> (w1653:tag)
                        n1720 = call "_digital_on_duration_off.vi"("duration (ms)"=w1652, "digital port"=w1653) -> ()  [unwired: 10 in]
                      }
                    }
                  }
                  frame 4 {
                    n1721 = case shown="True" w1654 {
                      frame False {
                      }
                      frame True {
                        n1722 = local read "water dur (ms) 3. 2"() -> (w1655:dbl)
                        n1723 = local read "water port 3.2"() -> (w1656:tag)
                        n1724 = call "_digital_on_duration_off.vi"("duration (ms)"=w1655, "digital port"=w1656) -> ()  [unwired: 10 in]
                      }
                    }
                  }
                }
                n1725 = case shown="1" w1618 {
                  tunnel: w1617 -> [_ w1657 _ w1663 _]
                  tunnel: w1616 -> [_ _ w1660 _ w1666]
                  frame 0, Default {
                  }
                  frame 1 {
                    n1726 = case shown="True" w1657 {
                      frame False {
                      }
                      frame True {
                        n1727 = local read "water dur (ms) 2.1"() -> (w1658:dbl)
                        n1728 = local read "water port 2.1"() -> (w1659:tag)
                        n1729 = call "_digital_on_duration_off.vi"("duration (ms)"=w1658, "digital port"=w1659) -> ()  [unwired: 10 in]
                      }
                    }
                  }
                  frame 2 {
                    n1730 = case shown="True" w1660 {
                      frame False {
                      }
                      frame True {
                        n1731 = local read "water dur (ms) 2.2"() -> (w1661:dbl)
                        n1732 = local read "water port 2.2"() -> (w1662:tag)
                        n1733 = call "_digital_on_duration_off.vi"("duration (ms)"=w1661, "digital port"=w1662) -> ()  [unwired: 10 in]
                      }
                    }
                  }
                  frame 3 {
                    n1734 = case shown="True" w1663 {
                      frame False {
                      }
                      frame True {
                        n1735 = local read "water dur (ms) 2.1"() -> (w1664:dbl)
                        n1736 = local read "water port 2.1"() -> (w1665:tag)
                        n1737 = call "_digital_on_duration_off.vi"("duration (ms)"=w1664, "digital port"=w1665) -> ()  [unwired: 10 in]
                      }
                    }
                  }
                  frame 4 {
                    n1738 = case shown="True" w1666 {
                      frame False {
                      }
                      frame True {
                        n1739 = local read "water dur (ms) 2.2"() -> (w1667:dbl)
                        n1740 = local read "water port 2.2"() -> (w1668:tag)
                        n1741 = call "_digital_on_duration_off.vi"("duration (ms)"=w1667, "digital port"=w1668) -> ()  [unwired: 10 in]
                      }
                    }
                  }
                }
                n1742 = case shown="4" w1602 {
                  tunnel: w1601 -> [_ w1633 _ w1639 _]
                  tunnel: w1600 -> [_ _ w1636 _ w1642]
                  frame 0, Default {
                  }
                  frame 1 {
                    n1743 = case shown="True" w1633 {
                      frame False {
                      }
                      frame True {
                        n1744 = local read "water dur (ms) 4.1"() -> (w1634:dbl)
                        n1745 = local read "water port 4.1"() -> (w1635:tag)
                        n1746 = call "_digital_on_duration_off.vi"("duration (ms)"=w1634, "digital port"=w1635) -> ()  [unwired: 10 in]
                      }
                    }
                  }
                  frame 2 {
                    n1747 = case shown="True" w1636 {
                      frame False {
                      }
                      frame True {
                        n1748 = local read "water dur (ms) 4.2"() -> (w1637:dbl)
                        n1749 = local read "water port 4.2"() -> (w1638:tag)
                        n1750 = call "_digital_on_duration_off.vi"("duration (ms)"=w1637, "digital port"=w1638) -> ()  [unwired: 10 in]
                      }
                    }
                  }
                  frame 3 {
                    n1751 = case shown="True" w1639 {
                      frame False {
                      }
                      frame True {
                        n1752 = local read "water dur (ms) 4.1"() -> (w1640:dbl)
                        n1753 = local read "water port 4.1"() -> (w1641:tag)
                        n1754 = call "_digital_on_duration_off.vi"("duration (ms)"=w1640, "digital port"=w1641) -> ()  [unwired: 10 in]
                      }
                    }
                  }
                  frame 4 {
                    n1755 = case shown="True" w1642 {
                      frame False {
                      }
                      frame True {
                        n1756 = local read "water dur (ms) 4.2"() -> (w1643:dbl)
                        n1757 = local read "water port 4.2"() -> (w1644:tag)
                        n1758 = call "_digital_on_duration_off.vi"("duration (ms)"=w1643, "digital port"=w1644) -> ()  [unwired: 10 in]
                      }
                    }
                  }
                }
              }
              frame #1 {
              }
            }
          }
          frame "graph" {
            n1759 = local read "mistake # 2.2R"() -> (w1734:dbl)
            n1760 = local read "mistake # 3.1L"() -> (w1726:dbl)
            n1761 = local read "mistake # 4.2R"() -> (w1702:dbl)
            n1762 = local read "mistake # 4.1L"() -> (w1710:dbl)
            n1763 = local read "water # 4.2R"() -> (w1703:dbl)
            n1764 = local read "water # 2.2R"() -> (w1735:dbl)
            n1765 = local read "water # 4.2R"() -> (w1704:dbl)
            n1766 = local read "mistake # 2.1L"() -> (w1742:dbl)
            n1767 = local read "water # 3.1L"() -> (w1727:dbl)
            n1768 = local read "water # 2.2R"() -> (w1736:dbl)
            n1769 = local read "water # 4.1L"() -> (w1711:dbl)
            n1770 = local read "water # 2.1L"() -> (w1743:dbl)
            n1771 = local read "water # 3.1L"() -> (w1729:dbl)
            n1772 = local read "mistake # 3.2R"() -> (w1718:dbl)
            n1773 = local read "mistake # 1.2R"() -> (w1751:dbl)
            n1774 = local read "water # 3.2R"() -> (w1719:dbl)
            n1775 = local read "water # 2.1L"() -> (w1744:dbl)
            n1776 = local read "water # 4.1L"() -> (w1713:dbl)
            n1777 = local read "mistake # 1.1L"() -> (w1758:dbl)
            n1778 = local read "water # 3.2R"() -> (w1721:dbl)
            n1779 = local read "water # 1.1L"() -> (w1759:dbl)
            n1780 = local read "water # 1.2R"() -> (w1752:dbl)
            n1781 = local read "water # 1.2R"() -> (w1753:dbl)
            n1782 = local read "water # 1.1L"() -> (w1761:dbl)
            n1783 = Add(x=w1703, y=w1702) -> (x+y=w1701:dbl)
            n1784 = Add(x=w1735, y=w1734) -> (x+y=w1733:dbl)
            n1785 = Add(x=w1743, y=w1742) -> (x+y=w1741:dbl)
            n1786 = Add(x=w1727, y=w1726) -> (x+y=w1725:dbl)
            n1787 = Add(x=w1759, y=w1758) -> (x+y=w1757:dbl)
            n1788 = Add(x=w1719, y=w1718) -> (x+y=w1717:dbl)
            n1789 = Add(x=w1752, y=w1751) -> (x+y=w1750:dbl)
            n1790 = Add(x=w1711, y=w1710) -> (x+y=w1709:dbl)
            n1791 = Divide(x=w1744, y=w1741) -> (x/y=w1745:dbl)
            n1792 = Divide(x=w1721, y=w1717) -> (x/y=w1720:dbl)
            n1793 = Divide(x=w1729, y=w1725) -> (x/y=w1728:dbl)
            n1794 = Divide(x=w1736, y=w1733) -> (x/y=w1737:dbl)
            n1795 = Divide(x=w1753, y=w1750) -> (x/y=w1749:dbl)
            n1796 = Divide(x=w1761, y=w1757) -> (x/y=w1760:dbl)
            n1797 = Divide(x=w1704, y=w1701) -> (x/y=w1705:dbl)
            n1798 = Divide(x=w1713, y=w1709) -> (x/y=w1712:dbl)
            n1799 = local read "time (s)"() -> (w1765:dbl)
            n1800 = call <vilib>:"Mean PtByPt.vi"("x"=w1728) -> ("mean"=w1730:dbl)  [unwired: 3 in, 1 out]
            n1801 = call <vilib>:"Mean PtByPt.vi"("x"=w1720) -> ("mean"=w1722:dbl)  [unwired: 3 in, 1 out]
            n1802 = call <vilib>:"Mean PtByPt.vi"("x"=w1749) -> ("mean"=w1754:dbl)  [unwired: 3 in, 1 out]
            n1803 = call <vilib>:"Mean PtByPt.vi"("x"=w1712) -> ("mean"=w1714:dbl)  [unwired: 3 in, 1 out]
            n1804 = call <vilib>:"Mean PtByPt.vi"("x"=w1705) -> ("mean"=w1700:dbl)  [unwired: 3 in, 1 out]
            n1805 = call <vilib>:"Mean PtByPt.vi"("x"=w1745) -> ("mean"=w1746:dbl)  [unwired: 3 in, 1 out]
            n1806 = call <vilib>:"Mean PtByPt.vi"("x"=w1737) -> ("mean"=w1738:dbl)  [unwired: 3 in, 1 out]
            n1807 = call <vilib>:"Mean PtByPt.vi"("x"=w1760) -> ("mean"=w1762:dbl)  [unwired: 3 in, 1 out]
            n1808 = local write "ratio 1.2R"(w1754) -> ()
            n1809 = local write "ratio 1.1L"(w1762) -> ()
            n1810 = local write "ratio 2.1L"(w1746) -> ()
            n1811 = local write "ratio 3.1L"(w1730) -> ()
            n1812 = local write "ratio 2.2R"(w1738) -> ()
            n1813 = local write "ratio 3.2R"(w1722) -> ()
            n1814 = call "ratio"("Signals"=w1765) -> ("Collected Signals"=w1706:dynamicdata)  [unwired: 9 in, 1 out]
            n1815 = call "ratio1"("Signals"=w1762) -> ("Collected Signals"=w1764:dynamicdata)  [unwired: 9 in, 1 out]
            n1816 = local write "ratio 4.2R"(w1700) -> ()
            n1817 = call "ratio2"("Signals"=w1754) -> ("Collected Signals"=w1756:dynamicdata)  [unwired: 9 in, 1 out]
            n1818 = local write "ratio 4.1L"(w1714) -> ()
            n1819 = call "ratio3"("Signals"=w1746) -> ("Collected Signals"=w1748:dynamicdata)  [unwired: 9 in, 1 out]
            n1820 = call "ratio5"("Signals"=w1730) -> ("Collected Signals"=w1732:dynamicdata)  [unwired: 9 in, 1 out]
            n1821 = call "ratio4"("Signals"=w1738) -> ("Collected Signals"=w1740:dynamicdata)  [unwired: 9 in, 1 out]
            n1822 = call "ratio6"("Signals"=w1722) -> ("Collected Signals"=w1724:dynamicdata)  [unwired: 9 in, 1 out]
            n1823 = call "ratio7"("Signals"=w1714) -> ("Collected Signals"=w1716:dynamicdata)  [unwired: 9 in, 1 out]
            n1824 = call "ratio8"("Signals"=w1700) -> ("Collected Signals"=w1708:dynamicdata)  [unwired: 9 in, 1 out]
            n1825 = call "Build ratio1"("Y Input"=w1764, "X Input"=w1706) -> ("XY Graph"=→"ratio 1.1L":cluster{"Y":dbl[], "Y":dbl[]}[])  [unwired: 3 in, 6 out]
            n1826 = call "Build ratio"("Y Input"=w1756, "X Input"=w1706) -> ("XY Graph"=→"ratio 1.2R":cluster{"Y":dbl[], "Y":dbl[]}[])  [unwired: 3 in, 6 out]
            n1827 = call "Build ratio2"("Y Input"=w1748, "X Input"=w1706) -> ("XY Graph"=→"ratio 2.1L":cluster{"Y":dbl[], "Y":dbl[]}[])  [unwired: 3 in, 6 out]
            n1828 = call "Build ratio4"("Y Input"=w1732, "X Input"=w1706) -> ("XY Graph"=→"ratio 3.1L":cluster{"Y":dbl[], "Y":dbl[]}[])  [unwired: 3 in, 6 out]
            n1829 = call "Build ratio3"("Y Input"=w1740, "X Input"=w1706) -> ("XY Graph"=→"ratio 2.2R":cluster{"Y":dbl[], "Y":dbl[]}[])  [unwired: 3 in, 6 out]
            n1830 = call "Build ratio5"("Y Input"=w1724, "X Input"=w1706) -> ("XY Graph"=→"ratio 3.2R":cluster{"Y":dbl[], "Y":dbl[]}[])  [unwired: 3 in, 6 out]
            n1831 = call "Build ratio6"("Y Input"=w1716, "X Input"=w1706) -> ("XY Graph"=→"ratio 4.1L":cluster{"Y":dbl[], "Y":dbl[]}[])  [unwired: 3 in, 6 out]
            n1832 = call "Build ratio7"("Y Input"=w1708, "X Input"=w1706) -> ("XY Graph"=→"ratio 4.2R":cluster{"Y":dbl[], "Y":dbl[]}[])  [unwired: 3 in, 6 out]
          }
          frame "data collection" {
          }
        }
        n1833 = Wait (ms)(milliseconds to wait=u32 0) -> ()  [unwired: 1 out]
      }
    }
  }
